vi "main 1.17a beta.vi"() -> ()   [LabVIEW 2015]
uses:
  subvi/PHOIBOS/DEFINITIONS/DEF_dev_state.ctl
  subvi/PHOIBOS/DEFINITIONS/DEF_dev_type.ctl
  <vilib>/Analysis/_algsub.llb/Real Vector Norm.vi
  <vilib>/Analysis/1siggen.llb/Ramp Pattern by Samples.vi
  <vilib>/DAQmx/create/channels.llb/DAQmx Create Channel (DI-Digital Input).vi
  <userlib>/caLab/Private/Put_DBL_PV.vi
  <vilib>/Utility/file.llb/Write Delimited Spreadsheet (string).vi
  <vilib>/Utility/file.llb/Read Delimited Spreadsheet (string).vi
  <userlib>/caLab/Private/Get_PV.vi
  <vilib>/Utility/file.llb/Write Delimited Spreadsheet (DBL).vi
  subvi/Newport ESP301/Newport ESP301.lvlib
  subvi/sp_manip.llb/sp_manip_lib.lvlib
  subvi/sp_manip.llb/tcp_gateway.lvlib
  <vilib>/Analysis/NI_AALBase.lvlib
  <vilib>/Analysis/NI_AALPro.lvlib
  subvi/ZaberTSeries/ZaberTSeries.lvlib
panel:
  out "Pics L":i32=200
  out "Waveform Chart":dbl(graph)
  out "G2 X":cluster{dbl[], "Ramp Pattern":dbl[]}(graph)={array[344 elements], "Ramp Pattern"=[0.0, 0.0, 0.0, 0.0, 0.0, 0.0, 0.0, 0.0, 0.0, 0.0, 0.0, 0.0, 0.0, 0.0, 0.0, 0.0, 0.0, 0.0, 0.0, 0.0, 0.0, 12.377241379310345, 41.64689655172414, 18.335172413793103, 0.0, 0.0, 0.0, 0.0, 0.0, 0.0, 0.0, 0.0, 0.0, 0.0, 0.0, 0.0, 0.0, 0.0, 0.0, 0.0, 0.0, 0.0, 0.0, 0.0, 0.0, 0.0, 0.0, 0.0, 0.0, 0.0, 0.0, 0.0, 0.0, 0.0, 0.0, 0.0, 0.0, 0.0, 0.0, 0.0, 0.0, 0.0, 0.0, 0.0, 0.0, 0.0, 0.0, 0.0, 0.0, 0.0, 0.0, 0.0, 0.0, 0.0, 0.0, 0.0, 0.0, 0.0, 0.0, 0.0, 0.0, 0.0, 0.0, 0.0, 0.0, 0.0, 0.0, 0.0, 0.0, 0.0, 0.0, 0.0, 0.0, 0.0, 0.0, 0.0, 0.0, 0.0, 0.0, 0.0, 0.0, 0.0, 0.0, 0.0, 0.0, 0.0, 0.0, 0.0, 0.0, 0.0, 0.0, 0.0, 0.0, 0.0, 0.0, 17.495517241379314, 48.13413793103449, 27.429999999999996, 0.0, 0.0, 0.0, 0.0, 0.0, 0.0, 0.0, 0.0, 0.0, 0.0, 0.0, 0.0, 0.0, 0.0, 0.0, 0.0, 0.0, 0.0, 0.0, 0.0, 0.0, 0.0, 0.0, 0.0, 0.0, 0.0, 0.0, 0.0, 0.0, 0.0, 0.0, 0.0, 0.0, 0.0, 0.0, 0.0, 0.0, 0.0, 0.0, 0.0, 0.0, 0.0, 0.0, 0.0, 0.0, 0.0, 0.0, 0.0, 0.0, 0.0, 0.0, 0.0, 0.0, 0.0, 0.0, 0.0, 0.0, 0.0, 0.0, 0.0, 0.0, 0.0, 0.0, 0.0, 17.760344827586206, 28.923448275862068, 17.532068965517244, 0.0, 0.0, 0.0, 0.0, 0.0, 0.0, 0.0, 0.0, 0.0, 0.0, 0.0, 0.0, 0.0, 0.0, 0.0, 0.0, 0.0, 0.0, 0.0, 0.0, 0.0, 0.0, 0.0, 0.0, 0.0, 0.0, 0.0, 0.0, 0.0, 0.0, 0.0, 0.0, 0.0, 0.0, 0.0, 0.0, 0.0, 0.0, 0.0, 0.0, 0.0, 0.0, 0.0, 0.0, 0.0, 2.201724137931034, 1.9948275862068956, 0.0, 0.0, 0.0, 0.0, 0.0, 0.0, 0.0, 0.0, 0.0, 0.0, 0.0, 0.0, 0.0, 0.0, 0.0, 0.0, 0.0, 0.0, 0.0, 0.0, 0.0, 0.0, 0.0, 0.0, 0.0, 0.0, 0.0, 0.0, 0.0, 0.0, 0.0, 0.0, 0.0, 0.0, 0.0, 0.0, 0.0, 0.0, 0.0, 0.0, 0.0, 0.0, 0.0, 0.0, 0.0, 0.0, 0.0, 0.0, 0.0, 0.0, 0.0, 0.0, 0.0, 0.0, 0.0, 0.0, 0.0, 0.0, 0.0, 0.0, 0.0, 0.0, 0.0, 0.0, 0.0, 0.0, 0.0, 0.0, 0.0, 0.0, 0.0, 0.0, 0.0, 0.0, 0.0, 0.0, 0.0, 0.0, 0.0, 0.0, 0.0, 0.0, 0.0, 0.0, 0.0, 0.0, 0.0, 0.0, 0.0, 0.0, 0.0, 0.0, 0.0, 0.0, 0.0, 0.0, 0.0, 0.0, 0.0, 0.0, 0.0, 0.0, 0.0, 0.0, 0.0, 0.0, 0.0, 0.0, 0.0, 0.0, 0.0, 0.0]}
  in  "reset every n pics":bool=TRUE
  in  "pics2avg":i32=50
  in  "abort acq.":bool
  out "G2 Y":cluster{dbl[], "Ramp Pattern":dbl[]}(graph)={[0.0, 0.0, 0.0, 0.0, 0.0, 0.0, 0.0, 0.0, 0.0, 0.0, 0.0, 0.0, 0.0, 0.0, 0.0, 0.0, 0.0, 0.0, 0.0, 0.0, 0.0, 0.0, 0.0, 0.0, 0.0, 0.0, 0.0, 0.0, 0.0, 0.0, 0.0, 0.0, 0.0, 0.0, 0.0, 0.0, 0.0, 0.0, 0.0, 0.0, 0.0, 0.0, 0.0, 0.0, 0.0, 0.0, 0.0, 0.0, 0.0, 0.0, 0.0, 0.0, 0.0, 0.0, 0.0, 0.0, 0.0, 0.0, 0.0, 0.0, 0.0, 0.0, 0.0, 0.0, 0.0, 0.0, 0.0, 0.0, 0.0, 0.0, 0.0, 0.0, 0.0, 0.0, 0.0, 0.0, 0.0, 0.0, 0.0, 0.0, 0.0, 0.0, 0.0, 0.0, 0.0, 0.0, 0.0, 0.0, 0.0, 0.0, 0.0, 0.0, 0.0, 0.0, 0.0, 0.0, 0.0, 0.0, 0.0, 0.0, 0.0, 0.0, 0.0, 0.0, 0.0, 0.0, 0.0, 0.0, 0.0, 0.0, 0.0, 0.0, 0.0, 0.0, 0.0, 0.0, 0.0, 0.0, 0.0, 0.0, 0.0, 0.0, 0.0, 0.0, 0.0, 0.0, 0.0, 0.0, 0.0, 0.0, 0.0, 0.0, 0.0, 0.0, 0.0, 0.0, 0.0, 0.0, 0.0, 0.0, 0.0, 0.0, 0.0, 0.0, 0.0, 0.0, 0.0, 0.0, 0.0, 0.0, 0.0, 0.0, 0.0, 0.0, 0.0, 0.0, 0.0, 0.0, 0.0, 0.0, 0.0, 0.0, 0.0, 0.0, 0.0, 0.0, 0.0, 0.0, 0.0, 0.0, 0.0, 0.0, 0.0, 0.0, 0.0, 0.0, 0.0, 0.0, 0.0, 0.0, 0.0, 0.0, 0.0, 0.0, 0.0, 0.0, 0.0, 0.0, 0.0, 0.0, 0.0, 0.0, 0.0, 0.0, 0.0, 0.0, 0.0, 0.0, 0.0, 0.0, 0.0, 0.0, 0.0, 0.0, 0.0, 0.0, 0.0, 0.0, 0.0, 0.0, 0.0, 0.0, 0.0, 0.0, 0.0, 0.0, 0.0, 0.0, 0.0, 0.0, 0.0, 0.0, 0.0, 0.0, 0.0, 0.0, 0.0, 0.0, 0.0, 0.0, 0.0, 0.0, 0.0, 0.0, 0.0, 0.0, 0.0, 0.0, 0.0, 0.0, 0.0, 0.0, 0.0, 0.0, 0.0, 0.0, 0.0, 0.0, 0.0, 0.0, 0.0, 0.0, 0.0, 0.0, 0.0, 0.0], "Ramp Pattern"=[0.0, 1.003921568627451, 2.007843137254902, 3.011764705882353, 4.015686274509804, 5.019607843137255, 6.023529411764706, 7.027450980392157, 8.031372549019608, 9.035294117647059, 10.03921568627451, 11.04313725490196, 12.047058823529412, 13.050980392156863, 14.054901960784314, 15.058823529411764, 16.062745098039215, 17.066666666666666, 18.070588235294117, 19.07450980392157, 20.07843137254902, 21.08235294117647, 22.08627450980392, 23.090196078431372, 24.094117647058823, 25.098039215686274, 26.101960784313725, 27.105882352941176, 28.109803921568627, 29.113725490196078, 30.11764705882353, 31.12156862745098, 32.12549019607843, 33.129411764705885, 34.13333333333333, 35.13725490196079, 36.141176470588235, 37.14509803921569, 38.14901960784314, 39.15294117647059, 40.15686274509804, 41.16078431372549, 42.16470588235294, 43.168627450980395, 44.17254901960784, 45.1764705882353, 46.180392156862744, 47.1843137254902, 48.188235294117646, 49.1921568627451, 50.19607843137255, 51.2, 52.20392156862745, 53.207843137254905, 54.21176470588235, 55.21568627450981, 56.219607843137254, 57.22352941176471, 58.227450980392156, 59.23137254901961, 60.23529411764706, 61.23921568627451, 62.24313725490196, 63.247058823529414, 64.25098039215686, 65.25490196078431, 66.25882352941177, 67.26274509803922, 68.26666666666667, 69.27058823529411, 70.27450980392157, 71.27843137254902, 72.28235294117647, 73.28627450980392, 74.29019607843138, 75.29411764705883, 76.29803921568627, 77.30196078431372, 78.30588235294118, 79.30980392156863, 80.31372549019608, 81.31764705882352, 82.32156862745099, 83.32549019607843, 84.32941176470588, 85.33333333333333, 86.33725490196079, 87.34117647058824, 88.34509803921569, 89.34901960784313, 90.3529411764706, 91.35686274509804, 92.36078431372549, 93.36470588235294, 94.3686274509804, 95.37254901960785, 96.37647058823529, 97.38039215686274, 98.3843137254902, 99.38823529411765, 100.3921568627451, 101.39607843137254, 102.4, 103.40392156862745, 104.4078431372549, 105.41176470588235, 106.41568627450981, 107.41960784313726, 108.4235294117647, 109.42745098039215, 110.43137254901961, 111.43529411764706, 112.43921568627451, 113.44313725490196, 114.44705882352942, 115.45098039215686, 116.45490196078431, 117.45882352941176, 118.46274509803922, 119.46666666666667, 120.47058823529412, 121.47450980392156, 122.47843137254903, 123.48235294117647, 124.48627450980392, 125.49019607843137, 126.49411764705883, 127.49803921568628, 128.50196078431372, 129.50588235294117, 130.50980392156862, 131.51372549019607, 132.51764705882354, 133.521568627451, 134.52549019607844, 135.52941176470588, 136.53333333333333, 137.53725490196078, 138.54117647058823, 139.54509803921567, 140.54901960784315, 141.5529411764706, 142.55686274509804, 143.5607843137255, 144.56470588235294, 145.5686274509804, 146.57254901960783, 147.57647058823528, 148.58039215686276, 149.5843137254902, 150.58823529411765, 151.5921568627451, 152.59607843137255, 153.6, 154.60392156862744, 155.6078431372549, 156.61176470588236, 157.6156862745098, 158.61960784313726, 159.6235294117647, 160.62745098039215, 161.6313725490196, 162.63529411764705, 163.6392156862745, 164.64313725490197, 165.64705882352942, 166.65098039215687, 167.65490196078431, 168.65882352941176, 169.6627450980392, 170.66666666666666, 171.6705882352941, 172.67450980392158, 173.67843137254903, 174.68235294117648, 175.68627450980392, 176.69019607843137, 177.69411764705882, 178.69803921568626, 179.7019607843137, 180.7058823529412, 181.70980392156864, 182.71372549019608, 183.71764705882353, 184.72156862745098, 185.72549019607843, 186.72941176470587, 187.73333333333332, 188.7372549019608, 189.74117647058824, 190.7450980392157, 191.74901960784314, 192.75294117647059, 193.75686274509803, 194.76078431372548, 195.76470588235293, 196.7686274509804, 197.77254901960785, 198.7764705882353, 199.78039215686275, 200.7843137254902, 201.78823529411764, 202.7921568627451, 203.79607843137254, 204.8, 205.80392156862746, 206.8078431372549, 207.81176470588235, 208.8156862745098, 209.81960784313725, 210.8235294117647, 211.82745098039214, 212.83137254901962, 213.83529411764707, 214.8392156862745, 215.84313725490196, 216.8470588235294, 217.85098039215686, 218.8549019607843, 219.85882352941175, 220.86274509803923, 221.86666666666667, 222.87058823529412, 223.87450980392157, 224.87843137254902, 225.88235294117646, 226.8862745098039, 227.89019607843136, 228.89411764705883, 229.89803921568628, 230.90196078431373, 231.90588235294118, 232.90980392156862, 233.91372549019607, 234.91764705882352, 235.92156862745097, 236.92549019607844, 237.9294117647059, 238.93333333333334, 239.93725490196078, 240.94117647058823, 241.94509803921568, 242.94901960784313, 243.95294117647057, 244.95686274509805, 245.9607843137255, 246.96470588235294, 247.9686274509804, 248.97254901960784, 249.9764705882353, 250.98039215686273, 251.98431372549018, 252.98823529411766, 253.9921568627451, 254.99607843137255, 256.0]}
  out "ETA":timestamp=timestamp(3655133644.4615793 s since 1904-01-01) format="%<%H:%M:%S>T"
  out "acq. imgs":i32=200
  out "snap_prog":dbl(slide)=1.0 scale=0.0..1.0
  in  "BasePath":path=path "T:/trARPES/PESData"
  in  "cam_liveavg":bool=TRUE caption="live average"
  out "cam_fps":dbl=19.690658487387566 caption="FPS" format="%.1g"
  out "sideimg":dbl[][](graph)
  out "RunNumber":u16=3091
  out "sum":dbl format="%#.2g"
  out "max":dbl=22.774482758620692
  out "mainimg":dbl[][](graph)
  out "ESP_con?":bool=TRUE caption="ESP301"
  out "phoib_con?":bool caption="PHOIBOS"
  out "manip_con?":bool=TRUE caption="manipulator"
  out "cam_con?":bool caption="camera"
  in  "main_close":bool=TRUE
  in  "Tab Control":enum32{"live", "scan", "devices"}(tab)=enum."devices"
  in  "wattpilot_set":bool
  out "Readback_wattpilot":dbl=304.89
  in  "Set Powet (%)":dbl
  out "Readback":dbl=340.0
  out "In Range":bool
  in  "setpoint_set":bool
  in  "Setpoint":dbl=302.0
  out "TB":dbl=304.91
  out "TA":dbl=304.49
  in  "phoib_I_10s":dbl
  out "phoib_I_10":dbl caption="Mesh Back"
  in  "mirr_go":bool
  in  "ESP_opent0file":bool
  in  "mirr_rel":i32=1 caption="relative [steps]"
  in  "mirr_Y-":bool
  in  "mirr_Y+":bool
  in  "mirr_X+":bool
  in  "mirr_X-":bool
  in  "manip_deltas":dbl[](array[numeric])=[0.0, 0.0, 5.0, 0.0, 0.0, 0.0] caption="delta" format="%#.5g"
  in  "aq.mode":enum32{"Radio Selection 1", "Radio Selection 2"}(radio)=enum."Radio Selection 2"
  in  "dark avg":i32=100
  in  "cam_avgs":i32=20 caption="N"
  in  "ESP_delta":dbl caption="relative [mm]"
  in  "ESP_-":bool
  in  "ESP_+":bool
  in  "ESP_go":bool
  in  "ESP_dest_t":dbl=728236.1319443199 caption="[fs]"
  in  "ESP_dest":dbl=-35.84015 caption="[mm]"
  in  "ESP_set_t0":bool
  in  "phoib_I_6s":dbl=3200.0
  in  "phoib_I_5s":dbl=1500.0
  in  "phoib_I_4s":dbl=4.558
  in  "phoib_I_3s":dbl=-10.0
  in  "phoib_I_2s":dbl=35.0
  in  "phoib_I_1s":dbl=21.0
  in  "phoib_standby":bool
  in  "phoib_set":bool
  out "phoib_I_6":dbl=3200.0 caption="Screen Voltage"
  out "phoib_I_5":dbl=1500.0 caption="Detctor Voltage"
  out "phoib_I_4":dbl=4.558 caption="Work Function"
  out "phoib_I_3":dbl=-10.0 caption="Coil Current"
  out "phoib_I_2":dbl=35.0 caption="Pass Energy"
  out "phoib_I_1":dbl=21.0 caption="Kinetic Energy"
  out "Saved Positions":string[][](table)=[["ertwertwert", "-2.299945", "-2.030214", "38.900024", "50.000762", "0.000887", "-97.998082"], ["uztgugt", "-14.999451", "-13.638894", "442.380066", "13.998380", "-1.893758", "-76.305838"], ["asdf", "-14.999451", "-13.638894", "442.380066", "13.998380", "-1.893758", "-76.305838"], ["test3", "-14.999451", "-13.638894", "441.380066", "13.998380", "-1.893758", "-76.305838"]]
  in  "Save Pos":bool
  in  "Load":bool
  in  "Delete":bool
  in  "ManipRel +":bool
  in  "ManipRel -":bool
  in  "Move Abs":bool
  in  "stop manip":bool
  in  "dest":dbl[](array[numeric])=[1.794011231344732, -4.007411134769244, 35.099853515625, 337.9843004481455, 2.0, 140.61656469713384] caption="destination" format="%#.5g"
  out "axis":string[](array[string])=["x", "y", "z", "polar", "tilt", "azimut"]
  out "pos":dbl[](array[numeric])=[1.794011231344732, -4.007411134769244, 35.099853515625, 337.9843004481455, 1.998632949125299, 140.61656469713384] caption="position" format="%.5f"
  in  "ana_mode":T1(ring)=enum."WideAngleMode"
  in  "ana_voltrange":enum16{"3.5kV", "1.5kV", "400V", "100V", "10V"}(ring)=enum."400V"
  out "ESP_pos":dbl=-35.84015 caption="Position"
  out "ESP_delay":dbl=-0.3335640952092252 caption="Delay"
  out "ESP_t0":dbl=-35.8401 caption="Time Zero @"
  out "phoib_I_7":dbl=-30.0 caption="Conversion Voltage"
  in  "phoib_I_7s":dbl=-30.0
  in  "phoib_I_8s":dbl=0.0039
  in  "phoib_I_9s":dbl
  out "phoib_I_8":dbl=0.0039 caption="FD1"
  out "phoib_I_9":dbl caption="Mesh Front"
  in  "gain":bool
  in  "cam_exp":u32=50 caption="exposure [ms]"
  in  "binning":u16(ring)=2 items=["X 1", "X 2", "X 4", "X 8"]
  in  "cam_dark?":bool=TRUE caption="subtract dark?"
  in  "cam_dark":bool
  in  "cam_saveimg":bool
  in  "e-size":u8
  in  "lower threshold":i32=50
  in  "count?":bool
  in  "ROI Left":i32=1
  in  "ROI Right":i32=43
  in  "ROI Top":i32=1
  in  "ROI Bottom":i32=33
  out "moving?":bool[](array[boolean])
  out "mirr_posX":i32=1955 caption="X"
  out "mirr_posY":i32=2950 caption="Y"
  in  "mirr_dest":i32[](array[numeric])=[60782, 121383]
  out "waveplate position":dbl format="%.6g"
  out "stage2 position":dbl format="%.6g"
  out "current scan 2":i32=3
  out "scan 1":dbl(slide)=1.0 scale=0.0..1.0
  in  "Tab Control 2":enum32{"setup", "data"}(tab)
  in  "scan_selector 2":T2(tab)
  in  "scan_manip_start 2":dbl[](array[numeric])=[1.794011231344732, -4.007411134769244, 35.099853515625, 337.9843004481455, 2.000390761745462, 140.61656469713384] caption="start position" format="%#.5g"
  in  "scan_manip_deltas 2":dbl[](array[numeric])=[0.0, 0.0, 0.0, 0.0, 1.0, 0.0] caption="direction vector\n(gets normalized)" format="%#.5g"
  in  "scan_manip_setstart 2":bool
  in  "scan_mirr_start 2":i32[](array[numeric])=[60782, 121383] caption="scan_mirr_start"
  in  "scan_mirr_deltas 2":i32[](array[numeric])=[1, 0] caption="direction vector\n(gets normalized)"
  in  "scan_mirr_setstart 2":bool
  in  "wait addional  2":dbl caption="s"
  in  "Wait for T 2":bool=TRUE
  in  "scan_volt_parameter 2":string(combo)="Kinetic Energy"
  in  "waypointsD2":string[][](table)
  in  "waypointsD1":string[][](table)=[["302", "1"], ["304", ""], ["", ""]]
  in  "load waypoints 1":bool
  in  "meas_iter":i32=1 caption="Iterations"
  in  "scan_selector":T2(tab)=enum."delay"
  in  "scan_manip_setstart":bool
  in  "scan_manip_start":dbl[](array[numeric])=[1.794011231344732, -4.007411134769244, 35.099853515625, 337.9843004481455, 2.000390761745462, 140.61656469713384] caption="start position" format="%#.5g"
  in  "scan_manip_deltas":dbl[](array[numeric])=[0.0, 0.0, 0.0, 0.0, 1.0, 0.0] caption="direction vector\n(gets normalized)" format="%#.5g"
  in  "scan_mirr_start":i32[](array[numeric])=[60782, 121383]
  in  "scan_mirr_deltas":i32[](array[numeric])=[1, 0] caption="direction vector\n(gets normalized)"
  in  "scan_mirr_setstart":bool
  in  "wait addional":dbl caption="s"
  in  "Wait for T":bool=TRUE
  in  "scan_volt_parameter":string(combo)="Kinetic Energy"
  in  "clear waypoints 1":bool
  in  "load waypoints 2":bool
  in  "clear waypoints 2":bool
  out "intensitygraph":cluster{"Array":dbl[], "Intensity Chart":dbl[]}(graph)={"Array"=[302.0, 303.0, 304.0], "Intensity Chart"=[1937.88, 12704.590000000002, 4640.840000000001]}
  out "energygraph":dbl[][](graph)=[[0.0, 0.0, 0.0, 64.28999999999999, 120.06, 0.0, 0.0, 0.0, 0.0, 0.0, 0.0, 0.0, 0.0, 0.0, 0.0, 0.0, 0.0, 0.0, 0.0, 0.0, 0.0, 0.0, 0.0, 0.0, 0.0, 0.0, 0.0, 0.0, 0.0, 0.0, 0.0, 0.0, 0.0, 0.0, 0.0, 0.0, 0.0, 0.0, 0.0, 0.0, 0.0, 0.0, 0.0, 0.0, 0.0, 0.0, 0.0, 0.0, 0.0, 384.53999999999996, 1103.3799999999999, 448.21000000000004, 0.0, 0.0, 0.0, 0.0, 0.0, 0.0, 0.0, 0.0, 0.0, 0.0, 0.0, 0.0, 0.0, 0.0, 0.0, 0.0, 0.0, 120.82, 0.0, 261.04, 195.1, 253.87, 199.70999999999998, 127.75, 87.50999999999999, 0.0, 52.54, 0.0, 0.0, 51.78, 55.73, 0.0, 0.0, 0.0, 0.0, 0.0, 0.0, 0.0, 0.0, 0.0, 0.0, 0.0, 0.0, 0.0, 0.0, 0.0, 0.0, 0.0, 0.0, 0.0, 0.0, 0.0, 0.0, 0.0, 0.0, 0.0, 0.0, 0.0, 0.0, 0.0, 0.0, 332.90999999999997, 1106.25, 934.74, 0.0, 156.76, 62.65, 0.0, 0.0, 0.0, 0.0, 0.0, 0.0, 54.62, 0.0, 0.0, 0.0, 0.0, 0.0, 0.0, 0.0, 0.0, 0.0, 0.0, 0.0, 0.0, 0.0, 0.0, 0.0, 0.0, 0.0, 0.0, 65.85, 165.75, 0.0, 0.0, 0.0, 0.0, 0.0, 0.0, 0.0, 0.0, 0.0, 0.0, 0.0, 0.0, 0.0, 0.0, 0.0, 0.0, 0.0, 266.63, 591.5, 261.64, 0.0, 391.9, 527.29, 82.87, 123.75, 286.74, 151.72, 0.0, 0.0, 0.0, 0.0, 0.0, 0.0, 0.0, 0.0, 0.0, 0.0, 0.0, 0.0, 0.0, 0.0, 0.0, 0.0, 0.0, 0.0, 0.0, 396.37, 721.0900000000001, 353.5, 83.97999999999999, 104.77000000000001, 0.0, 57.83, 60.98, 182.28, 128.78, 0.0, 0.0, 0.0, 465.25, 624.3399999999999, 348.62, 0.0, 0.0, 0.0, 0.0, 0.0, 0.0, 0.0, 0.0, 0.0, 0.0, 0.0, 0.0, 119.7, 217.91, 120.56, 0.0, 0.0, 0.0, 0.0, 0.0, 0.0, 0.0, 58.89, 0.0, 0.0, 0.0, 202.23999999999998, 149.79000000000002, 0.0, 117.82, 212.51999999999998, 534.74, 421.98, 50.97, 0.0, 0.0, 0.0, 0.0, 362.15999999999997, 656.04, 265.02, 0.0, 0.0, 0.0, 0.0, 0.0, 0.0, 0.0, 0.0, 0.0, 0.0, 0.0, 0.0, 0.0, 0.0, 0.0, 0.0, 0.0, 0.0, 0.0, 0.0, 0.0, 0.0, 0.0, 0.0, 0.0, 0.0, 0.0, 0.0, 0.0, 0.0, 0.0, 0.0, 0.0, 0.0, 0.0, 0.0, 0.0, 0.0, 0.0, 0.0, 0.0, 0.0, 0.0, 0.0, 0.0, 0.0, 0.0, 0.0, 0.0, 0.0, 0.0, 0.0, 0.0, 0.0, 0.0, 0.0, 0.0, 0.0, 0.0, 0.0, 0.0, 0.0, 0.0, 0.0, 237.67999999999998, 286.08, 130.9, 0.0, 0.0, 0.0, 0.0, 0.0, 0.0, 0.0, 0.0, 0.0, 0.0, 0.0, 0.0, 0.0, 0.0, 0.0, 0.0, 0.0, 0.0, 0.0, 0.0, 0.0, 0.0, 0.0, 0.0, 0.0, 0.0, 0.0, 0.0], [0.0, 0.0, 0.0, 0.0, 0.0, 0.0, 0.0, 0.0, 0.0, 0.0, 0.0, 0.0, 0.0, 0.0, 0.0, 0.0, 0.0, 485.13, 1279.2, 234.71, 0.0, 0.0, 0.0, 0.0, 0.0, 0.0, 0.0, 0.0, 0.0, 0.0, 0.0, 0.0, 50.5, 654.4200000000001, 511.98, 0.0, 0.0, 0.0, 0.0, 0.0, 0.0, 0.0, 0.0, 0.0, 0.0, 0.0, 0.0, 0.0, 0.0, 0.0, 0.0, 0.0, 0.0, 0.0, 0.0, 0.0, 0.0, 0.0, 63.72, 693.84, 574.54, 0.0, 0.0, 0.0, 68.68, 1054.28, 1010.9499999999999, 0.0, 0.0, 0.0, 0.0, 0.0, 0.0, 0.0, 0.0, 0.0, 0.0, 0.0, 56.57, 971.76, 1333.73, 330.0, 0.0, 0.0, 0.0, 0.0, 0.0, 349.33000000000004, 292.7, 0.0, 0.0, 0.0, 0.0, 0.0, 0.0, 82.77000000000001, 1059.23, 1069.87, 156.47, 0.0, 0.0, 0.0, 0.0, 293.91, 333.47, 551.4, 493.64, 73.72999999999999, 0.0, 0.0, 0.0, 0.0, 0.0, 0.0, 0.0, 0.0, 0.0, 0.0, 0.0, 0.0, 0.0, 0.0, 286.01, 543.0699999999999, 251.94, 0.0, 0.0, 0.0, 0.0, 0.0, 233.63, 968.4799999999999, 771.53, 109.94, 0.0, 123.07, 499.72999999999996, 431.4, 0.0, 0.0, 60.85, 69.5, 0.0, 0.0, 0.0, 0.0, 0.0, 0.0, 0.0, 0.0, 0.0, 0.0, 0.0, 0.0, 0.0, 0.0, 52.01, 0.0, 0.0, 0.0, 0.0, 0.0, 0.0, 0.0, 0.0, 0.0, 0.0, 0.0, 0.0, 0.0, 0.0, 0.0, 0.0, 0.0, 0.0, 0.0, 0.0, 0.0, 0.0, 0.0, 0.0, 0.0, 0.0, 0.0, 0.0, 0.0, 0.0, 0.0, 0.0, 0.0, 52.95, 478.8, 870.47, 572.83, 61.67, 268.19, 1143.4, 1804.2599999999998, 1145.6100000000001, 739.22, 904.59, 1109.3000000000002, 1233.6599999999999, 212.92, 0.0, 0.0, 105.95, 448.76000000000005, 1306.3500000000001, 1005.5900000000001, 68.8, 0.0, 57.94, 0.0, 0.0, 0.0, 0.0, 0.0, 0.0, 0.0, 0.0, 0.0, 0.0, 0.0, 0.0, 0.0, 0.0, 0.0, 0.0, 0.0, 0.0, 0.0, 0.0, 0.0, 0.0, 0.0, 0.0, 159.01, 520.94, 925.5600000000001, 1641.53, 2261.26, 1259.83, 0.0, 0.0, 0.0, 0.0, 0.0, 0.0, 136.69, 398.81, 382.02, 0.0, 0.0, 0.0, 0.0, 0.0, 0.0, 421.01, 1376.5800000000002, 1425.75, 268.07, 0.0, 345.84000000000003, 396.77, 0.0, 0.0, 0.0, 0.0, 0.0, 216.93, 727.65, 830.9, 774.2299999999999, 839.3900000000001, 309.97, 0.0, 0.0, 0.0, 0.0, 0.0, 0.0, 0.0, 100.57, 459.66, 305.86, 0.0, 0.0, 0.0, 0.0, 0.0, 0.0, 0.0, 0.0, 0.0, 0.0, 0.0, 0.0, 0.0, 0.0, 0.0, 0.0, 0.0, 0.0, 0.0, 0.0, 0.0, 0.0, 0.0, 0.0, 0.0, 64.97999999999999, 379.62, 337.15999999999997, 83.6, 463.66, 399.03999999999996, 0.0, 0.0, 0.0, 0.0, 0.0, 0.0, 0.0, 0.0, 0.0, 0.0, 0.0, 0.0, 0.0, 0.0, 0.0, 0.0, 0.0, 0.0, 0.0, 0.0, 0.0, 0.0, 0.0, 0.0, 0.0, 0.0, 0.0], [0.0, 0.0, 0.0, 0.0, 0.0, 0.0, 0.0, 0.0, 0.0, 0.0, 0.0, 0.0, 0.0, 0.0, 0.0, 165.83, 124.99, 78.27000000000001, 0.0, 0.0, 0.0, 765.77, 1457.88, 293.67, 0.0, 0.0, 0.0, 0.0, 0.0, 0.0, 0.0, 0.0, 0.0, 0.0, 0.0, 0.0, 0.0, 0.0, 0.0, 0.0, 0.0, 0.0, 0.0, 0.0, 0.0, 0.0, 0.0, 0.0, 0.0, 85.5, 116.32, 0.0, 0.0, 0.0, 0.0, 0.0, 0.0, 0.0, 0.0, 0.0, 0.0, 0.0, 0.0, 0.0, 0.0, 0.0, 0.0, 0.0, 179.01, 123.78999999999999, 64.69, 0.0, 433.57000000000005, 1457.15, 661.49, 0.0, 0.0, 0.0, 0.0, 0.0, 0.0, 171.38, 497.28999999999996, 835.47, 1797.0300000000002, 1202.25, 169.95, 0.0, 0.0, 0.0, 0.0, 383.74, 496.08, 196.89999999999998, 0.0, 0.0, 0.0, 0.0, 719.08, 1717.5100000000002, 1360.8, 163.65, 118.56, 798.75, 610.32, 0.0, 0.0, 0.0, 0.0, 73.12, 51.75, 0.0, 0.0, 0.0, 0.0, 0.0, 0.0, 0.0, 0.0, 0.0, 0.0, 0.0, 233.35000000000002, 1128.3, 1138.8400000000001, 207.43, 0.0, 0.0, 50.52, 0.0, 0.0, 0.0, 0.0, 0.0, 0.0, 0.0, 0.0, 0.0, 0.0, 0.0, 0.0, 0.0, 0.0, 0.0, 0.0, 0.0, 0.0, 0.0, 0.0, 0.0, 0.0, 122.82, 66.93, 184.87, 606.35, 1065.2, 616.33, 82.97, 0.0, 0.0, 0.0, 0.0, 0.0, 0.0, 0.0, 0.0, 0.0, 0.0, 0.0, 210.77, 369.49, 0.0, 0.0, 0.0, 0.0, 0.0, 0.0, 0.0, 0.0, 0.0, 0.0, 0.0, 0.0, 0.0, 0.0, 0.0, 0.0, 0.0, 0.0, 61.71, 492.70000000000005, 501.67999999999995, 50.9, 0.0, 0.0, 0.0, 0.0, 0.0, 0.0, 0.0, 0.0, 0.0, 0.0, 0.0, 0.0, 0.0, 0.0, 0.0, 0.0, 0.0, 0.0, 0.0, 0.0, 0.0, 0.0, 0.0, 0.0, 0.0, 0.0, 0.0, 0.0, 0.0, 0.0, 0.0, 0.0, 0.0, 0.0, 0.0, 0.0, 0.0, 0.0, 0.0, 0.0, 0.0, 0.0, 0.0, 0.0, 0.0, 0.0, 0.0, 0.0, 0.0, 0.0, 0.0, 0.0, 0.0, 0.0, 0.0, 0.0, 0.0, 0.0, 0.0, 0.0, 0.0, 0.0, 0.0, 0.0, 0.0, 0.0, 0.0, 0.0, 0.0, 0.0, 0.0, 0.0, 0.0, 0.0, 0.0, 0.0, 0.0, 191.69, 347.02, 262.31, 325.89, 168.79, 0.0, 0.0, 52.9, 53.13, 0.0, 0.0, 0.0, 0.0, 0.0, 0.0, 0.0, 0.0, 0.0, 0.0, 0.0, 0.0, 0.0, 0.0, 0.0, 0.0, 0.0, 0.0, 0.0, 0.0, 0.0, 0.0, 0.0, 0.0, 0.0, 0.0, 327.12, 491.83000000000004, 242.02999999999997, 0.0, 0.0, 0.0, 0.0, 0.0, 0.0, 0.0, 676.6, 975.77, 229.86, 0.0, 144.15, 151.75, 0.0, 0.0, 0.0, 0.0, 0.0, 0.0, 0.0, 0.0, 0.0, 0.0, 0.0, 0.0, 0.0, 0.0, 0.0, 0.0, 0.0, 0.0, 0.0, 0.0, 0.0, 0.0, 0.0]]
  out "anglegraph":dbl[][](graph)=[[0.0, 0.0, 0.0, 0.0, 0.0, 0.0, 0.0, 0.0, 0.0, 0.0, 0.0, 0.0, 0.0, 0.0, 0.0, 0.0, 0.0, 0.0, 0.0, 0.0, 0.0, 0.0, 0.0, 0.0, 0.0, 0.0, 0.0, 307.98, 204.45, 0.0, 0.0, 0.0, 0.0, 0.0, 0.0, 0.0, 0.0, 0.0, 0.0, 0.0, 0.0, 0.0, 0.0, 0.0, 0.0, 0.0, 0.0, 0.0, 0.0, 0.0, 0.0, 0.0, 0.0, 0.0, 0.0, 0.0, 0.0, 0.0, 0.0, 0.0, 0.0, 0.0, 0.0, 0.0, 0.0, 0.0, 0.0, 0.0, 0.0, 0.0, 0.0, 0.0, 0.0, 0.0, 0.0, 0.0, 0.0, 0.0, 0.0, 0.0, 0.0, 0.0, 0.0, 0.0, 0.0, 0.0, 0.0, 0.0, 0.0, 0.0, 0.0, 0.0, 0.0, 0.0, 0.0, 0.0, 0.0, 0.0, 0.0, 0.0, 0.0, 0.0, 0.0, 0.0, 0.0, 0.0, 0.0, 0.0, 0.0, 0.0, 0.0, 0.0, 0.0, 0.0, 0.0, 0.0, 0.0, 0.0, 0.0, 0.0, 0.0, 0.0, 0.0, 0.0, 0.0, 0.0, 0.0, 0.0, 0.0, 0.0, 0.0, 0.0, 0.0, 0.0, 0.0, 0.0, 0.0, 0.0, 0.0, 0.0, 0.0, 0.0, 0.0, 0.0, 0.0, 0.0, 0.0, 0.0, 0.0, 0.0, 0.0, 0.0, 0.0, 0.0, 0.0, 0.0, 640.8800000000001, 550.45, 91.89, 0.0, 0.0, 0.0, 0.0, 0.0, 0.0, 0.0, 0.0, 0.0, 0.0, 0.0, 0.0, 0.0, 0.0, 0.0, 0.0, 69.94, 60.96, 0.0, 0.0, 0.0, 0.0, 0.0, 0.0, 0.0, 0.0, 0.0, 0.0, 0.0, 0.0, 0.0, 0.0, 0.0, 0.0, 0.0, 0.0, 0.0, 115.87, 235.84, 172.04999999999998, 0.0, 0.0, 0.0, 0.0, 0.0, 0.0, 0.0, 0.0, 0.0, 0.0, 0.0, 0.0, 0.0, 0.0, 0.0, 0.0, 0.0, 0.0, 0.0, 0.0, 0.0, 0.0, 0.0, 0.0, 0.0, 0.0, 0.0, 0.0, 0.0, 0.0, 0.0, 0.0, 0.0, 0.0, 0.0, 0.0, 0.0, 0.0, 0.0, 0.0, 0.0, 0.0, 0.0, 0.0, 0.0, 0.0, 0.0, 0.0, 0.0, 0.0, 0.0, 0.0, 0.0, 0.0, 0.0, 0.0, 0.0], [0.0, 0.0, 0.0, 0.0, 0.0, 0.0, 0.0, 0.0, 0.0, 0.0, 0.0, 0.0, 0.0, 0.0, 0.0, 0.0, 54.97, 1426.6399999999999, 1312.94, 180.81, 0.0, 0.0, 0.0, 0.0, 0.0, 0.0, 0.0, 465.48, 989.61, 293.56, 0.0, 0.0, 0.0, 0.0, 0.0, 0.0, 0.0, 0.0, 0.0, 0.0, 0.0, 0.0, 0.0, 0.0, 0.0, 0.0, 0.0, 0.0, 0.0, 0.0, 0.0, 0.0, 0.0, 0.0, 0.0, 0.0, 0.0, 0.0, 0.0, 331.78, 944.91, 463.28, 0.0, 0.0, 0.0, 0.0, 143.70999999999998, 402.81, 196.09, 0.0, 0.0, 0.0, 483.82, 433.7, 0.0, 0.0, 0.0, 0.0, 0.0, 0.0, 89.85, 513.2, 263.03999999999996, 0.0, 0.0, 0.0, 0.0, 0.0, 0.0, 0.0, 0.0, 104.84, 0.0, 226.86, 214.93, 235.13, 0.0, 0.0, 0.0, 0.0, 0.0, 0.0, 0.0, 0.0, 0.0, 0.0, 0.0, 0.0, 0.0, 0.0, 0.0, 0.0, 0.0, 0.0, 0.0, 0.0, 0.0, 0.0, 0.0, 0.0, 0.0, 0.0, 0.0, 0.0, 0.0, 0.0, 0.0, 0.0, 0.0, 0.0, 0.0, 0.0, 0.0, 0.0, 0.0, 0.0, 0.0, 0.0, 0.0, 380.83, 649.96, 229.04, 0.0, 0.0, 0.0, 276.21000000000004, 441.79999999999995, 228.29, 0.0, 0.0, 0.0, 0.0, 0.0, 0.0, 0.0, 0.0, 0.0, 0.0, 0.0, 0.0, 0.0, 0.0, 0.0, 0.0, 0.0, 0.0, 0.0, 0.0, 123.92000000000002, 1311.81, 1454.81, 600.87, 0.0, 0.0, 0.0, 0.0, 0.0, 0.0, 0.0, 0.0, 0.0, 0.0, 0.0, 0.0, 0.0, 0.0, 0.0, 0.0, 0.0, 0.0, 0.0, 0.0, 0.0, 0.0, 0.0, 0.0, 0.0, 0.0, 0.0, 0.0, 0.0, 0.0, 654.53, 894.22, 410.35, 0.0, 0.0, 0.0, 0.0, 0.0, 0.0, 0.0, 0.0, 0.0, 0.0, 0.0, 0.0, 0.0, 0.0, 0.0, 0.0, 0.0, 0.0, 0.0, 0.0, 0.0, 0.0, 0.0, 0.0, 0.0, 0.0, 0.0, 0.0, 0.0, 0.0, 0.0, 0.0, 0.0, 0.0, 0.0, 0.0, 0.0, 0.0, 0.0, 0.0, 0.0, 0.0, 0.0, 0.0, 0.0, 0.0, 0.0, 0.0, 0.0, 0.0, 0.0], [0.0, 0.0, 0.0, 0.0, 0.0, 0.0, 0.0, 0.0, 0.0, 0.0, 0.0, 0.0, 0.0, 0.0, 0.0, 0.0, 0.0, 0.0, 0.0, 0.0, 0.0, 0.0, 0.0, 0.0, 0.0, 0.0, 0.0, 0.0, 0.0, 125.9, 1017.51, 504.48, 0.0, 0.0, 0.0, 0.0, 0.0, 0.0, 0.0, 0.0, 0.0, 0.0, 0.0, 0.0, 0.0, 0.0, 0.0, 0.0, 0.0, 0.0, 0.0, 0.0, 0.0, 0.0, 0.0, 0.0, 0.0, 0.0, 0.0, 0.0, 0.0, 0.0, 0.0, 0.0, 0.0, 0.0, 0.0, 0.0, 0.0, 0.0, 0.0, 0.0, 109.81, 66.88, 0.0, 0.0, 733.48, 806.32, 342.43, 0.0, 0.0, 0.0, 0.0, 0.0, 0.0, 0.0, 0.0, 0.0, 0.0, 0.0, 0.0, 0.0, 0.0, 0.0, 0.0, 0.0, 0.0, 0.0, 0.0, 0.0, 0.0, 0.0, 0.0, 0.0, 0.0, 174.07999999999998, 275.74, 429.21, 301.15999999999997, 0.0, 0.0, 0.0, 0.0, 0.0, 0.0, 0.0, 0.0, 0.0, 0.0, 0.0, 0.0, 0.0, 0.0, 0.0, 0.0, 0.0, 0.0, 0.0, 0.0, 0.0, 0.0, 0.0, 0.0, 0.0, 0.0, 0.0, 0.0, 0.0, 0.0, 0.0, 0.0, 0.0, 0.0, 0.0, 0.0, 0.0, 0.0, 0.0, 0.0, 0.0, 0.0, 0.0, 0.0, 0.0, 0.0, 0.0, 0.0, 0.0, 0.0, 0.0, 0.0, 0.0, 0.0, 0.0, 0.0, 0.0, 0.0, 0.0, 0.0, 0.0, 0.0, 0.0, 0.0, 0.0, 0.0, 252.98000000000002, 303.56, 60.91, 52.9, 53.13, 0.0, 0.0, 0.0, 0.0, 0.0, 0.0, 0.0, 0.0, 0.0, 0.0, 0.0, 0.0, 0.0, 0.0, 0.0, 0.0, 0.0, 0.0, 0.0, 0.0, 0.0, 0.0, 0.0, 0.0, 0.0, 0.0, 0.0, 0.0, 0.0, 0.0, 0.0, 0.0, 0.0, 61.05, 350.49, 266.71000000000004, 0.0, 0.0, 0.0, 0.0, 0.0, 0.0, 0.0, 0.0, 0.0, 0.0, 0.0, 0.0, 0.0, 0.0, 0.0, 0.0, 0.0, 0.0, 0.0, 0.0, 0.0, 0.0, 0.0, 0.0, 0.0, 0.0, 0.0, 0.0, 0.0, 0.0, 0.0, 0.0, 0.0, 0.0, 0.0, 0.0, 0.0, 0.0, 0.0, 0.0]]
  in  "stop after iteration":bool
  in  "time/step [s]":dbl=10.787117004394531
  out "current iteration":i32=1
  out "current scan":i32=3
  out "iteration":dbl(slide)=1.0 scale=0.0..1.0
  out "scan 2":dbl(slide)=1.0 scale=0.0..1.0
  in  "stop after step":bool
  in  "scan_go":bool
  out "measpoints":i32=3
  out "total steps":i32=3
  out "RAM [MB]":dbl=1.6590000000000003
  out "disk [MB]":dbl=1.6590000000000003
  out "duration [HH:MM:SS]":dbl=32.361351013183594 format="%<%H:%M:%S>t"
  out "ETA 2":timestamp
  in  "WattPilot EPICS chanel readback":string="trARPES:Wattpilot:PumpPercent_RBV"
  in  "WattPilot EPICS chanel set":string="trARPES:Wattpilot:PumpPercent"
  in  "ESP patch":i32[](array[numeric])=[3, 2, 1]
  in  "LS310  EPICS Heater":string="trARPES:Carving:HT-RNG"
  in  "LS310  EPICS SP":string="trARPES:Carving:TEMP"
  in  "LS310  EPICS chanel B":string="trARPES:Carving:TEMP-B"
  in  "mm/s":dbl
  in  "Set Speed to":bool
  in  "ESP Axis waveplate":i32=2 min=1 max=3
  in  "mirr_init":bool
  in  "mirr_release":bool
  in  "mirr_Y#":u8=2
  in  "manip_init":bool
  in  "manip_release":bool
  in  "phoib_init":bool
  in  "phoib_release":bool
  in  "ESP_init":bool
  in  "ESP_release":bool
  in  "ESP301 VISA":refnum<visa-resource-name>="COM4"
  in  "board number":i32
  in  "cam_init":bool
  in  "cam_release":bool
  out "cam_error":errorcluster
  out "phoib_error":errorcluster
  out "state":T3=1 items=["Off"=-1, "Standby"=0, "On"=1]
  in  "ESP Axis delay":i32=3 min=1 max=3
  out "error out":errorcluster={"status"=FALSE, "code"=1073676418, "source"="VISA Close in Newport ESP301.lvlib:Close.vi->main 1.17a beta.vi"}
  out "error out 2":errorcluster={"status"=TRUE, "code"=1, "source"="TCP Write in sp_manip_lib.lvlib:sp_manip_disconnect.vi->main 1.17a beta.vi"}
  out "mirr_Error":errorcluster={"status"=FALSE, "code"=1073676418, "source"="VISA Close in ZaberTSeries.lvlib:Close.vi->main 1.17a beta.vi"}
  in  "mirr_VISA":refnum<visa-resource-name>="COM7"
  in  "mirr_X#":u8=1
  in  "Operating mode\nHP & QE / HS & DiCam Pro":u32=1
  in  "Frame trigger \n(High Performance and QE only)":u16
  in  "LS310  EPICS chanel A":string="trARPES:Carving:TEMP_RBV"
  in  "Status EPICS chanel":string="trARPES:Carving:TEMP-STAT"
  # "camera"
  # "analyzer"
  # "manipulator"
  # "temperature"
  # "aquisition"
  # "delay stage"
  # "Position"
  # "Destination"
  # "WattPilot"
  # "- no settings -"
  # "waypoints are absolute values"
  # "- no settings -"
  # "waypoints are absolute values"
  # "- no settings -"
  # "waypoints are absolute values"
  # "- no settings -"
  # "waypoints are absolute values"
  # "X\nY\nZ\npolar\ntilt\nazimut"
  # "waypoint \"0\" is start position"
  # "X\nY"
  # "waypoint \"0\" is start position"
  # "waypoints are absolute values"
  # "- no settings -"
  # "waypoints are absolute values"
  # "- no settings -"
  # "waypoints are absolute values"
  # "- no settings -"
  # "waypoints are absolute values"
  # "- no settings -"
  # "waypoints are absolute values"
  # "X\nY\nZ\npolar\ntilt\nazimut"
  # "waypoint \"0\" is start position"
  # "X\nY"
  # "waypoint \"0\" is start position"
  # "waypoints are absolute values"
  # "camera"
  # "phoibos"
  # "ESP301"
  # "manipulator"
  # "mirror"
  # "delay"
  # "waveplate"
  # "stage2"
  # "0 = sequential\n1 = simultaneous"
  # "0 = internal\n1 = external rising\n2 = external falling"
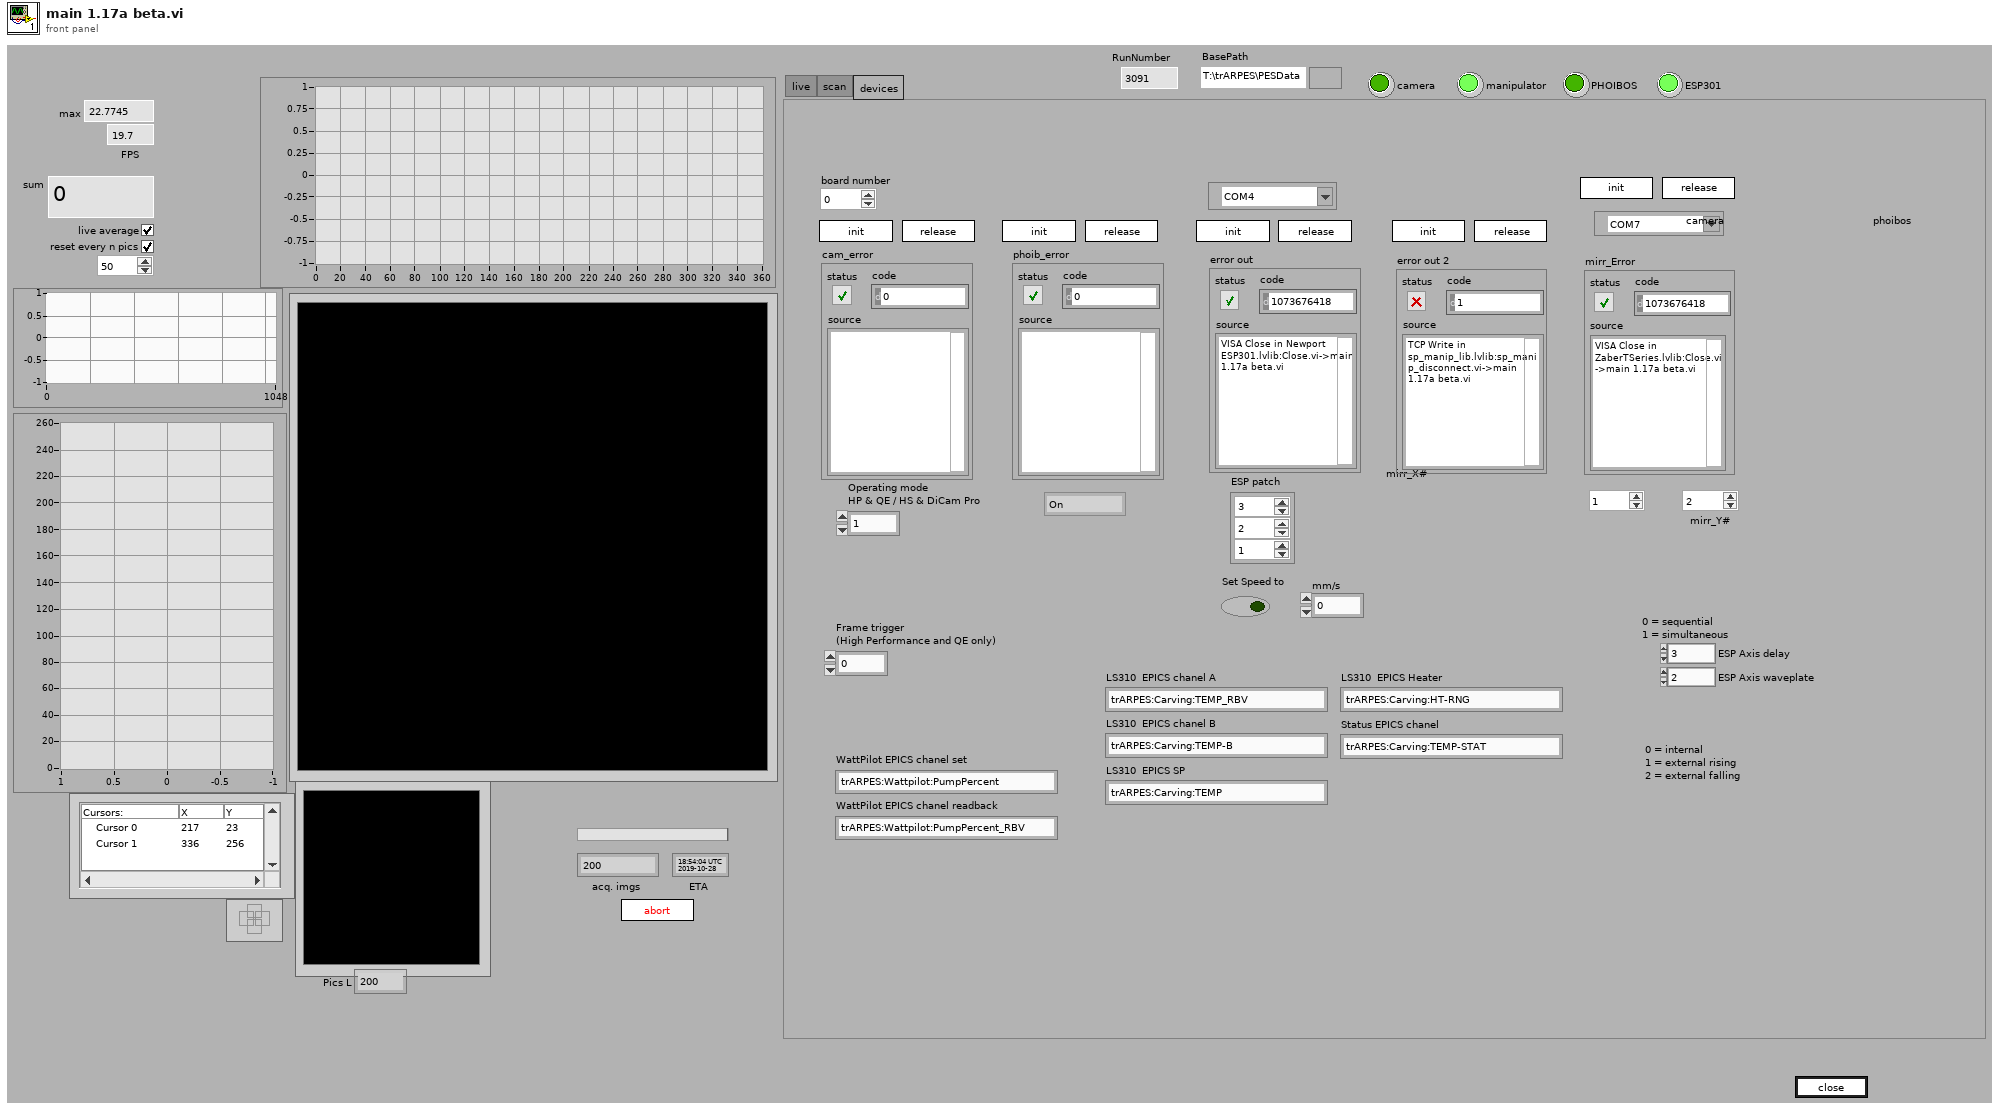
[diagram p1: front panel]
types:
  T1 = enum16{"HighMagnification", "MediumMagnification", "LowMagnification", "HighAngularDispersion", "MediumAngularDispersion", "LowAngularDispersion", "WideAngleMode", "LargeArea", "MediumArea", "SmallArea", "HighMagnification2", "SmallArea2"}
  T2 = enum32{"none", "delay", "wattpilot", "waveplate", "stage2", "manipulator", "mirror", "temperature", "voltage"}
  T3 = typedef "DEF_dev_state.ctl" = i32
  T4 = cluster{"queue out":refnum<queue>, "queue out":refnum<queue>, "queue out":refnum<queue>, "queue out":refnum<queue>, "queue out":refnum<queue>, "queue out":refnum<queue>, "queue out":refnum<queue>}
  T5 = typedef "LVCursorListTypeDef.ctl" = cluster{"Name":string, "Color":u32, "Style":u8, "Point Style":u8, "Name Visible":bool, "Allow Drag":bool, "Cursor Mode":u32, "Plot":i32, "Index":i32, "Position":cluster{"X":dbl, "Y":dbl}, "X Scale":u32, "Y Scale":u32, "Watch Plots":i32[], "Watch All Plots":bool, "Plot Area":i32, "Label Offset":cluster{"X":dbl, "Y":dbl}}[]
  T6 = cluster{"mirr_X#":u8, "Command":u8, dbl, "Response Count":i32}
  T7 = cluster{"mirr_Y#":u8, "Command":u8, dbl, "Response Count":i32}
  T8 = cluster{i32, "Command":u8, i32, "Response Count":i32}
  T9 = cluster{"Axis_Name":string, "Axis_Type":string, "Axis_Position":dbl, "continous":bool, "moving":bool}[]
  T10 = typedef "DEF_dev_type.ctl" = enum32{"devA (analyzer)", "devD (detector)"}
  T11 = cluster{"Camera type":u32, "Operating mode\nHP & QE / HS & DiCam Pro ":u32, "Frame trigger \n(High Performance and QE only)":u16, "Sequence trigger":u16, "Low Light\n(QE only)":bool, "Gain":bool, "Horzontal\nbinning":u16, "Vertical\nbinning ":u16, "ROI Left":i32, "ROI Right":i32, "ROI Top":i32, "ROI Bottom":i32}
  T12 = cluster{"Name":string, "Color":u32, "Style":u8, "Point Style":u8, "Name Visible":bool, "Allow Drag":bool, "Cursor Mode":u32, "Plot":i32, "Index":i32, "Position":cluster{"X":dbl, "Y":dbl}, "X Scale":u32, "Y Scale":u32, "Watch Plots":i32[], "Watch All Plots":bool, "Plot Area":i32, "Label Offset":cluster{"X":dbl, "Y":dbl}}
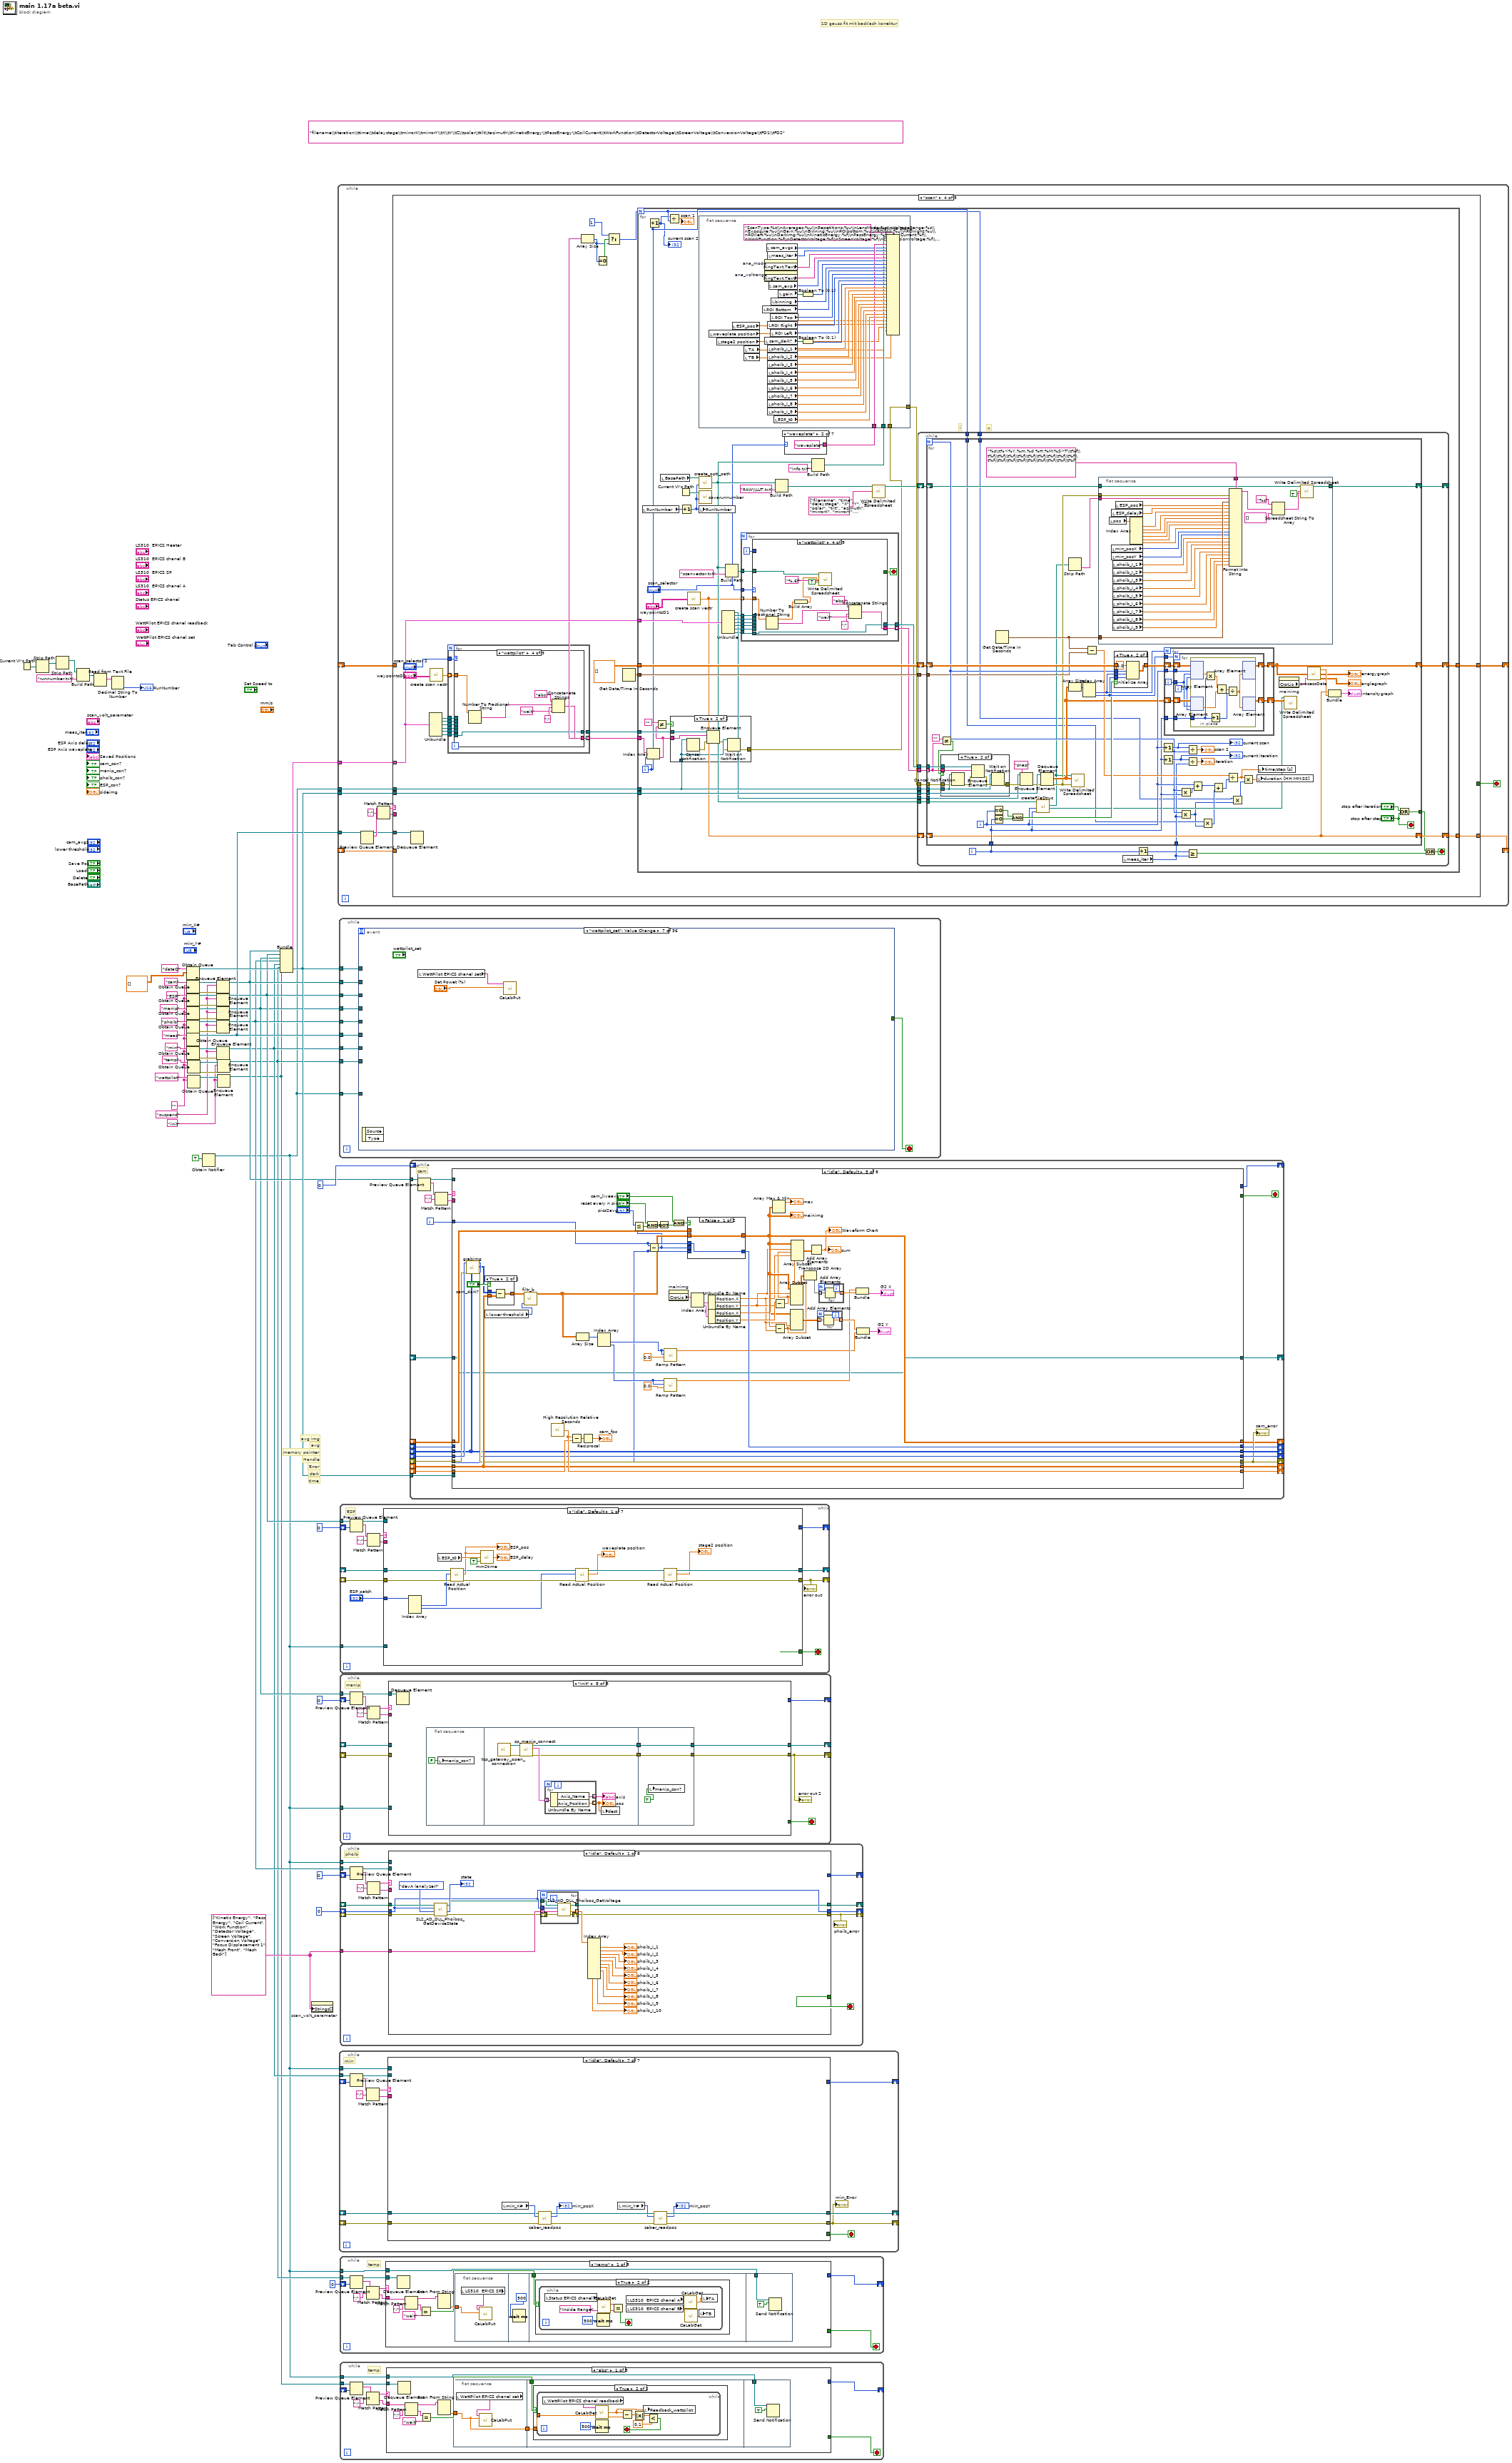
[diagram p0: block diagram]
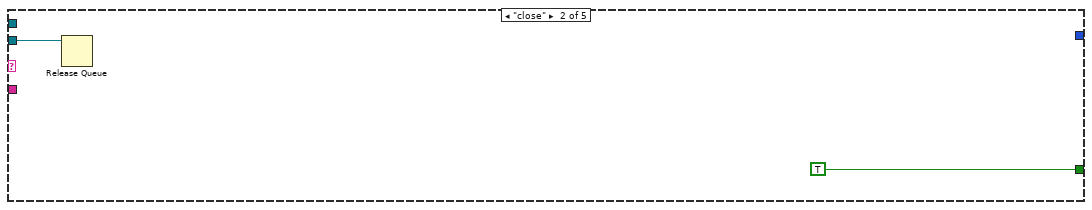
[diagram p3: hidden frame]
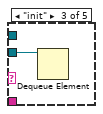
[diagram p4: hidden frame]
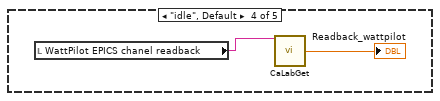
[diagram p5: hidden frame]
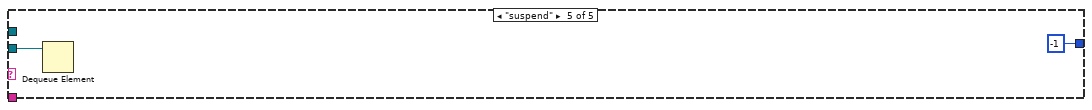
[diagram p6: hidden frame]
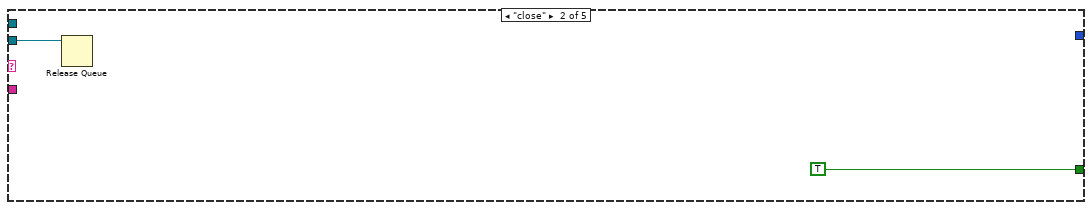
[diagram p8: hidden frame]
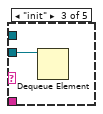
[diagram p9: hidden frame]
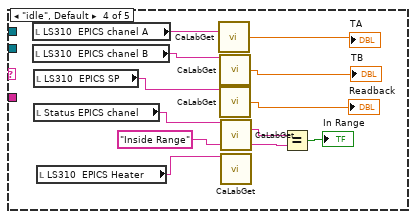
[diagram p10: hidden frame]
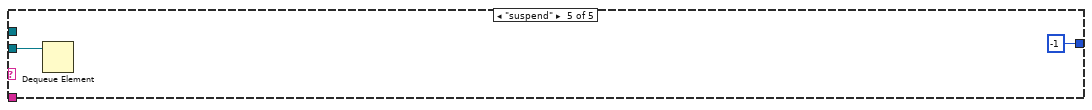
[diagram p11: hidden frame]
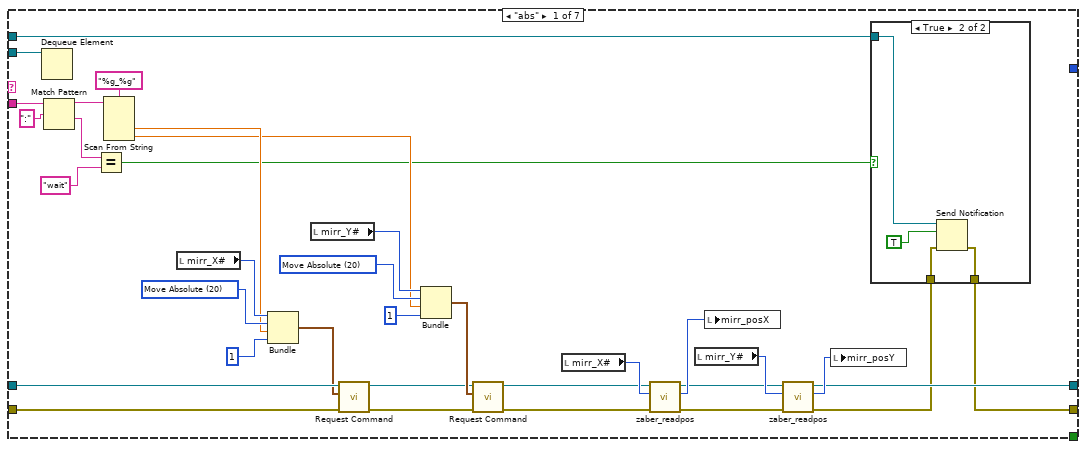
[diagram p12: hidden frame]
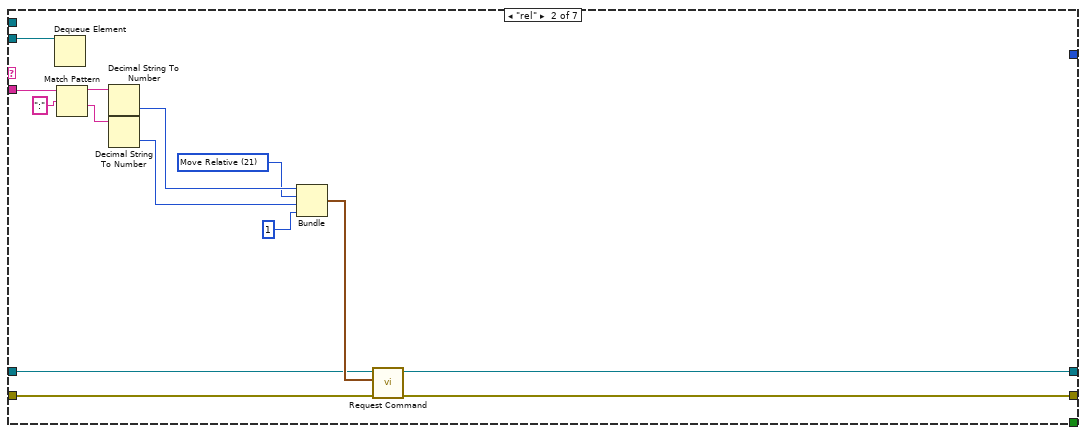
[diagram p14: hidden frame]
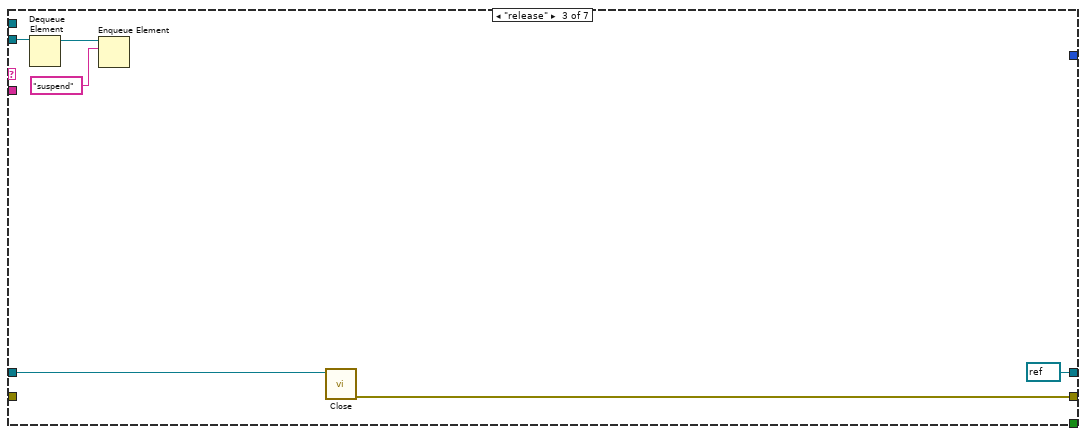
[diagram p15: hidden frame]
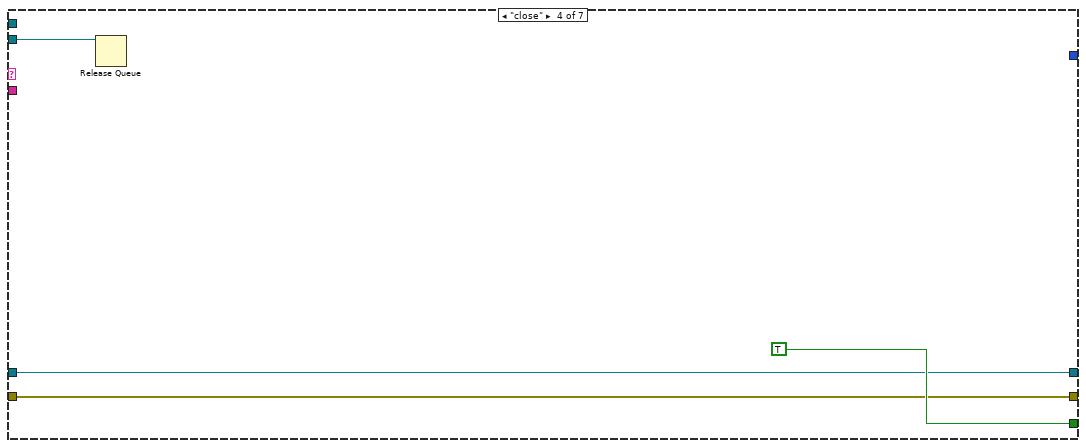
[diagram p16: hidden frame]
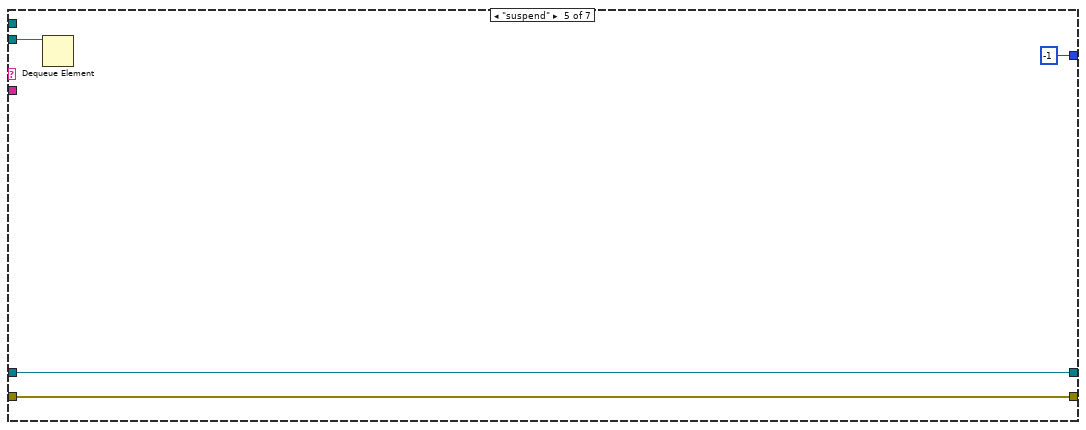
[diagram p17: hidden frame]
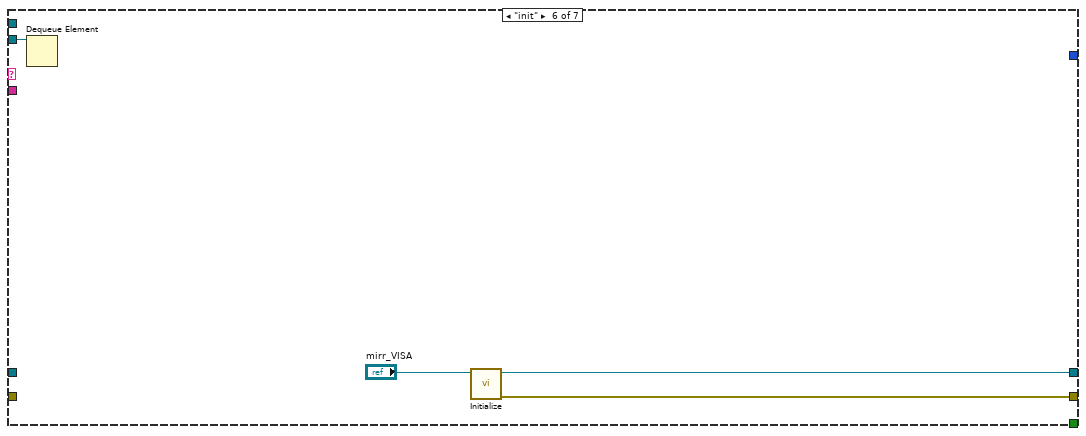
[diagram p18: hidden frame]
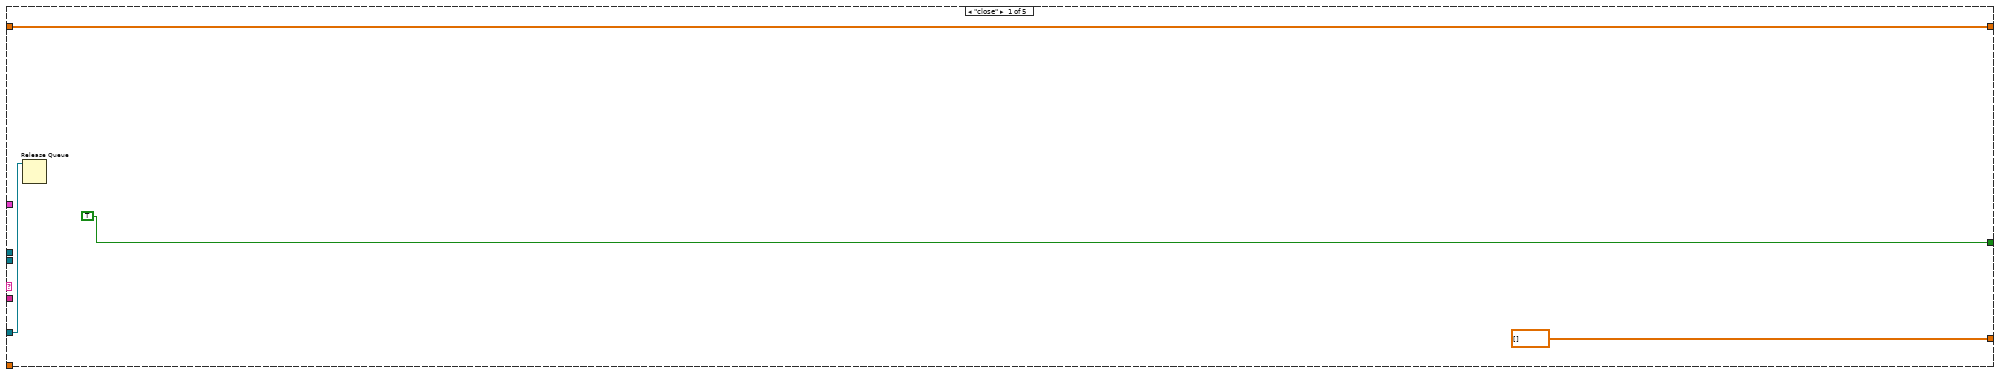
[diagram p19: hidden frame]
diagram:
  (unwired) "filename\\titeration\\ttime\\tdelaystage\\tmirrorX\\tmirrorY\\tX\\tY\\tZ\\tpolar\\ttilt\\tazimuth\\tKineticEnergy\\tPassEnergy\\tCoilCurrent\\tWorkFunction\\tDetectorVoltage\\tScreenVoltage\\tConversionVoltage\\tFD1\\tFD2"
  w18 = string[] ["Kinetic Energy", "Pass Energy", "Coil Current", "Work Function", "Detector Voltage", "Screen Voltage", "Conversion Voltage", "Focus Displacement 1", "Mesh Front", "Mesh Back"]
  w1 = "init" ("name (unnamed)")
  w8 = "suspend" ("name (unnamed)")
  w2 = "" ("name (unnamed)")
  # "1D gauss fit mit backlash korrektur"
  # "avg img"
  # "avg"
  # "time"
  # "dark"
  # "Error"
  # "Handle"
  # "memory pointer"
  n1 = Current VI's Path() -> (path=w26:path)
  n2 = Strip Path(path=w26) -> (stripped path=w30:path)  [unwired: 1 out]
  n3 = Strip Path(path=w30) -> (stripped path=w31:path)  [unwired: 1 out]
  n4 = Build Path(base path=w31, name or relative path="runnumber.txt") -> (appended path=w28:path)
  n5 = Read from Text File(file (use dialog)=w28) -> (text=w29:string)  [unwired: 3 in, 3 out]
  n6 = Decimal String To Number(string=w29) -> (number=→"RunNumber":i32)  [unwired: 2 in, 1 out]
  n7 = Obtain Queue(name (unnamed)="dataQ", element data type=dbl[][] []) -> (queue out=w32:refnum<queue>)  [unwired: 3 in, 2 out]
  n8 = Obtain Queue(name (unnamed)="cam", element data type=w2) -> (queue out=w51:refnum<queue>, error out=w50:errorcluster)  [unwired: 3 in, 1 out]
  n9 = Obtain Queue(name (unnamed)="ESP", element data type=w2) -> (queue out=w48:refnum<queue>, error out=w49:errorcluster)  [unwired: 3 in, 1 out]
  n10 = Obtain Queue(name (unnamed)="manip", element data type=w2) -> (queue out=w45:refnum<queue>, error out=w44:errorcluster)  [unwired: 3 in, 1 out]
  n11 = Obtain Queue(name (unnamed)="phoib", element data type=w2) -> (queue out=w42:refnum<queue>, error out=w43:errorcluster)  [unwired: 3 in, 1 out]
  n12 = Obtain Queue(name (unnamed)="meas", element data type=w2) -> (queue out=w25:refnum<queue>)  [unwired: 3 in, 2 out]
  n13 = Obtain Queue(name (unnamed)="mirr", element data type=w2) -> (queue out=w16:refnum<queue>, error out=w15:errorcluster)  [unwired: 3 in, 1 out]
  n14 = Obtain Queue(name (unnamed)="temp", element data type=w2) -> (queue out=w11:refnum<queue>, error out=w10:errorcluster)  [unwired: 3 in, 1 out]
  n15 = Obtain Queue(name (unnamed)="wattpilot", element data type=w2) -> (queue out=w5:refnum<queue>)  [unwired: 3 in, 2 out]
  n16 = Obtain Notifier(notification data type=TRUE) -> (notifier out=w6:refnum<notifier>)  [unwired: 3 in, 2 out]
  n17 = Enqueue Element(queue=w51, element=w8, error in (no error)=w50) -> (queue out=w23:refnum<queue>)  [unwired: 1 in, 2 out]
  n18 = Enqueue Element(queue=w48, element=w8, error in (no error)=w49) -> (queue out=w22:refnum<queue>)  [unwired: 1 in, 2 out]
  n19 = Enqueue Element(queue=w45, element=w8, error in (no error)=w44) -> (queue out=w21:refnum<queue>)  [unwired: 1 in, 2 out]
  n20 = Enqueue Element(queue=w42, element=w8, error in (no error)=w43) -> (queue out=w20:refnum<queue>)  [unwired: 1 in, 2 out]
  n21 = Enqueue Element(queue=w16, element=w8, error in (no error)=w15) -> (queue out=w13:refnum<queue>)  [unwired: 1 in, 2 out]
  n22 = Enqueue Element(queue=w11, element=w1, error in (no error)=w10) -> (queue out=w7:refnum<queue>)  [unwired: 1 in, 2 out]
  n23 = Enqueue Element(queue=w5, element=w1) -> (queue out=w4:refnum<queue>)  [unwired: 2 in, 2 out]
  n24 = Bundle("queue out"=w23, "queue out"=w22, "queue out"=w21, "queue out"=w20, "queue out"=w13, "queue out"=w7, "queue out"=w4) -> (w24:T4)  [unwired: 1 in]
  n25 = property on="scan_volt_parameter" class="CmbBox"("Strings[]"=w18) -> ()  [unwired: 2 in, 2 out]
  n26 = while {
    tunnel: w32 -> [w66]
    tunnel: w25 -> [w63]
    tunnel: w24 -> [w59]
    shift-right: [w57] -> _
    shift-left: _ -> [w56]
    tunnel: w6 -> [w55]
    shift-right: [w54] -> _
    shift-left: _ -> [w53]
    stop <- w58 stop-if-true
    n27 = Preview Queue Element(queue=w63) -> (queue out=w60:refnum<queue>, element=w65:string)  [unwired: 2 in, 2 out]
    n28 = Match Pattern(string=w65, regular expression=":") -> (before substring=w62:string, after substring=w61:string)  [unwired: 1 in, 2 out]
    n29 = case shown="\"scan\"" w62 {
      tunnel: w66 -> [_ _ w122 w146 _]
      tunnel: w61 -> [_ _ _ _ _]
      tunnel: w60 -> [w70 _ w123 w142 w626]
      tunnel: [TRUE _ _ _ _] -> w58
      tunnel: w59 -> [_ _ w110 w139 _]
      tunnel: [w68 w72 w108 w144 w632] -> w57
      tunnel: w56 -> [w68 w72 w108 _ w632]
      tunnel: w55 -> [_ _ _ w143 _]
      tunnel: [dbl[] [] ("Array") w71 w80 w140 w628] -> w54
      tunnel: w53 -> [_ w71 w80 _ w628]
      frame "close" {
        n30 = Release Queue(queue=w70) -> ()  [unwired: 2 in, 3 out]
      }
      frame "idle", Default {
      }
      frame "single" {
        n31 = Dequeue Element(queue=w123) -> ()  [unwired: 2 in, 4 out]
        n32 = local read "RunNumber"() -> (w117:u16)
        n33 = local read "BasePath"() -> (w118:path)
        n34 = Unbundle(w110) -> ("queue out"=w109:refnum<queue>)  [unwired: 6 out]
        n35 = Increment(x=w117) -> (x+1=w119:u16)
        n36 = Current VI's Path() -> (path=w116:path)
        n37 = call "saverunnumber.vi"("RunNumber"=w119, "VI path"=w116) -> ()  [unwired: 10 in]
        n38 = local write "RunNumber"(w119) -> ()
        n39 = call "create_opti_path.vi"("RunNumber"=w119, "base path"=w118) -> ("Path"=w112:path)  [unwired: 2 in]
        n40 = Enqueue Element(queue=w109, element="snap" ("string")) -> (error out=w120:errorcluster)  [unwired: 2 in, 2 out]
        n41 = Build Path(base path=w112, name or relative path="info.txt") -> (appended path=w81:path)
        n42 = Build Path(base path=w112, name or relative path="AVG\\000.tsv") -> (appended path=w114:path)
        n43 = Dequeue Element(queue=w122, error in (no error)=w120) -> (element=w111:dbl[][])  [unwired: 1 in, 3 out]
        n44 = call-poly <vilib>:"Write Delimited Spreadsheet.vi"("file path (dialog if empty)"=w114, "2D data"=w111) -> ()  [unwired: 12 in, 2 out]
        n45 = local read "ROI Bottom"() -> (w88:i32)
        n46 = property on="ana_mode" class="Enum (strict)"() -> ("RingText.Text"=w103:string)  [unwired: 2 in, 2 out]
        n47 = property on="ana_voltrange" class="Enum (strict)"() -> ("RingText.Text"=w102:string)  [unwired: 2 in, 2 out]
        n48 = local read "cam_dark?"() -> (w84:bool)
        n49 = local read "cam_avgs"() -> (w105:i32)
        n50 = local read "meas_iter"() -> (w104:i32)
        n51 = local read "phoib_I_1"() -> (w101:dbl)
        n52 = local read "phoib_I_2"() -> (w100:dbl)
        n53 = local read "phoib_I_3"() -> (w99:dbl)
        n54 = local read "phoib_I_4"() -> (w98:dbl)
        n55 = local read "phoib_I_5"() -> (w97:dbl)
        n56 = local read "phoib_I_6"() -> (w96:dbl)
        n57 = local read "phoib_I_7"() -> (w95:dbl)
        n58 = local read "phoib_I_8"() -> (w94:dbl)
        n59 = local read "phoib_I_9"() -> (w93:dbl)
        n60 = local read "ROI Right"() -> (w86:i32)
        n61 = local read "cam_exp"() -> (w92:u32)
        n62 = local read "ROI Top"() -> (w87:i32)
        n63 = local read "ROI Left"() -> (w85:i32)
        n64 = local read "binning"() -> (w89:u16)
        n65 = local read "pos"() -> (w79:dbl[])
        n66 = local read "gain"() -> (w91:bool)
        n67 = Get Date/Time In Seconds() -> (seconds since 1Jan1904=w82:timestamp)
        n68 = Boolean To (0,1)(Boolean=w91) -> (0, 1=w90:i16)
        n69 = Boolean To (0,1)(Boolean=w84) -> (0, 1=w83:i16)
        n70 = Index Array(array=w79) -> (element #1=w78:dbl, element #2=w77:dbl, element #3=w76:dbl, element #4=w75:dbl, element #5=w74:dbl, element #6=w73:dbl)  [unwired: 6 in]
        n71 = Format Into String(format string="ScanType=%s\\nAverages=%u\\nRepetitions=%u\\nLensMode=%s\\nVoltageRange=%s\\nKineticEnergy=%f\\nPassEnergy=%f\\nCoilCurrent=%f\\nWorkFunction=%f\\nDetectorVoltage=%f\\nScreenVoltage=%f\\nConversionVoltage=%f\\nFocusDisplacement1=%f\\nFocusDisplacement2=%f\\nExposure=%u\\nGain=%u\\nBinning=%u\\nROIbottom=%u\\nROItop=%u\\nROIright=%u\\nROIleft=%u\\nDarkImg=%u\\nStartTime=%<%Y.%m.%d %H:%M:%S>T\\n\nX=%f\\n\nY=%f\\n\nZ=%f\\n\nPolar=%f\\n\nTilt=%f\\n\nAzimuth=%f\\n", initial string=w81, "single" ("input 1"), w105, w104, w103, w102, w101, w100, w99, w98, w97, w96, w95, w94, w93, w92, w90, w89, w88, w87, w86, w85, w83, w82, w78, w77, w76, w75, w74, w73) -> ()  [unwired: 1 in, 2 out]
      }
      frame "scan" {
        n72 = Dequeue Element(queue=w142) -> ()  [unwired: 2 in, 4 out]
        n73 = Unbundle(w139) -> ("queue out"=w138:refnum<queue>, "queue out"=w137:refnum<queue>, "queue out"=w136:refnum<queue>, "queue out"=w135:refnum<queue>, "queue out"=w134:refnum<queue>, "queue out"=w124:refnum<queue>)  [unwired: 1 out]
        n74 = call "create scan vectr.vi"("Table Control"="waypointsD2") -> ("Array"=w132:dbl[])
        n75 = for {
          tunnel: "scan_selector 2" -> [w156]
          tunnel: w138 -> [w155]
          tunnel: w137 -> [w154]
          tunnel: w136 -> [w153]
          tunnel: w135 -> [w152]
          tunnel: w134 -> [w151]
          tunnel: [w150] -> w129 mode=indexing
          tunnel: [w149] -> w133
          tunnel: w132 -> [w148] mode=indexing
          tunnel: w124 -> [w147]
          n76 = case shown="\"wattpilot\"" w156 {
            tunnel: ["" w160 w171 w182 w188 w199 w217 w231 w243] -> w150
            tunnel: w155 -> [w157 w159 w173 _ w187 _ _ _ _]
            tunnel: w154 -> [_ _ _ _ _ w198 _ _ _]
            tunnel: w153 -> [_ _ _ _ _ _ _ _ w242]
            tunnel: w152 -> [_ _ _ _ _ _ w216 _ _]
            tunnel: w151 -> [_ _ _ _ _ _ _ w230 _]
            tunnel: [w157 w159 w173 w181 w187 w198 w216 w230 w242] -> w149
            tunnel: w148 -> [_ w161 w172 w183 w189 w200 w215 w233 w244]
            tunnel: w147 -> [_ _ _ w181 _ _ _ _ _]
            frame "none", Default {
            }
            frame "delay" {
              w164 = ":" ("string")
              n77 = local read "ESP_t0"() -> (w168:dbl)
              n78 = call "time2mm.vi"("fs[1]/ps[0]"=TRUE, "Offset (mm)"=w168, "time"=w161) -> ("position (mm)"=w169:dbl)
              n79 = Number To Decimal String(number=0) -> (decimal integer string=w166:string)  [unwired: 1 in]
              n80 = Number To Fractional String(number=w169) -> (F-format string=w162:string)  [unwired: 3 in]
              n81 = Concatenate Strings("abs:" ("string"), w166, w164, w162, w164, "wait" ("string")) -> (w160:string)
            }
            frame "waveplate" {
              w179 = ":" ("string")
              n82 = Number To Fractional String(number=w172) -> (F-format string=w174:string)  [unwired: 3 in]
              n83 = Number To Decimal String(number=1) -> (decimal integer string=w177:string)  [unwired: 1 in]
              n84 = Concatenate Strings("abs:" ("string"), w177, w179, w174, w179, "wait" ("string")) -> (w171:string)
            }
            frame "wattpilot" {
              n85 = Number To Fractional String(number=w183) -> (F-format string=w184:string)  [unwired: 3 in]
              n86 = Concatenate Strings("abs:" ("string"), w184, ":" ("string"), "wait" ("string")) -> (w182:string)
            }
            frame "stage2" {
              w194 = ":" ("string")
              n87 = Number To Decimal String(number=2) -> (decimal integer string=w191:string)  [unwired: 1 in]
              n88 = Number To Fractional String(number=w189) -> (F-format string=w190:string)  [unwired: 3 in]
              n89 = Concatenate Strings("abs:" ("string"), w191, w194, w190, w194, "wait" ("string")) -> (w188:string)
            }
            frame "manipulator" {
              n90 = call-poly <vilib>:"Vector Norm.vi"("Input Vector"="scan_manip_deltas 2") -> ("norm"=w201:dbl)  [unwired: 9 in, 1 out]
              n91 = Divide(x="scan_manip_deltas 2", y=w201) -> (x/y=w202:dbl[])
              n92 = Multiply(x=w202, y=w200) -> (x*y=w213:dbl[])
              n93 = Add(x="scan_manip_start 2", y=w213) -> (x+y=w214:dbl[])
              n94 = Index Array(array=w214) -> (element #1=w211:dbl, element #2=w210:dbl, element #3=w209:dbl, element #4=w208:dbl, element #5=w207:dbl, element #6=w206:dbl)  [unwired: 6 in]
              n95 = Format Into String(format string="%g_%g_%g_%g_%g_%g", w211, w210, w209, w208, w207, w206) -> (resulting string=w204:string)  [unwired: 2 in, 1 out]
              n96 = Concatenate Strings("abs:" ("string"), w204, ":wait" ("string")) -> (w199:string)
            }
            frame "mirror" {
              n97 = call-poly <vilib>:"Vector Norm.vi"("Input Vector"="scan_mirr_deltas 2") -> ("norm"=w220:dbl)  [unwired: 9 in, 1 out]
              n98 = Divide(x="scan_mirr_deltas 2", y=w220) -> (x/y=w221:dbl[])
              n99 = Multiply(x=w221, y=w215) -> (x*y=w228:dbl[])
              n100 = Add(x="scan_mirr_start 2", y=w228) -> (x+y=w229:dbl[])
              n101 = Index Array(array=w229) -> (element #1=w225:dbl, element #2=w224:dbl)  [unwired: 2 in]
              n102 = Format Into String(format string="%g_%g", w225, w224) -> (resulting string=w222:string)  [unwired: 2 in, 1 out]
              n103 = Concatenate Strings("abs:" ("string"), w222, ":wait" ("string")) -> (w217:string)
            }
            frame "temperature" {
              n104 = Number To Fractional String(number=w233) -> (F-format string=w235:string)  [unwired: 3 in]
              n105 = Concatenate Strings("ramp:" ("string"), w235) -> (w236:string)
              n106 = case shown="True" "Wait for T 2" {
                tunnel: w236 -> [w238 w241]
                tunnel: ":wait" ("string") -> [_ w240]
                tunnel: [w238 w239] -> w231
                frame False {
                }
                frame True {
                  n107 = Concatenate Strings(w241, w240) -> (w239:string)
                }
              }
            }
            frame "voltage" {
              n108 = Number To Fractional String(number=w244) -> (F-format string=w248:string)  [unwired: 3 in]
              n109 = Concatenate Strings("setsgl:" ("string"), "scan_volt_parameter 2", ":" ("string"), w248) -> (w243:string)
            }
          }
        }
        n110 = Array Size(array=w129) -> (size(s)=w126:i32)
        n111 = Equal To 0?(x=w126) -> (x = 0?=w128:bool)
        n112 = Select(t=1, s=w128, f=w126) -> (s? t:f=w125:i32)
        n113 = Get Date/Time In Seconds() -> (seconds since 1Jan1904=w141:timestamp)
        n114 = for {
          N: w125 -> [w250]
          tunnel: w146 -> [w292]
          tunnel: dbl[][][] [] -> [w291]
          tunnel: [w290] -> w144
          tunnel: w143 -> [w287]
          tunnel: w141 -> [w289]
          tunnel: [w288] -> w140
          tunnel: w139 -> [w279]
          tunnel: w129 -> [w254]
          tunnel: w133 -> [w260]
          i -> [w252]
          # "i"
          # "n"
          n115 = local read "RunNumber"() -> (w272:u16)
          n116 = Index Array(array=w254, index=w252) -> (element=w253:string)
          n117 = Increment(x=w252) -> (x+1=w249:i32)
          "current scan 2" <- w249
          n118 = Not Equal?(x="", y=w253) -> (x != y?=w285:bool)
          n119 = local read "BasePath"() -> (w271:path)
          n120 = Divide(x=w249, y=w250) -> (x/y=→"scan 1":dbl)
          n121 = case shown="True" w285 {
            tunnel: w260 -> [_ w475]
            tunnel: w253 -> [_ w474]
            tunnel: w287 -> [_ w473]
            tunnel: [errorcluster {"status"=FALSE, "code"=0, "source"=""} ("error out") w470] -> w259
            frame False {
            }
            frame True {
              n122 = Cancel Notification(0:w473) -> (11:w472:errorcluster)  [unwired: 1 in, 2 out]
              n123 = Enqueue Element(queue=w475, element=w474, error in (no error)=w472) -> (error out=w471:errorcluster)  [unwired: 1 in, 2 out]
              n124 = Wait on Notification(notifier=w473, error in (no error)=w471) -> (error out=w470:errorcluster)  [unwired: 2 in, 3 out]
            }
          }
          n125 = Current VI's Path() -> (path=w273:path)
          n126 = Increment(x=w272) -> (x+1=w270:u16)
          n127 = call "create scan vectr.vi"("Table Control"="waypointsD1") -> ("Array"=w261:dbl[])
          n128 = flat-sequence {
            tunnel: w275 -> [w307]
            tunnel: w262 -> [w299]
            tunnel: w259 -> [w293]
            tunnel: [w293] -> w258
            frame #0 {
              n129 = local read "waveplate position"() -> (w296:dbl)
              n130 = local read "stage2 position"() -> (w295:dbl)
              n131 = local read "ESP_pos"() -> (w297:dbl)
              n132 = local read "TA"() -> (w298:dbl)
              n133 = local read "TB"() -> (w294:dbl)
              n134 = local read "ROI Bottom"() -> (w311:i32)
              n135 = property on="ana_mode" class="Enum (strict)"() -> ("RingText.Text"=w303:string)  [unwired: 2 in, 2 out]
              n136 = property on="ana_voltrange" class="Enum (strict)"() -> ("RingText.Text"=w304:string)  [unwired: 2 in, 2 out]
              n137 = local read "cam_dark?"() -> (w306:bool)
              n138 = local read "cam_avgs"() -> (w301:i32)
              n139 = local read "meas_iter"() -> (w302:i32)
              n140 = local read "ROI Right"() -> (w313:i32)
              n141 = local read "phoib_I_1"() -> (w316:dbl)
              n142 = local read "phoib_I_2"() -> (w317:dbl)
              n143 = local read "phoib_I_3"() -> (w318:dbl)
              n144 = local read "phoib_I_4"() -> (w319:dbl)
              n145 = local read "phoib_I_5"() -> (w320:dbl)
              n146 = local read "phoib_I_6"() -> (w321:dbl)
              n147 = local read "phoib_I_7"() -> (w322:dbl)
              n148 = local read "phoib_I_8"() -> (w323:dbl)
              n149 = local read "phoib_I_9"() -> (w324:dbl)
              n150 = local read "cam_exp"() -> (w308:u32)
              n151 = local read "ROI Top"() -> (w312:i32)
              n152 = local read "ROI Left"() -> (w314:i32)
              n153 = local read "binning"() -> (w310:u16)
              n154 = local read "ESP_t0"() -> (w325:dbl)
              n155 = local read "gain"() -> (w305:bool)
              n156 = Boolean To (0,1)(Boolean=w305) -> (0, 1=w309:i16)
              n157 = Boolean To (0,1)(Boolean=w306) -> (0, 1=w315:i16)
              n158 = Format Into String(format string="ScanType:%s\\nAverages:%u\\nRepetitions:%u\\nLensMode:%s\\nVoltageRange:%s\\nExposure:%u\\nGain:%u\\nBinning:%u\\nROIbottom:%u\\nROItop:%u\\nROIright:%u\\nROIleft:%u\\nDarkImg:%u\\nKineticEnergy:%f\\nPassEnergy:%f\\nCoilCurrent:%f\\nWorkFunction:%f\\nDetectorVoltage:%f\\nScreenVoltage:%f\\nConversionVoltage:%f\\nFocusDisplacement1:%f\\nFocusDisplacement2:%f\\nTimeZero:%f\\nDelayStage:%f\\nWaveplate:%f\\n2ndStage:%f\\nTempA:%f\\nTempB:%f\\n", initial string=w299, w307, w301, w302, w303, w304, w308, w309, w310, w311, w312, w313, w314, w315, w316, w317, w318, w319, w320, w321, w322, w323, w324, w325, w297, w296, w295, w298, w294) -> ()  [unwired: 1 in, 2 out]
            }
          }
          n159 = call "create_opti_path.vi"("RunNumber"=w270, "base path"=w271) -> ("Path"=w263:path)  [unwired: 2 in]
          n160 = call "saverunnumber.vi"("RunNumber"=w270, "VI path"=w273) -> ()  [unwired: 10 in]
          n161 = local write "RunNumber"(w270) -> ()
          n162 = Unbundle(w279) -> ("queue out"=w278:refnum<queue>, "queue out"=w280:refnum<queue>, "queue out"=w281:refnum<queue>, "queue out"=w282:refnum<queue>, "queue out"=w283:refnum<queue>, "queue out"=w284:refnum<queue>, "queue out"=w251:refnum<queue>)
          n163 = Build Path(base path=w263, name or relative path="scanvector.txt") -> (appended path=w265:path)
          n164 = for {
            tunnel: [w345] -> w277 mode=indexing
            tunnel: [w344] -> w276
            tunnel: w280 -> [w343]
            tunnel: w281 -> [w342]
            tunnel: w282 -> [w341]
            tunnel: w283 -> [w340]
            tunnel: w265 -> [w339]
            tunnel: w284 -> [w338]
            tunnel: w261 -> [w337] mode=indexing
            tunnel: "scan_selector" -> [w335]
            tunnel: w251 -> [w333]
            i -> [w334]
            stop <- w336 stop-if-true
            n165 = case shown="\"wattpilot\"" w335 {
              tunnel: w337 -> [w354 _ w368 w382 w390 w421 w433 w450 w459]
              tunnel: [w352 w362 w365 w379 w391 w409 w430 w448 w463] -> w344
              tunnel: [w357 "" w369 w383 w392 w410 w431 w443 w464] -> w345
              tunnel: w343 -> [w352 w362 w365 _ w391 _ _ _ _]
              tunnel: w342 -> [_ _ _ _ _ w409 _ _ _]
              tunnel: w341 -> [_ _ _ _ _ _ _ _ w463]
              tunnel: w340 -> [_ _ _ _ _ _ w430 _ _]
              tunnel: w339 -> [w347 _ w367 w381 w389 w405 w427 w451 w460]
              tunnel: w338 -> [_ _ _ _ _ _ _ w448 _]
              tunnel: [_ TRUE _ _ _ _ _ _ _] -> w336
              tunnel: w334 -> [_ _ _ _ _ _ _ _ _]
              tunnel: w333 -> [_ _ _ w379 _ _ _ _ _]
              frame "delay" {
                w359 = ":" ("string")
                n166 = local read "ESP_t0"() -> (w353:dbl)
                n167 = call "time2mm.vi"("fs[1]/ps[0]"=TRUE, "Offset (mm)"=w353, "time"=w354) -> ("position (mm)"=w349:dbl)
                n168 = Build Array(w349) -> (w348:dbl[])
                n169 = Number To Decimal String(number=0) -> (decimal integer string=w356:string)  [unwired: 1 in]
                n170 = Number To Fractional String(number=w349) -> (F-format string=w361:string)  [unwired: 3 in]
                n171 = call-poly <vilib>:"Write Delimited Spreadsheet.vi"("file path (dialog if empty)"=w347, "format (%.3f)"="%.6f", "1D data"=w348, "append to file? (F)"=TRUE) -> ()  [unwired: 10 in, 2 out]
                n172 = Concatenate Strings("abs:" ("string"), w356, w359, w361, w359, "wait" ("string")) -> (w357:string)
              }
              frame "none", Default {
              }
              frame "waveplate" {
                w366 = ":" ("string")
                n173 = Number To Fractional String(number=w368) -> (F-format string=w377:string)  [unwired: 3 in]
                n174 = Build Array(w368) -> (w371:dbl[])
                n175 = Number To Decimal String(number=1) -> (decimal integer string=w374:string)  [unwired: 1 in]
                n176 = call-poly <vilib>:"Write Delimited Spreadsheet.vi"("file path (dialog if empty)"=w367, "format (%.3f)"="%.6f", "1D data"=w371, "append to file? (F)"=TRUE) -> ()  [unwired: 10 in, 2 out]
                n177 = Concatenate Strings("abs:" ("string"), w374, w366, w377, w366, "wait" ("string")) -> (w369:string)
              }
              frame "wattpilot" {
                n178 = Number To Fractional String(number=w382) -> (F-format string=w388:string)  [unwired: 3 in]
                n179 = Build Array(w382) -> (w384:dbl[])
                n180 = call-poly <vilib>:"Write Delimited Spreadsheet.vi"("file path (dialog if empty)"=w381, "format (%.3f)"="%.6f", "1D data"=w384, "append to file? (F)"=TRUE) -> ()  [unwired: 10 in, 2 out]
                n181 = Concatenate Strings("abs:" ("string"), w388, ":" ("string"), "wait" ("string")) -> (w383:string)
              }
              frame "stage2" {
                w394 = ":" ("string")
                n182 = Build Array(w390) -> (w399:dbl[])
                n183 = Number To Decimal String(number=2) -> (decimal integer string=w400:string)  [unwired: 1 in]
                n184 = Number To Fractional String(number=w390) -> (F-format string=w401:string)  [unwired: 3 in]
                n185 = call-poly <vilib>:"Write Delimited Spreadsheet.vi"("file path (dialog if empty)"=w389, "format (%.3f)"="%.6f", "1D data"=w399, "append to file? (F)"=TRUE) -> ()  [unwired: 10 in, 2 out]
                n186 = Concatenate Strings("abs:" ("string"), w400, w394, w401, w394, "wait" ("string")) -> (w392:string)
              }
              frame "manipulator" {
                n187 = call-poly <vilib>:"Vector Norm.vi"("Input Vector"="scan_manip_deltas") -> ("norm"=w423:dbl)  [unwired: 9 in, 1 out]
                n188 = Divide(x="scan_manip_deltas", y=w423) -> (x/y=w422:dbl[])
                n189 = Multiply(x=w422, y=w421) -> (x*y=w408:dbl[])
                n190 = Add(x="scan_manip_start", y=w408) -> (x+y=w404:dbl[])
                n191 = call-poly <vilib>:"Write Delimited Spreadsheet.vi"("file path (dialog if empty)"=w405, "format (%.3f)"="%.6f", "1D data"=w404, "append to file? (F)"=TRUE) -> ()  [unwired: 10 in, 2 out]
                n192 = Index Array(array=w404) -> (element #1=w412:dbl, element #2=w413:dbl, element #3=w414:dbl, element #4=w415:dbl, element #5=w416:dbl, element #6=w417:dbl)  [unwired: 6 in]
                n193 = Format Into String(format string="%g_%g_%g_%g_%g_%g", w412, w413, w414, w415, w416, w417) -> (resulting string=w419:string)  [unwired: 2 in, 1 out]
                n194 = Concatenate Strings("abs:" ("string"), w419, ":wait" ("string")) -> (w410:string)
              }
              frame "mirror" {
                n195 = call-poly <vilib>:"Vector Norm.vi"("Input Vector"="scan_mirr_deltas") -> ("norm"=w441:dbl)  [unwired: 9 in, 1 out]
                n196 = Divide(x="scan_mirr_deltas", y=w441) -> (x/y=w440:dbl[])
                n197 = Multiply(x=w440, y=w433) -> (x*y=w429:dbl[])
                n198 = Add(x="scan_mirr_start", y=w429) -> (x+y=w426:dbl[])
                n199 = call-poly <vilib>:"Write Delimited Spreadsheet.vi"("file path (dialog if empty)"=w427, "format (%.3f)"="%.6f", "1D data"=w426, "append to file? (F)"=TRUE) -> ()  [unwired: 10 in, 2 out]
                n200 = Index Array(array=w426) -> (element #1=w436:dbl, element #2=w437:dbl)  [unwired: 2 in]
                n201 = Format Into String(format string="%g_%g", w436, w437) -> (resulting string=w439:string)  [unwired: 2 in, 1 out]
                n202 = Concatenate Strings("abs:" ("string"), w439, ":wait" ("string")) -> (w431:string)
              }
              frame "temperature" {
                n203 = Build Array(w450) -> (w449:dbl[])
                n204 = Number To Fractional String(number=w450) -> (F-format string=w447:string)  [unwired: 3 in]
                n205 = Concatenate Strings("ramp:" ("string"), w447) -> (w445:string)
                n206 = case shown="True" "Wait for T" {
                  tunnel: w445 -> [w454 w457]
                  tunnel: ":wait" ("string") -> [_ w456]
                  tunnel: [w454 w455] -> w443
                  frame False {
                  }
                  frame True {
                    n207 = Concatenate Strings(w457, w456) -> (w455:string)
                  }
                }
                n208 = call-poly <vilib>:"Write Delimited Spreadsheet.vi"("file path (dialog if empty)"=w451, "format (%.3f)"="%.6f", "1D data"=w449, "append to file? (F)"=TRUE) -> ()  [unwired: 10 in, 2 out]
              }
              frame "voltage" {
                n209 = local read "scan_volt_parameter"() -> (w467:string)
                n210 = Build Array(w459) -> (w458:dbl[])
                n211 = Number To Fractional String(number=w459) -> (F-format string=w465:string)  [unwired: 3 in]
                n212 = Concatenate Strings("setsgl:" ("string"), w467, ":" ("string"), w465) -> (w464:string)
                n213 = call-poly <vilib>:"Write Delimited Spreadsheet.vi"("file path (dialog if empty)"=w460, "format (%.3f)"="%.6f", "1D data"=w458, "append to file? (F)"=TRUE) -> ()  [unwired: 10 in, 2 out]
              }
            }
          }
          n214 = Build Path(base path=w263, name or relative path="RAW\\LUT.txt") -> (appended path=w274:path)
          n215 = case shown="\"waveplate\"" "scan_selector" {
            tunnel: ["delay" ("input 1") "waveplate" ("input 1") "stage2" ("input 1") "manipulator" ("input 1") "temperature" "mirror" ("input 1") "voltage" ("input 1")] -> w275
            frame "delay", Default {
            }
            frame "waveplate" {
            }
            frame "stage2" {
            }
            frame "manipulator" {
            }
            frame "temperature" {
            }
            frame "mirror" {
            }
            frame "voltage" {
            }
          }
          n216 = Build Path(base path=w263, name or relative path="info.txt") -> (appended path=w262:path)
          n217 = call-poly <vilib>:"Write Delimited Spreadsheet.vi"("file path (dialog if empty)"=w274, "1D data"=string[] ["filename", "time", "delaystage", "X", "Y", "Z", "polar", "tilt", "azimuth", "mirrorX", "mirrorY", "KineticEnergy", "PassEnergy", "CoilCurrent", "WorkFunction", "DetectorVoltage", "ScreenVoltage", "ConversionVoltage", "FD1", "FD2"]) -> ("new file path (Not A Path if cancelled)"=w266:path)  [unwired: 12 in, 1 out]
          n218 = while {
            tunnel: w263 -> [w497]
            tunnel: w292 -> [w496]
            shift-right: [w495] -> w290
            shift-left: w291 -> [w494]
            tunnel: w287 -> [w493]
            tunnel: w289 -> [w492]
            tunnel: w276 -> [w491]
            tunnel: w277 -> [w490]
            tunnel: w278 -> [w489]
            shift-right: [w487] -> _
            shift-left: w266 -> [w488]
            shift-right: [w486] -> w288
            shift-left: w261 -> [w485]
            tunnel: w258 -> [w478]
            tunnel: w250 -> [w477]
            tunnel: w252 -> [w476]
            i -> [w484]
            stop <- w481 stop-if-true
            n219 = local read "meas_iter"() -> (w483:i32)
            n220 = for {
              N -> [w534]
              tunnel: w497 -> [w532]
              tunnel: w496 -> [w553]
              tunnel: w484 -> [w530]
              shift-right: [w544] -> w495
              shift-left: w494 -> [w549]
              tunnel: w493 -> [w546]
              tunnel: w492 -> [w533]
              tunnel: w491 -> [w526]
              tunnel: w490 -> [w506] mode=indexing
              tunnel: w489 -> [w525]
              shift-right: [w521] -> w487
              shift-left: w488 -> [w522]
              shift-right: [w517] -> w486
              shift-left: w485 -> [w517]
              tunnel: [w514] -> w480
              tunnel: w483 -> [w513]
              tunnel: w478 -> [w508]
              tunnel: w477 -> [w500]
              tunnel: w476 -> [w504]
              i -> [w531]
              stop <- "stop after step" stop-if-true
              n221 = Not Equal?(x="", y=w506) -> (x != y?=w505:bool)
              n222 = case shown="True" w505 {
                tunnel: [w558 w564] -> w548
                tunnel: w546 -> [_ w562]
                tunnel: w526 -> [_ w561]
                tunnel: w506 -> [_ w560]
                tunnel: w508 -> [w558 w559]
                frame False {
                }
                frame True {
                  n223 = Cancel Notification(0:w562, 3:w559) -> (11:w563:errorcluster)  [unwired: 2 out]
                  n224 = Enqueue Element(queue=w561, element=w560, error in (no error)=w563) -> (error out=w565:errorcluster)  [unwired: 1 in, 2 out]
                  n225 = Wait on Notification(notifier=w562, error in (no error)=w565) -> (error out=w564:errorcluster)  [unwired: 2 in, 3 out]
                }
              }
              n226 = Equal To 0?(x=w531) -> (x = 0?=w552:bool)
              n227 = Equal To 0?(x=w530) -> (x = 0?=w551:bool)
              n228 = Get Date/Time In Seconds() -> (seconds since 1Jan1904=w523:timestamp)
              n229 = And(x=w552, y=w551) -> (x .and. y?=w550:bool)
              n230 = Enqueue Element(queue=w525, element="snap", error in (no error)=w548) -> (error out=w547:errorcluster)  [unwired: 1 in, 2 out]
              n231 = call "createFileStruc.vi"("i_iter"=w530, "i_delay"=w531, "meas_path"=w532) -> ("AVG file"=w527:path, "RAW file"=w519:path)  [unwired: 7 in]
              n232 = Dequeue Element(queue=w553, error in (no error)=w547) -> (element=w529:dbl[][], error out=w520:errorcluster)  [unwired: 1 in, 2 out]
              n233 = Strip Path(path=w519) -> (name=w518:string)  [unwired: 1 out]
              n234 = Array Size(array=w529) -> (size(s)=w557:i32[])
              n235 = call-poly <vilib>:"Write Delimited Spreadsheet.vi"("file path (dialog if empty)"=w519, "2D data"=w529, "error in (no error)"=w520) -> ()  [unwired: 11 in, 2 out]
              n236 = Index Array(array=w557) -> (element #1=w555:i32, element #2=w554:i32)  [unwired: 2 in]
              n237 = Subtract(x=w523, y=w533) -> (x-y=w536:dbl)
              n238 = flat-sequence {
                tunnel: "%s\\t%<%Y.%m.%d %H:%M:%S>T\\t%f\\t%f\\t%f\\t%f\\t%f\\t%f\\t%f\\t%f\\t%f\\t%f\\t%f\\t%f\\t%f\\t%f\\t%f\\t%f\\t%f\\t%f\\t%f" -> [w595]
                tunnel: w523 -> [w594]
                tunnel: w522 -> [w571]
                tunnel: [w570] -> w521
                tunnel: w520 -> [w567]
                tunnel: w518 -> [w566]
                frame #0 {
                  n239 = local read "pos"() -> (w596:dbl[])
                  n240 = local read "mirr_posX"() -> (w583:i32)
                  n241 = local read "mirr_posY"() -> (w584:i32)
                  n242 = local read "ESP_delay"() -> (w576:dbl)
                  n243 = local read "phoib_I_1"() -> (w585:dbl)
                  n244 = local read "phoib_I_2"() -> (w586:dbl)
                  n245 = local read "phoib_I_3"() -> (w587:dbl)
                  n246 = local read "phoib_I_4"() -> (w588:dbl)
                  n247 = local read "phoib_I_5"() -> (w589:dbl)
                  n248 = local read "phoib_I_6"() -> (w590:dbl)
                  n249 = local read "phoib_I_7"() -> (w591:dbl)
                  n250 = local read "phoib_I_8"() -> (w592:dbl)
                  n251 = local read "phoib_I_9"() -> (w593:dbl)
                  n252 = local read "ESP_pos"() -> (w575:dbl)
                  n253 = Index Array(array=w596) -> (element #1=w577:dbl, element #2=w578:dbl, element #3=w579:dbl, element #4=w580:dbl, element #5=w581:dbl, element #6=w582:dbl)  [unwired: 6 in]
                  n254 = Format Into String(format string=w595, error in=w567, w566, w594, w575, w576, w577, w578, w579, w580, w581, w582, w583, w584, w585, w586, w587, w588, w589, w590, w591, w592, w593) -> (resulting string=w573:string)  [unwired: 1 in, 1 out]
                  n255 = Spreadsheet String To Array(format string="%s", spreadsheet string=w573, array type (2D Dbl)=string[] []) -> (array=w569:string[])  [unwired: 1 in]
                  n256 = call-poly <vilib>:"Write Delimited Spreadsheet.vi"("file path (dialog if empty)"=w571, "1D data"=w569, "append to file? (F)"=TRUE) -> ("new file path (Not A Path if cancelled)"=w570:path)  [unwired: 11 in, 1 out]
                }
              }
              n257 = case shown="True" w550 {
                tunnel: w534 -> [_ w602]
                tunnel: [w597 w600] -> w556
                tunnel: w549 -> [w597 _]
                tunnel: w555 -> [_ w599]
                tunnel: w554 -> [_ w598]
                frame False {
                }
                frame True {
                  n258 = Initialize Array(0.0 ("element"), w602, w599, w598) -> (w600:dbl[][][])
                }
              }
              n259 = Increment(x=w531) -> (x+1=w540:i32)
              "current scan" <- w540
              n260 = Increment(x=w530) -> (x+1=w539:i32)
              "current iteration" <- w539
              n261 = for {
                N: w555 -> [_]
                tunnel: w531 -> [w609]
                shift-right: [w607] -> w544
                shift-left: w556 -> [w610]
                tunnel: w530 -> [w605]
                shift-right: [w604] -> w528
                shift-left: w529 -> [w606]
                tunnel: w554 -> [w603]
                i -> [w608]
                n262 = for {
                  N: w603 -> [_]
                  tunnel: w609 -> [w617]
                  tunnel: w608 -> [w614]
                  shift-right: [w616] -> w607
                  shift-left: w610 -> [w618]
                  tunnel: w605 -> [w612]
                  shift-right: [w611] -> w604
                  shift-left: w606 -> [w615]
                  i -> [w613]
                  n263 = in-place {
                    in-place-border: w612 -> [w624]
                    n264 = in-place-array #1(w618, w617, w614, w613) -> (w625:dbl)
                    n265 = in-place-array #2(w615, w614, w613) -> (w622:dbl)
                    n266 = Multiply(x=w625, y=w624) -> (x*y=w623:dbl)
                    n267 = Increment(x=w624) -> (x+1=w620:i32)
                    n268 = Add(x=w623, y=w622) -> (x+y=w621:dbl)
                    n269 = Divide(x=w621, y=w620) -> (x/y=w619:dbl)
                    n270 = in-place-array #1(w619) -> (w616:dbl[][][])  [unwired: 3 out]
                    n271 = in-place-array #2(w619) -> (w611:dbl[][])  [unwired: 2 out]
                  }
                }
              }
              n272 = Multiply(x=w534, y=w530) -> (x*y=w535:i32)
              n273 = Multiply(x=w534, y=w513) -> (x*y=w499:i32)
              n274 = Divide(x=w540, y=w534) -> (x/y=→"scan 2":dbl)
              n275 = Divide(x=w539, y=w513) -> (x/y=→"iteration":dbl)
              n276 = Add(x=w531, y=w535) -> (x+y=w502:i32)
              n277 = Multiply(x=w504, y=w499) -> (x*y=w503:i32)
              n278 = Add(x=w502, y=w503) -> (x+y=w501:i32)
              n279 = Divide(x=w536, y=w501) -> (x/y=w509:dbl)
              n280 = Multiply(x=w500, y=w499) -> (x*y=w498:i32)
              n281 = Multiply(x=w509, y=w498) -> (x*y=w512:dbl)
              n282 = local write "duration [HH:MM:SS]"(w512) -> ()
              n283 = local write "time/step [s]"(w509) -> ()
              n284 = property on="mainimg" class="IntGraph (strict)"() -> ("CrsrLis"=w543:T5)  [unwired: 2 in, 2 out]
              n285 = call-poly <vilib>:"Write Delimited Spreadsheet.vi"("file path (dialog if empty)"=w527, "2D data"=w528) -> ()  [unwired: 12 in, 2 out]
              n286 = call "processData.vi"("Cursor List"=w543, "data in"=w544) -> ("Angle Chart"=→"anglegraph":dbl[][], "Energy Chart"=→"energygraph":dbl[][], "Intensity Chart"=w542:dbl[])  [unwired: 1 in]
              n287 = Bundle("Array"=w517, "Intensity Chart"=w542) -> (→"intensitygraph":cluster{"Array":dbl[], "Intensity Chart":dbl[]})  [unwired: 1 in]
              n288 = Or(x="stop after iteration", y="stop after step") -> (x .or. y?=w514:bool)
            }
            n289 = Increment(x=w484) -> (x+1=w482:i32)
            n290 = Greater Or Equal?(x=w482, y=w483) -> (x >= y?=w479:bool)
            n291 = Or(x=w480, y=w479) -> (x .or. y?=w481:bool)
          }
        }
      }
      frame "refresh" {
        n292 = Dequeue Element(queue=w626) -> ()  [unwired: 2 in, 4 out]
        n293 = property on="mainimg" class="IntGraph (strict)"() -> ("CrsrLis"=w633:T5)  [unwired: 2 in, 2 out]
        n294 = call "processData.vi"("Cursor List"=w633, "data in"=w632) -> ("Angle Chart"=w630:dbl[][], "Energy Chart"=w631:dbl[][], "Intensity Chart"=w627:dbl[])  [unwired: 1 in]
        n295 = Bundle("Array"=w628, "Intensity Chart"=w627) -> (w629:cluster{"Array":dbl[], "Intensity Chart":dbl[]})  [unwired: 1 in]
        n296 = local write "energygraph"(w631) -> ()
        n297 = local write "intensitygraph"(w629) -> ()
        n298 = local write "anglegraph"(w630) -> ()
      }
    }
  }
  n299 = while {
    tunnel: w23 -> [w642]
    tunnel: w22 -> [w641]
    tunnel: w21 -> [w640]
    tunnel: w20 -> [w639]
    tunnel: w25 -> [w637]
    tunnel: w32 -> [w638]
    tunnel: w6 -> [w636]
    tunnel: w13 -> [w635]
    tunnel: w7 -> [w634]
    stop <- w643 stop-if-true
    n300 = event shown="[6] \"wattpilot_set\": Value Change" {
      selector: _ -> [_ _ _ _ _ _ _ _ _ _ _ _ _ _ _ _ _ _ _ _ _ _ _ _ _ _ _ _ _ _ _ _ _ _ _ _]
      dyn-events: _ -> [_ _ _ _ _ _ _ _ _ _ _ _ _ _ _ _ _ _ _ _ _ _ _ _ _ _ _ _ _ _ _ _ _ _ _ _]
      timeout: _ -> [_ _ _ _ _ _ _ _ _ _ _ _ _ _ _ _ _ _ _ _ _ _ _ _ _ _ _ _ _ _ _ _ _ _ _ _]
      tunnel: [_ TRUE _ _ _ _ _ _ _ _ _ _ _ _ _ _ _ _ _ _ _ _ _ _ _ _ _ _ _ _ _ _ _ _ _ _] -> w643
      tunnel: w642 -> [_ w658 w670 _ _ _ _ _ _ _ w700 w702 _ _ _ _ _ _ _ _ _ _ _ _ _ _ _ _ _ _ _ _ _ _ _ _]
      tunnel: w641 -> [_ w657 _ w674 _ _ _ _ _ _ _ _ _ _ _ _ _ _ _ _ _ _ _ w781 _ _ w803 _ _ _ _ _ _ _ _ _]
      tunnel: w640 -> [_ w656 _ _ w680 _ _ _ _ _ _ _ _ _ _ _ _ _ _ _ w755 w771 w773 _ _ _ _ _ _ _ _ _ _ _ _ _]
      tunnel: w639 -> [_ w655 _ _ _ _ _ w690 w696 w697 _ _ _ _ _ _ _ _ _ _ _ _ _ _ _ _ _ _ _ _ _ _ _ _ _ _]
      tunnel: w638 -> [_ w663 _ _ _ _ _ _ _ _ _ _ _ _ _ _ _ _ _ _ _ _ _ _ _ _ _ _ _ _ _ _ _ _ _ _]
      tunnel: w637 -> [_ w654 _ _ _ _ _ _ _ _ _ _ w704 w706 _ _ _ _ _ _ _ _ _ _ _ _ _ _ _ _ _ _ _ w827 _ _]
      tunnel: w636 -> [_ w662 _ _ _ _ _ _ _ _ _ _ _ _ _ _ _ _ _ _ _ _ _ _ _ _ _ _ _ _ _ _ _ _ _ _]
      tunnel: w635 -> [_ w653 _ _ _ _ _ _ _ _ _ _ _ _ _ w729 _ _ _ _ _ _ _ _ _ _ _ _ _ _ _ _ _ _ w829 w850]
      tunnel: w634 -> [_ w646 _ _ _ _ _ _ _ _ _ _ _ _ _ _ _ _ _ _ _ _ _ _ _ _ _ _ _ _ _ _ _ _ _ _]
      event Timeout {
        n301 = event-data() -> ()  [unwired: 1 in, 1 out]
      }
      event "main_close": Value Change {
        w644 = "close" ("element")
        w659 = "release" ("element")
        n302 = event-data() -> ()  [unwired: 1 in, 1 out]
        n303 = Flush Queue(queue=w658) -> (queue out=w652:refnum<queue>)  [unwired: 1 in, 2 out]
        n304 = Flush Queue(queue=w657) -> (queue out=w651:refnum<queue>)  [unwired: 1 in, 2 out]
        n305 = Flush Queue(queue=w656) -> (queue out=w650:refnum<queue>)  [unwired: 1 in, 2 out]
        n306 = Flush Queue(queue=w655) -> (queue out=w649:refnum<queue>)  [unwired: 1 in, 2 out]
        n307 = Flush Queue(queue=w654) -> (queue out=w648:refnum<queue>)  [unwired: 1 in, 2 out]
        n308 = Flush Queue(queue=w653) -> (queue out=w647:refnum<queue>)  [unwired: 1 in, 2 out]
        n309 = Flush Queue(queue=w646) -> (queue out=w645:refnum<queue>)  [unwired: 1 in, 2 out]
        n310 = Release Notifier(notifier=w662) -> ()  [unwired: 2 in, 3 out]
        n311 = Release Queue(queue=w663) -> ()  [unwired: 2 in, 3 out]
        n312 = Enqueue Element(queue=w652, element=w659) -> (queue out=w667:refnum<queue>)  [unwired: 2 in, 2 out]
        n313 = Enqueue Element(queue=w651, element=w659) -> (queue out=w666:refnum<queue>)  [unwired: 2 in, 2 out]
        n314 = Enqueue Element(queue=w650, element=w659) -> (queue out=w665:refnum<queue>)  [unwired: 2 in, 2 out]
        n315 = Enqueue Element(queue=w649, element=w659) -> (queue out=w664:refnum<queue>)  [unwired: 2 in, 2 out]
        n316 = Enqueue Element(queue=w647, element=w659) -> (queue out=w661:refnum<queue>, error out=w660:errorcluster)  [unwired: 2 in, 1 out]
        n317 = Enqueue Element(queue=w667, element=w644) -> ()  [unwired: 2 in, 3 out]
        n318 = Enqueue Element(queue=w666, element=w644) -> ()  [unwired: 2 in, 3 out]
        n319 = Enqueue Element(queue=w665, element=w644) -> ()  [unwired: 2 in, 3 out]
        n320 = Enqueue Element(queue=w664, element=w644) -> ()  [unwired: 2 in, 3 out]
        n321 = Enqueue Element(queue=w648, element=w644) -> ()  [unwired: 2 in, 3 out]
        n322 = Enqueue Element(queue=w661, element=w644, error in (no error)=w660) -> ()  [unwired: 1 in, 3 out]
        n323 = Enqueue Element(queue=w645, element=w644) -> ()  [unwired: 2 in, 3 out]
      }
      event "cam_release", "cam_init": Value Change {
        n324 = event-data() -> ()  [unwired: 1 in, 2 out]
        n325 = Select(t="init" ("name (unnamed)"), s="cam_init", f="release" ("name (unnamed)")) -> (s? t:f=w669:string)
        n326 = Enqueue Element(queue=w670, element=w669) -> ()  [unwired: 2 in, 3 out]
      }
      event "ESP_release", "ESP_init": Value Change {
        n327 = event-data() -> ()  [unwired: 1 in, 2 out]
        n328 = Select(t="init" ("name (unnamed)"), s="ESP_init", f="release" ("name (unnamed)")) -> (s? t:f=w678:string)
        n329 = Enqueue Element(queue=w674, element=w678) -> ()  [unwired: 2 in, 3 out]
      }
      event "manip_init", "manip_release": Value Change {
        n330 = event-data() -> ()  [unwired: 1 in, 2 out]
        n331 = Flush Queue(queue=w680) -> (queue out=w679:refnum<queue>)  [unwired: 1 in, 2 out]
        n332 = Select(t="init" ("name (unnamed)"), s="manip_init", f="release" ("name (unnamed)")) -> (s? t:f=w682:string)
        n333 = Enqueue Element(queue=w679, element=w682) -> ()  [unwired: 2 in, 3 out]
      }
      event "setpoint_set": Value Change {
        n334 = event-data() -> ()  [unwired: 1 in, 2 out]
        n335 = local read "LS310  EPICS SP"() -> (w686:string)
        n336 = call-poly <userlib>:"CaLabPut.vi"("Value"="Setpoint", "PV Name"=w686) -> ()  [unwired: 6 in, 4 out]
      }
      event "wattpilot_set": Value Change {
        n337 = event-data() -> ()  [unwired: 1 in, 2 out]
        n338 = local read "WattPilot EPICS chanel set"() -> (w688:string)
        n339 = call-poly <userlib>:"CaLabPut.vi"("Value"="Set Powet (%)", "PV Name"=w688) -> ()  [unwired: 6 in, 4 out]
      }
      event "phoib_release", "phoib_init": Value Change {
        n340 = event-data() -> ()  [unwired: 1 in, 2 out]
        n341 = Flush Queue(queue=w690) -> (queue out=w689:refnum<queue>)  [unwired: 1 in, 2 out]
        n342 = Select(t="init" ("name (unnamed)"), s="phoib_init", f="release" ("name (unnamed)")) -> (s? t:f=w692:string)
        n343 = Enqueue Element(queue=w689, element=w692) -> ()  [unwired: 2 in, 3 out]
      }
      event "phoib_standby": Value Change {
        n344 = event-data() -> ()  [unwired: 1 in, 2 out]
        n345 = Enqueue Element(queue=w696, element="standby") -> ()  [unwired: 2 in, 3 out]
      }
      event "phoib_set": Value Change {
        n346 = event-data() -> ()  [unwired: 1 in, 2 out]
        n347 = Enqueue Element(queue=w697, element="set") -> ()  [unwired: 2 in, 3 out]
      }
      event "cam_dark": Value Change {
        n348 = event-data() -> ()  [unwired: 1 in, 2 out]
        n349 = Enqueue Element(queue=w700, element="dark") -> ()  [unwired: 2 in, 3 out]
      }
      event "ROI Left", "ROI Right", "ROI Top", "ROI Bottom", "cam_exp", "binning", "gain": Value Change {
        n350 = event-data() -> ()  [unwired: 1 in, 1 out]
        n351 = Enqueue Element(queue=w702, element="set") -> ()  [unwired: 2 in, 3 out]
      }
      event "cam_saveimg": Value Change {
        n352 = event-data() -> ()  [unwired: 1 in, 1 out]
        n353 = Enqueue Element(queue=w704, element="single") -> ()  [unwired: 2 in, 3 out]
      }
      event "scan_go": Value Change {
        n354 = event-data() -> ()  [unwired: 1 in, 1 out]
        n355 = Enqueue Element(queue=w706, element="scan") -> ()  [unwired: 2 in, 3 out]
      }
      event "meas_iter", "waypointsD1", "waypointsD2": Value Change {
        n356 = event-data() -> ()  [unwired: 1 in, 6 out]
        n357 = local read "waypointsD2"() -> (w717:string[][])
        n358 = local read "waypointsD1"() -> (w727:string[][])
        n359 = call "create scan vectr.vi"("Table Control"=w717) -> ("Array"=w716:dbl[])
        n360 = call "create scan vectr.vi"("Table Control"=w727) -> ("Array"=w726:dbl[])
        n361 = Array Size(array=w716) -> (size(s)=w714:i32)
        n362 = Array Size(array=w726) -> (size(s)=w710:i32)
        n363 = local read "meas_iter"() -> (w722:i32)
        n364 = local read "binning"() -> (w724:u16)
        n365 = Equal To 0?(x=w714) -> (x = 0?=w715:bool)
        n366 = Select(t=1, s=w715, f=w714) -> (s? t:f=w712:i32)
        n367 = Index Array(array=dbl[] [8.79, 2.2, 0.553, 0.138], index=w724) -> (element=w721:dbl)
        n368 = Multiply(x=w712, y=w710) -> (x*y=w711:i32)
        "measpoints" <- w711
        n369 = Multiply(x=w711, y=w722) -> (x*y=w719:i32)
        "total steps" <- w719
        n370 = Get Date/Time In Seconds() -> (seconds since 1Jan1904=w709:timestamp)
        n371 = Multiply(x=w719, y=w721) -> (x*y=→"disk [MB]":dbl)
        n372 = Multiply(x=w719, y="time/step [s]") -> (x*y=w708:dbl)
        "duration [HH:MM:SS]" <- w708
        n373 = Multiply(x=w710, y=w721) -> (x*y=→"RAM [MB]":dbl)
        n374 = Add(x=w709, y=w708) -> (x+y=→"ETA 2":timestamp)
      }
      event "mirr_go": Value Change {
        n375 = event-data() -> ()  [unwired: 1 in, 1 out]
        n376 = Index Array(array="mirr_dest") -> (element #1=w734:i32, element #2=w733:i32)  [unwired: 2 in]
        n377 = Format Into String(format string="%g_%g", w734, w733) -> (resulting string=w731:string)  [unwired: 2 in, 1 out]
        n378 = Concatenate Strings("abs:" ("string"), w731) -> (w728:string)
        n379 = Enqueue Element(queue=w729, element=w728) -> ()  [unwired: 2 in, 3 out]
      }
      event "scan_manip_setstart": Value Change {
        n380 = event-data() -> ()  [unwired: 1 in, 1 out]
        n381 = local read "pos"() -> (w736:dbl[])
        n382 = local write "scan_manip_start"(w736) -> ()
      }
      event "scan_manip_setstart 2": Value Change {
        n383 = event-data() -> ()  [unwired: 1 in, 1 out]
        n384 = local read "pos"() -> (w737:dbl[])
        n385 = local write "scan_manip_start 2"(w737) -> ()
      }
      event "scan_mirr_setstart": Value Change {
        n386 = event-data() -> ()  [unwired: 1 in, 1 out]
        n387 = local read "mirr_posX"() -> (w740:i32)
        n388 = local read "mirr_posY"() -> (w739:i32)
        n389 = Build Array(w740, w739) -> (w738:i32[])
        n390 = local write "scan_mirr_start"(w738) -> ()
      }
      event "scan_mirr_setstart 2": Value Change {
        n391 = event-data() -> ()  [unwired: 1 in, 1 out]
        n392 = local read "mirr_posX"() -> (w743:i32)
        n393 = local read "mirr_posY"() -> (w742:i32)
        n394 = Build Array(w743, w742) -> (w741:i32[])
        n395 = local write "scan_mirr_start 2"(w741) -> ()
      }
      event "Move Abs": Value Change {
        n396 = event-data() -> ()  [unwired: 1 in, 1 out]
        n397 = Index Array(array="dest") -> (element #1=w753:dbl, element #2=w752:dbl, element #3=w751:dbl, element #4=w750:dbl, element #5=w749:dbl, element #6=w748:dbl)  [unwired: 6 in]
        n398 = Format Into String(format string="%g_%g_%g_%g_%g_%g", w753, w752, w751, w750, w749, w748) -> (resulting string=w746:string)  [unwired: 2 in, 1 out]
        n399 = Concatenate Strings("abs:" ("string"), w746) -> (w745:string)
        n400 = Enqueue Element(queue=w755, element=w745) -> ()  [unwired: 2 in, 3 out]
      }
      event "ManipRel +", "ManipRel -": Value Change {
        n401 = event-data() -> ()  [unwired: 1 in, 2 out]
        n402 = Negate(x="manip_deltas") -> (-x=w759:dbl[])
        n403 = Select(t="manip_deltas", s="ManipRel +", f=w759) -> (s? t:f=w757:dbl[])
        n404 = Index Array(array=w757) -> (element #1=w763:dbl, element #2=w764:dbl, element #3=w765:dbl, element #4=w766:dbl, element #5=w767:dbl, element #6=w768:dbl)  [unwired: 6 in]
        n405 = Format Into String(format string="%g_%g_%g_%g_%g_%g", w763, w764, w765, w766, w767, w768) -> (resulting string=w770:string)  [unwired: 2 in, 1 out]
        n406 = Concatenate Strings("rel:" ("string"), w770, ":wait" ("string")) -> (w761:string)
        n407 = Enqueue Element(queue=w771, element=w761) -> ()  [unwired: 2 in, 3 out]
      }
      event "stop manip": Value Change {
        n408 = event-data() -> ()  [unwired: 1 in, 1 out]
        n409 = Enqueue Element(queue=w773, element="stop") -> ()  [unwired: 2 in, 3 out]
      }
      event "ESP_go": Value Change {
        w775 = ":" ("string")
        n410 = event-data() -> ()  [unwired: 1 in, 1 out]
        n411 = Number To Decimal String(number=0) -> (decimal integer string=w777:string)  [unwired: 1 in]
        n412 = Number To Fractional String(number="ESP_dest") -> (F-format string=w776:string)  [unwired: 3 in]
        n413 = Concatenate Strings("abs:" ("string"), w777, w775, w776, w775) -> (w780:string)
        n414 = Enqueue Element(queue=w781, element=w780) -> ()  [unwired: 2 in, 3 out]
      }
      event "ESP_set_t0": Value Change {
        n415 = event-data() -> ()  [unwired: 1 in, 1 out]
        n416 = Current VI's Path() -> (path=w792:path)
        n417 = Strip Path(path=w792) -> (stripped path=w790:path)  [unwired: 1 out]
        n418 = Strip Path(path=w790) -> (stripped path=w789:path)  [unwired: 1 out]
        n419 = local read "ESP_pos"() -> (w791:dbl)
        "ESP_t0" <- w791
        n420 = Number To Fractional String(number=w791) -> (F-format string=w784:string)  [unwired: 3 in]
        n421 = Build Path(base path=w789, name or relative path="t0.txt") -> (appended path=w786:path)
        n422 = Get Date/Time In Seconds() -> (seconds since 1Jan1904=w788:timestamp)
        n423 = Format Date/Time String(time format string (%c)="%Y.%m.%d %H:%M", seconds (now)=w788) -> (date/time string=w785:string)  [unwired: 1 in]
        n424 = Build Array(w785, w784) -> (w783:string[])
        n425 = call-poly <vilib>:"Write Delimited Spreadsheet.vi"("file path (dialog if empty)"=w786, "1D data"=w783, "append to file? (F)"=TRUE) -> ()  [unwired: 11 in, 2 out]
      }
      event "ESP_opent0file": Value Change {
        n426 = event-data() -> ()  [unwired: 1 in, 6 out]
        n427 = Current VI's Path() -> (path=w796:path)
        n428 = Strip Path(path=w796) -> (stripped path=w795:path)  [unwired: 1 out]
        n429 = Strip Path(path=w795) -> (stripped path=w797:path)  [unwired: 1 out]
        n430 = call <vilib>:"System Exec.vi"("wait until completion? (T)"=FALSE, "working directory"=w797, "command line"="notepad t0.txt") -> ()  [unwired: 5 in, 4 out]
      }
      event "ESP_+", "ESP_-": Value Change {
        n431 = event-data() -> ()  [unwired: 1 in, 6 out]
        n432 = Negate(x="ESP_delta") -> (-x=w806:dbl)
        n433 = Select(t="ESP_delta", s="ESP_+", f=w806) -> (s? t:f=w804:dbl)
        n434 = Number To Decimal String(number=0) -> (decimal integer string=w802:string)  [unwired: 1 in]
        n435 = Number To Fractional String(number=w804) -> (F-format string=w800:string)  [unwired: 3 in]
        n436 = Concatenate Strings("rel:" ("string"), w802, ":" ("string"), w800) -> (w809:string)
        n437 = Enqueue Element(queue=w803, element=w809) -> ()  [unwired: 2 in, 3 out]
      }
      event "ESP_dest": Value Change {
        n438 = event-data() -> ()  [unwired: 1 in, 6 out]
        n439 = local read "ESP_dest"() -> (w813:dbl)
        n440 = local read "ESP_t0"() -> (w812:dbl)
        n441 = call "mm2time.vi"("fs?"=TRUE ("fs[1]/ps[0]"), "Offset (mm)"=w812, "distance (mm)"=w813) -> ("time in fs/ps seconds"=w810:dbl)
        n442 = local write "ESP_dest_t"(w810) -> ()
      }
      event "ESP_dest_t": Value Change {
        n443 = event-data() -> ()  [unwired: 1 in, 1 out]
        n444 = local read "ESP_t0"() -> (w816:dbl)
        n445 = call "time2mm.vi"("fs[1]/ps[0]"=TRUE, "Offset (mm)"=w816, "time"="ESP_dest_t") -> ("position (mm)"=w814:dbl)
        n446 = local write "ESP_dest"(w814) -> ()
      }
      event "load waypoints 1": Value Change {
        n447 = event-data() -> ()  [unwired: 1 in, 6 out]
        n448 = call-poly <vilib>:"Read Delimited Spreadsheet.vi"() -> ("all rows"=w819:string[][], "error out"=w818:errorcluster)  [unwired: 10 in, 4 out]
        n449 = case shown="No Error" w818 {
          tunnel: w819 -> [w820 _]
          frame No Error {
            n450 = local write "waypointsD1"(w820) -> ()
          }
          frame Error {
          }
        }
      }
      event "load waypoints 2": Value Change {
        n451 = event-data() -> ()  [unwired: 1 in, 6 out]
        n452 = call-poly <vilib>:"Read Delimited Spreadsheet.vi"() -> ("all rows"=w822:string[][], "error out"=w821:errorcluster)  [unwired: 10 in, 4 out]
        n453 = case shown="No Error" w821 {
          tunnel: w822 -> [w823 _]
          frame No Error {
            n454 = local write "waypointsD2"(w823) -> ()
          }
          frame Error {
          }
        }
      }
      event "clear waypoints 1": Value Change {
        n455 = event-data() -> ()  [unwired: 1 in, 6 out]
        n456 = local write "waypointsD1"(string[][] []) -> ()
      }
      event "clear waypoints 2": Value Change {
        n457 = event-data() -> ()  [unwired: 1 in, 6 out]
        n458 = local write "waypointsD2"(string[][] []) -> ()
      }
      event "mainimg": Cursor Release {
        n459 = event-data() -> ()  [unwired: 1 in, 1 out]
        n460 = Enqueue Element(queue=w827, element="refresh") -> ()  [unwired: 2 in, 3 out]
      }
      event "mirr_init", "mirr_release": Value Change {
        n461 = event-data() -> ()  [unwired: 1 in, 6 out]
        n462 = Flush Queue(queue=w829) -> (queue out=w830:refnum<queue>)  [unwired: 1 in, 2 out]
        n463 = Select(t="init" ("name (unnamed)"), s="mirr_init", f="release" ("name (unnamed)")) -> (s? t:f=w831:string)
        n464 = Enqueue Element(queue=w830, element=w831) -> ()  [unwired: 2 in, 3 out]
      }
      event "mirr_X-", "mirr_X+", "mirr_Y+", "mirr_Y-": Value Change {
        n465 = event-data() -> ()  [unwired: 1 in, 1 out]
        n466 = local read "mirr_X#"() -> (w841:u8)
        n467 = local read "mirr_Y#"() -> (w840:u8)
        n468 = Or(x="mirr_X+", y="mirr_X-") -> (x .or. y?=w842:bool)
        n469 = Or(x="mirr_X-", y="mirr_Y-") -> (x .or. y?=w848:bool)
        n470 = Negate(x="mirr_rel") -> (-x=w847:i32)
        n471 = Select(t=w841, s=w842, f=w840) -> (s? t:f=w839:u8)
        n472 = Select(t=w847, s=w848, f="mirr_rel") -> (s? t:f=w836:i32)
        n473 = Number To Decimal String(number=w839) -> (decimal integer string=w838:string)  [unwired: 1 in]
        n474 = Number To Decimal String(number=w836) -> (decimal integer string=w835:string)  [unwired: 1 in]
        n475 = Concatenate Strings("rel:" ("string"), w838, ":" ("string"), w835) -> (w834:string)
        n476 = Enqueue Element(queue=w850, element=w834) -> ()  [unwired: 2 in, 3 out]
      }
    }
  }
  n477 = while {
    tunnel: w13 -> [w859]
    shift-right: [w856] -> _
    shift-left: _ -> [w857]
    tunnel: w6 -> [w855]
    shift-right: [w854] -> _
    shift-left: _ -> [w853]
    shift-right: [w851] -> _
    shift-left: _ -> [w852]
    stop <- w858 stop-if-true
    # "mirr"
    n478 = Preview Queue Element(queue=w859, timeout in ms (-1)=w857) -> (queue out=w862:refnum<queue>, element=w863:string)  [unwired: 1 in, 2 out]
    n479 = Match Pattern(string=w863, regular expression=":") -> (before substring=w861:string, after substring=w860:string)  [unwired: 1 in, 2 out]
    n480 = case shown="\"idle\", Default" w861 {
      tunnel: w862 -> [w898 w908 w923 w927 w930 w935 _]
      tunnel: w860 -> [w892 w909 _ _ _ _ _]
      tunnel: [_ _ _ TRUE _ _ _] -> w858
      tunnel: [_ _ _ _ -1 _ _] -> w856
      tunnel: w855 -> [w865 _ _ _ _ _ _]
      tunnel: [w884 w905 refnum<visa-resource-name> refnum ("VISA resource name out") w925 w929 w934 w940] -> w854
      tunnel: w853 -> [w897 w907 w922 w925 w929 _ w944]
      tunnel: [w869 w904 w921 w924 w928 w933 w939] -> w851
      tunnel: w852 -> [w896 w906 _ w924 w928 _ w943]
      frame "abs" {
        w880 = u8 20 items=["Echo"=55, "Home"=1, "Move Absolute"=20, "Move Relative"=21, "Move at Constant Speed"=22, "Renumber"=2, "Restore Settings"=36, "Stop"=23] ("Command")
        w895 = u8 20 items=["Echo"=55, "Home"=1, "Move Absolute"=20, "Move Relative"=21, "Move at Constant Speed"=22, "Renumber"=2, "Restore Settings"=36, "Stop"=23] ("Command")
        n481 = Dequeue Element(queue=w898) -> ()  [unwired: 2 in, 4 out]
        n482 = Match Pattern(string=w892, regular expression=":") -> (before substring=w882:string, after substring=w868:string)  [unwired: 1 in, 2 out]
        n483 = Equal?(x=w868, y="wait") -> (x = y?=w866:bool)
        n484 = Scan From String(format string="%g_%g", input string=w882) -> (output 1=w877:dbl, output 2=w876:dbl)  [unwired: 4 in, 3 out]
        n485 = local read "mirr_X#"() -> (w879:u8)
        n486 = Bundle("mirr_X#"=w879, "Command"=w895, w877, "Response Count"=1) -> (w891:T6)  [unwired: 1 in]
        n487 = local read "mirr_Y#"() -> (w878:u8)
        n488 = call "Request Command.vi"("error in (no error)"=w896, "Request"=w891, "VISA resource name"=w897) -> ("error out"=w873:errorcluster, "VISA resource name out"=w874:refnum<visa-resource-name>)  [unwired: 5 in, 2 out]
        n489 = Bundle("mirr_Y#"=w878, "Command"=w880, w876, "Response Count"=1) -> (w875:T7)  [unwired: 1 in]
        n490 = call "Request Command.vi"("error in (no error)"=w873, "Request"=w875, "VISA resource name"=w874) -> ("error out"=w871:errorcluster, "VISA resource name out"=w872:refnum<visa-resource-name>)  [unwired: 5 in, 2 out]
        n491 = local read "mirr_X#"() -> (w889:u8)
        n492 = call "zaber_readpos.vi"("error in (no error)"=w871, "axis"=w889, "VISA in"=w872) -> ("error out"=w885:errorcluster, "position"=w890:i32, "VISA out"=w886:refnum<visa-resource-name>)  [unwired: 6 in]
        n493 = local read "mirr_Y#"() -> (w887:u8)
        n494 = local write "mirr_posX"(w890) -> ()
        n495 = call "zaber_readpos.vi"("error in (no error)"=w885, "axis"=w887, "VISA in"=w886) -> ("error out"=w870:errorcluster, "position"=w888:i32, "VISA out"=w884:refnum<visa-resource-name>)  [unwired: 6 in]
        n496 = local write "mirr_posY"(w888) -> ()
        n497 = case shown="True" w866 {
          tunnel: w870 -> [w899 w903]
          tunnel: [w899 w902] -> w869
          tunnel: w865 -> [_ w901]
          frame False {
          }
          frame True {
            n498 = Send Notification(notification=TRUE, notifier=w901, error in (no error)=w903) -> (error out=w902:errorcluster)  [unwired: 1 out]
          }
        }
      }
      frame "rel" {
        w912 = u8 21 items=["Echo"=55, "Home"=1, "Move Absolute"=20, "Move Relative"=21, "Move at Constant Speed"=22, "Renumber"=2, "Restore Settings"=36, "Stop"=23] ("Command")
        n499 = Dequeue Element(queue=w908) -> ()  [unwired: 2 in, 4 out]
        n500 = Match Pattern(string=w909, regular expression=":") -> (before substring=w914:string, after substring=w913:string)  [unwired: 1 in, 2 out]
        n501 = Decimal String To Number(string=w914) -> (number=w916:i32)  [unwired: 2 in, 1 out]
        n502 = Decimal String To Number(string=w913) -> (number=w917:i32)  [unwired: 2 in, 1 out]
        n503 = Bundle(w916, "Command"=w912, w917, "Response Count"=1) -> (w910:T8)  [unwired: 1 in]
        n504 = call "Request Command.vi"("error in (no error)"=w906, "Request"=w910, "VISA resource name"=w907) -> ("error out"=w904:errorcluster, "VISA resource name out"=w905:refnum<visa-resource-name>)  [unwired: 5 in, 2 out]
      }
      frame "release" {
        n505 = Dequeue Element(queue=w923) -> (queue out=w919:refnum<queue>)  [unwired: 2 in, 3 out]
        n506 = Enqueue Element(queue=w919, element="suspend") -> ()  [unwired: 2 in, 3 out]
        n507 = call "Close.vi"("VISA resource name"=w922) -> ("error out"=w921:errorcluster)  [unwired: 9 in, 1 out]
      }
      frame "close" {
        n508 = Release Queue(queue=w927) -> ()  [unwired: 2 in, 3 out]
      }
      frame "suspend" {
        n509 = Dequeue Element(queue=w930) -> ()  [unwired: 2 in, 4 out]
      }
      frame "init" {
        n510 = Dequeue Element(queue=w935) -> ()  [unwired: 2 in, 4 out]
        n511 = call "Initialize.vi"("VISA resource name"="mirr_VISA") -> ("error out"=w933:errorcluster, "VISA resource name out"=w934:refnum<visa-resource-name>)  [unwired: 8 in, 1 out]
      }
      frame "idle", Default {
        n512 = local read "mirr_X#"() -> (w945:u8)
        n513 = call "zaber_readpos.vi"("error in (no error)"=w943, "axis"=w945, "VISA in"=w944) -> ("error out"=w941:errorcluster, "position"=→"mirr_posX":i32, "VISA out"=w942:refnum<visa-resource-name>)  [unwired: 6 in]
        n514 = local read "mirr_Y#"() -> (w938:u8)
        n515 = call "zaber_readpos.vi"("error in (no error)"=w941, "axis"=w938, "VISA in"=w942) -> ("error out"=w939:errorcluster, "position"=→"mirr_posY":i32, "VISA out"=w940:refnum<visa-resource-name>)  [unwired: 6 in]
      }
    }
    "mirr_Error" <- w851
  }
  n516 = while {
    tunnel: w22 -> [w955]
    shift-right: [w953] -> _
    shift-left: _ -> [w951]
    shift-right: [w952] -> _
    shift-left: _ -> [w950]
    shift-right: [w948] -> _
    shift-left: 0 -> [w949]
    tunnel: w6 -> [w947]
    stop <- w954 stop-if-true
    # "ESP"
    n517 = Preview Queue Element(queue=w955, timeout in ms (-1)=w949) -> (queue out=w958:refnum<queue>, element=w959:string)  [unwired: 1 in, 2 out]
    n518 = Match Pattern(string=w959, regular expression=":") -> (before substring=w957:string, after substring=w956:string)  [unwired: 1 in, 2 out]
    n519 = case shown="\"idle\", Default" w957 {
      tunnel: w958 -> [_ w981 w1001 w1041 w1044 w1051 w1056]
      tunnel: w956 -> [_ w985 w1007 _ _ _ _]
      tunnel: [_ _ _ _ _ TRUE _] -> w954
      tunnel: [w964 w987 w1002 w1039 refnum<visa-resource-name> refnum ("VISA resource name out") w1048 w1055] -> w953
      tunnel: [w965 w988 w1000 w1038 w1046 w1049 w1054] -> w952
      tunnel: w951 -> [w974 w990 w1005 w1039 w1047 w1048 _]
      tunnel: w950 -> [w973 w989 w1006 w1038 _ w1049 _]
      tunnel: [_ _ _ -1 _ _ _] -> w948
      tunnel: w947 -> [_ _ w994 _ _ _ _]
      tunnel: "ESP patch" -> [w971 w980 w993 _ _ _ _]
      frame "idle", Default {
        n520 = Index Array(array=w971) -> (element #1=w970:i32, element #2=w967:i32)  [unwired: 3 in, 1 out]
        n521 = local read "ESP_t0"() -> (w977:dbl)
        n522 = call "Read Actual Position.vi"("error in (no error)"=w973, "Axis (1)"=w970, "VISA resource name"=w974) -> ("error out"=w968:errorcluster, "Position (units)"=w972:dbl, "VISA resource name out"=w969:refnum<visa-resource-name>)  [unwired: 2 in]
        "ESP_pos" <- w972
        n523 = call "mm2time.vi"("fs?"=TRUE, "Offset (mm)"=w977, "distance (mm)"=w972) -> ("time in fs/ps seconds"=→"ESP_delay":dbl)
        n524 = call "Read Actual Position.vi"("error in (no error)"=w968, "Axis (1)"=w967, "VISA resource name"=w969) -> ("error out"=w966:errorcluster, "Position (units)"=→"waveplate position":dbl, "VISA resource name out"=w963:refnum<visa-resource-name>)  [unwired: 2 in]
        n525 = call "Read Actual Position.vi"("error in (no error)"=w966, "VISA resource name"=w963) -> ("error out"=w965:errorcluster, "Position (units)"=→"stage2 position":dbl, "VISA resource name out"=w964:refnum<visa-resource-name>)  [unwired: 3 in]
      }
      frame "rel" {
        n526 = Dequeue Element(queue=w981) -> ()  [unwired: 2 in, 4 out]
        n527 = Match Pattern(string=w985, regular expression=":") -> (before substring=w984:string, after substring=w983:string)  [unwired: 1 in, 2 out]
        n528 = Decimal String To Number(string=w984) -> (number=w979:i32)  [unwired: 2 in, 1 out]
        n529 = Fract/Exp String To Number(string=w983) -> (number=w982:dbl)  [unwired: 3 in, 1 out]
        n530 = Index Array(array=w980, index=w979) -> (element=w978:i32)
        n531 = call "Move Relative.vi"("error in (no error)"=w989, "Position (0 units)"=w982, "Axis (1)"=w978, "VISA resource name"=w990) -> ("error out"=w988:errorcluster, "VISA resource name out"=w987:refnum<visa-resource-name>)  [unwired: 2 in]
      }
      frame "abs" {
        n532 = Dequeue Element(queue=w1001) -> ()  [unwired: 2 in, 4 out]
        n533 = Match Pattern(string=w1007, regular expression=":") -> (before substring=w1008:string, after substring=w998:string)  [unwired: 1 in, 2 out]
        n534 = Match Pattern(string=w998, regular expression=":") -> (before substring=w997:string, after substring=w996:string)  [unwired: 1 in, 2 out]
        n535 = Decimal String To Number(string=w1008) -> (number=w992:i32)  [unwired: 2 in, 1 out]
        n536 = Fract/Exp String To Number(string=w997) -> (number=w995:dbl)  [unwired: 3 in, 1 out]
        n537 = Index Array(array=w993, index=w992) -> (element=w991:i32)
        n538 = call "Move Absolute.vi"("error in (no error)"=w1006, "Position (0 units)"=w995, "Axis (1)"=w991, "VISA resource name"=w1005) -> ("error out"=w1003:errorcluster, "VISA resource name out"=w1004:refnum<visa-resource-name>)  [unwired: 2 in]
        n539 = case shown="\"wait\"" w996 {
          tunnel: w991 -> [_ w1012]
          tunnel: w1004 -> [w1011 w1028]
          tunnel: w1003 -> [w1010 w1027]
          tunnel: [w1011 w1017] -> w1002
          tunnel: [w1010 w1024] -> w1000
          tunnel: w994 -> [_ w1023]
          frame "", Default {
          }
          frame "wait" {
            n540 = while {
              tunnel: w1012 -> [w1037]
              shift-right: [w1034] -> w1026
              shift-left: w1028 -> [w1036]
              shift-right: [w1033] -> w1025
              shift-left: w1027 -> [w1035]
              stop <- w1032 stop-if-true
              n541 = call "Get Axis Motion Status.vi"("error in (no error)"=w1035, "Axis (1)"=w1037, "VISA resource name"=w1036) -> ("error out"=w1033:errorcluster, "Motion Done"=w1032:bool, "VISA resource name out"=w1034:refnum<visa-resource-name>)  [unwired: 2 in]
            }
            n542 = flat-sequence {
              tunnel: w1026 -> [w1031]
              tunnel: w1025 -> [w1030]
              tunnel: [w1031] -> w1019
              tunnel: [w1030] -> w1018
              frame #0 {
                n543 = Wait (ms)(milliseconds to wait=u32 1000) -> ()  [unwired: 1 out]
              }
            }
            n544 = local read "ESP_t0"() -> (w1021:dbl)
            n545 = call "Read Actual Position.vi"("error in (no error)"=w1018, "Axis (1)"=w1012, "VISA resource name"=w1019) -> ("error out"=w1013:errorcluster, "Position (units)"=w1015:dbl, "VISA resource name out"=w1017:refnum<visa-resource-name>)  [unwired: 2 in]
            n546 = call "mm2time.vi"("fs?"=TRUE, "Offset (mm)"=w1021, "distance (mm)"=w1015) -> ("time in fs/ps seconds"=w1016:dbl)
            n547 = call <vilib>:"Clear Errors.vi"("error in (no error)"=w1013) -> ("error out"=w1014:errorcluster)  [unwired: 5 in, 1 out]
            n548 = local write "ESP_pos"(w1015) -> ()
            n549 = local write "ESP_delay"(w1016) -> ()
            n550 = Send Notification(notification=TRUE, notifier=w1023, error in (no error)=w1014) -> (error out=w1024:errorcluster)  [unwired: 1 out]
          }
        }
      }
      frame "suspend" {
        n551 = Dequeue Element(queue=w1041) -> ()  [unwired: 2 in, 4 out]
      }
      frame "release" {
        n552 = Dequeue Element(queue=w1044) -> (queue out=w1042:refnum<queue>)  [unwired: 2 in, 3 out]
        n553 = call "Close.vi"("VISA resource name"=w1047) -> ("error out"=w1046:errorcluster)  [unwired: 10 in]
        n554 = Enqueue Element(queue=w1042, element="suspend") -> ()  [unwired: 2 in, 3 out]
      }
      frame "close" {
        n555 = Release Queue(queue=w1051) -> ()  [unwired: 2 in, 3 out]
      }
      frame "init" {
        n556 = Dequeue Element(queue=w1056) -> ()  [unwired: 2 in, 4 out]
        n557 = flat-sequence {
          tunnel: [w1059] -> w1053
          tunnel: [w1058] -> w1052
          tunnel: [w1063] -> w1054
          tunnel: [w1064] -> w1055
          tunnel: w1053 -> [w1064]
          tunnel: w1052 -> [w1063]
          frame #0 {
            n558 = local write "ESP_con?"(FALSE ("ESP_con?")) -> ()
          }
          frame #1 {
            n559 = call "Initialize.vi"("VISA resource name"="ESP301 VISA", "Serial Link (RS232)"=enum16{"RS232", "USB"}."RS232") -> ("VISA resource name out"=w1059:refnum<visa-resource-name>, "error out"=w1058:errorcluster)  [unwired: 7 in]
          }
          frame #2 {
            n560 = local write "ESP_con?"(TRUE ("ESP_con?")) -> ()
          }
        }
      }
    }
    "error out" <- w952
  }
  n561 = while {
    tunnel: w21 -> [w1073]
    shift-right: [w1071] -> _
    shift-left: _ -> [w1069]
    shift-right: [w1070] -> _
    shift-left: _ -> [w1068]
    shift-right: [w1066] -> _
    shift-left: 0 -> [w1067]
    tunnel: w6 -> [w1065]
    stop <- w1072 stop-if-true
    # "manip"
    n562 = Preview Queue Element(queue=w1073, timeout in ms (-1)=w1067) -> (queue out=w1076:refnum<queue>, element=w1077:string)  [unwired: 1 in, 2 out]
    n563 = Match Pattern(string=w1077, regular expression=":") -> (before substring=w1075:string, after substring=w1074:string)  [unwired: 1 in, 2 out]
    n564 = case shown="\"init\"" w1075 {
      tunnel: w1076 -> [_ w1089 w1116 w1163 w1201 w1207 w1216 w1221]
      tunnel: w1074 -> [_ _ w1103 w1162 _ _ _ _]
      tunnel: [_ _ _ _ _ _ TRUE _] -> w1072
      tunnel: [w1083 w1091 w1095 w1160 w1203 refnum<k5> refnum ("gateway_connection out") w1214 w1220] -> w1071
      tunnel: [w1082 w1090 w1097 w1159 w1202 w1209 w1213 w1219] -> w1070
      tunnel: w1069 -> [w1085 w1093 w1119 w1153 w1203 w1211 w1214 _]
      tunnel: w1068 -> [w1084 w1092 w1118 w1154 w1202 _ w1213 _]
      tunnel: [_ _ _ _ -1 _ _ _] -> w1066
      tunnel: w1065 -> [_ _ w1094 w1156 _ _ _ _]
      frame "idle", Default {
        n565 = call "sp_manip_get_axis_status.vi"("error in"=w1084, "gateway_connection"=w1085) -> ("error out"=w1082:errorcluster, "axis_out"=w1081:T9, "gateway_connection out"=w1083:refnum<k5>)  [unwired: 5 in, 2 out]
        n566 = for {
          tunnel: w1081 -> [w1088] mode=indexing
          tunnel: [w1087] -> w1080 mode=indexing
          tunnel: [w1086] -> w1079 mode=indexing
          n567 = Unbundle By Name(w1088) -> ("Axis_Position"=w1087:dbl, "moving"=w1086:bool)
        }
        "moving?" <- w1079
        n568 = local write "pos"(w1080) -> ()
      }
      frame "stop" {
        n569 = Dequeue Element(queue=w1089) -> ()  [unwired: 2 in, 4 out]
        n570 = call "sp_manip_abort.vi"("error in"=w1092, "gateway_connection"=w1093) -> ("error out"=w1090:errorcluster, "gateway_connection out"=w1091:refnum<k5>)  [unwired: 6 in, 2 out]
      }
      frame "rel" {
        n571 = Dequeue Element(queue=w1116) -> ()  [unwired: 2 in, 4 out]
        n572 = Match Pattern(string=w1103, regular expression=":") -> (before substring=w1102:string, after substring=w1101:string)  [unwired: 1 in, 2 out]
        n573 = Equal?(x=w1101, y="wait") -> (x = y?=w1099:bool)
        n574 = call "sp_manip_get_axis_status.vi"("error in"=w1118, "gateway_connection"=w1119) -> ("error out"=w1121:errorcluster, "axis_out"=w1108:T9, "gateway_connection out"=w1120:refnum<k5>)  [unwired: 5 in, 2 out]
        n575 = Scan From String(format string="%g_%g_%g_%g_%g_%g", input string=w1102) -> (output 1=w1115:dbl, output 2=w1114:dbl, output 3=w1113:dbl, output 4=w1112:dbl, output 5=w1111:dbl, output 6=w1110:dbl)  [unwired: 8 in, 3 out]
        n576 = for {
          tunnel: w1108 -> [w1148] mode=indexing
          tunnel: [w1147] -> w1106 mode=indexing
          tunnel: [w1146] -> w1107 mode=indexing
          n577 = Unbundle By Name(w1148) -> ("Axis_Name"=w1147:string, "Axis_Position"=w1146:dbl)
        }
        n578 = Build Array(w1115, w1114, w1113, w1112, w1111, w1110) -> (w1109:dbl[])
        n579 = Add(x=w1107, y=w1109) -> (x+y=w1105:dbl[])
        n580 = call "sp_manip_start_move.vi"("error in"=w1121, "target positions"=w1105, "axis names"=w1106, "gateway_connection"=w1120) -> ("error out"=w1098:errorcluster, "gateway_connection out"=w1096:refnum<k5>)  [unwired: 4 in, 2 out]
        n581 = case shown="True" w1099 {
          tunnel: w1098 -> [w1122 w1133]
          tunnel: [w1122 w1132] -> w1097
          tunnel: w1096 -> [w1123 w1134]
          tunnel: [w1123 w1126] -> w1095
          tunnel: w1094 -> [_ w1131]
          frame False {
          }
          frame True {
            n582 = while {
              tunnel: w1134 -> [w1140]
              tunnel: w1133 -> [w1139]
              tunnel: [w1138] -> w1127
              tunnel: [w1137] -> w1125
              stop <- w1141 continue-if-true
              n583 = call "sp_manip_get_axis_status.vi"("error in"=w1139, "gateway_connection"=w1140) -> ("error out"=w1137:errorcluster, "axis_out"=w1143:T9, "gateway_connection out"=w1138:refnum<k5>)  [unwired: 5 in, 2 out]
              n584 = for {
                tunnel: w1143 -> [w1145] mode=indexing
                tunnel: [w1144] -> w1142 mode=indexing
                n585 = Unbundle By Name(w1145) -> ("moving"=w1144:bool)
              }
              n586 = Or Array Elements(Boolean array=w1142) -> (logical OR=w1141:bool)
            }
            n587 = call "sp_manip_get_axis_status.vi"("error in"=w1125, "gateway_connection"=w1127) -> ("error out"=w1124:errorcluster, "axis_out"=w1129:T9, "gateway_connection out"=w1126:refnum<k5>)  [unwired: 5 in, 2 out]
            n588 = for {
              tunnel: w1129 -> [w1136] mode=indexing
              tunnel: [w1135] -> w1128 mode=indexing
              n589 = Unbundle By Name(w1136) -> ("Axis_Position"=w1135:dbl)
            }
            n590 = Send Notification(notification=TRUE, notifier=w1131, error in (no error)=w1124) -> (error out=w1132:errorcluster)  [unwired: 1 out]
            n591 = local write "dest"(w1128) -> ()
          }
        }
      }
      frame "abs" {
        n592 = Dequeue Element(queue=w1163) -> ()  [unwired: 2 in, 4 out]
        n593 = call "sp_manip_get_axis_status.vi"("error in"=w1154, "gateway_connection"=w1153) -> ("error out"=w1149:errorcluster, "axis_out"=w1152:T9, "gateway_connection out"=w1150:refnum<k5>)  [unwired: 5 in, 2 out]
        n594 = Match Pattern(string=w1162, regular expression=":") -> (before substring=w1166:string, after substring=w1165:string)  [unwired: 1 in, 2 out]
        n595 = Equal?(x=w1165, y="wait") -> (x = y?=w1155:bool)
        n596 = for {
          tunnel: w1152 -> [w1176] mode=indexing
          tunnel: [w1175] -> w1151 mode=indexing
          n597 = Unbundle By Name(w1176) -> ("Axis_Name"=w1175:string)
        }
        n598 = Scan From String(format string="%g_%g_%g_%g_%g_%g", input string=w1166) -> (output 1=w1172:dbl, output 2=w1171:dbl, output 3=w1170:dbl, output 4=w1169:dbl, output 5=w1168:dbl, output 6=w1167:dbl)  [unwired: 8 in, 3 out]
        n599 = Build Array(w1172, w1171, w1170, w1169, w1168, w1167) -> (w1174:dbl[])
        n600 = call "sp_manip_start_move.vi"("error in"=w1149, "target positions"=w1174, "axis names"=w1151, "gateway_connection"=w1150) -> ("error out"=w1158:errorcluster, "gateway_connection out"=w1157:refnum<k5>)  [unwired: 4 in, 2 out]
        n601 = case shown="True" w1155 {
          tunnel: w1158 -> [w1177 w1188]
          tunnel: [w1177 w1187] -> w1159
          tunnel: w1157 -> [w1178 w1189]
          tunnel: [w1178 w1180] -> w1160
          tunnel: w1156 -> [_ w1186]
          frame False {
          }
          frame True {
            n602 = while {
              tunnel: w1189 -> [w1195]
              tunnel: w1188 -> [w1194]
              tunnel: [w1193] -> w1182
              tunnel: [w1192] -> w1181
              stop <- w1196 continue-if-true
              n603 = call "sp_manip_get_axis_status.vi"("error in"=w1194, "gateway_connection"=w1195) -> ("error out"=w1192:errorcluster, "axis_out"=w1198:T9, "gateway_connection out"=w1193:refnum<k5>)  [unwired: 5 in, 2 out]
              n604 = for {
                tunnel: w1198 -> [w1200] mode=indexing
                tunnel: [w1199] -> w1197 mode=indexing
                n605 = Unbundle By Name(w1200) -> ("moving"=w1199:bool)
              }
              n606 = Or Array Elements(Boolean array=w1197) -> (logical OR=w1196:bool)
            }
            n607 = call "sp_manip_get_axis_status.vi"("error in"=w1181, "gateway_connection"=w1182) -> ("error out"=w1179:errorcluster, "axis_out"=w1184:T9, "gateway_connection out"=w1180:refnum<k5>)  [unwired: 5 in, 2 out]
            n608 = for {
              tunnel: w1184 -> [w1191] mode=indexing
              tunnel: [w1190] -> w1183 mode=indexing
              n609 = Unbundle By Name(w1191) -> ("Axis_Position"=w1190:dbl)
            }
            n610 = local write "pos"(w1183) -> ()
            n611 = Send Notification(notification=TRUE, notifier=w1186, error in (no error)=w1179) -> (error out=w1187:errorcluster)  [unwired: 1 out]
          }
        }
      }
      frame "suspend" {
        n612 = Dequeue Element(queue=w1201) -> ()  [unwired: 2 in, 4 out]
      }
      frame "release" {
        n613 = Dequeue Element(queue=w1207) -> (queue out=w1205:refnum<queue>)  [unwired: 2 in, 3 out]
        n614 = call "sp_manip_disconnect.vi"("gateway_connection"=w1211) -> ("error out"=w1210:errorcluster, "gateway_connection_out"=w1212:refnum<k5>)  [unwired: 7 in, 2 out]
        n615 = call "tcp_gateway_close_connection.vi"("error in"=w1210, "server_connection"=w1212) -> ("error out"=w1209:errorcluster)  [unwired: 5 in]
        n616 = Enqueue Element(queue=w1205, element="suspend") -> ()  [unwired: 2 in, 3 out]
      }
      frame "close" {
        n617 = Release Queue(queue=w1216) -> ()  [unwired: 2 in, 3 out]
      }
      frame "init" {
        n618 = Dequeue Element(queue=w1221) -> ()  [unwired: 2 in, 4 out]
        n619 = flat-sequence {
          tunnel: [w1224] -> w1218
          tunnel: [w1223] -> w1217
          tunnel: [w1234] -> w1219
          tunnel: [w1235] -> w1220
          tunnel: w1218 -> [w1235]
          tunnel: w1217 -> [w1234]
          frame #0 {
            n620 = local write "manip_con?"(FALSE ("manip_con?")) -> ()
          }
          frame #1 {
            n621 = call "tcp_gateway_open_connection.vi"() -> ("gateway_connection"=w1227:refnum<k5>, "error out"=w1226:errorcluster)  [unwired: 5 in, 3 out]
            n622 = call "sp_manip_connect.vi"("error in"=w1226, "gateway_connection"=w1227) -> ("error out"=w1223:errorcluster, "axis_out"=w1225:T9, "gateway_connection out"=w1224:refnum<k5>)  [unwired: 5 in, 2 out]
            n623 = for {
              tunnel: w1225 -> [w1232] mode=indexing
              tunnel: [w1231] -> w1228 mode=indexing
              tunnel: [w1230] -> w1229 mode=indexing
              n624 = Unbundle By Name(w1232) -> ("Axis_Name"=w1231:string, "Axis_Position"=w1230:dbl)
            }
            "axis" <- w1228
            "pos" <- w1229
            n625 = local write "dest"(w1229) -> ()
          }
          frame #2 {
            n626 = local write "manip_con?"(TRUE ("manip_con?")) -> ()
          }
        }
      }
    }
    "error out 2" <- w1070
  }
  n627 = while {
    tunnel: w20 -> [w1247]
    shift-right: [w1236] -> _
    shift-left: 0 -> [w1245]
    shift-right: [w1244] -> _
    shift-left: _ -> [w1243]
    shift-right: [w1242] -> _
    shift-left: _ -> [w1241]
    shift-right: [w1240] -> _
    shift-left: u32 0 ("pHandle") -> [w1239]
    tunnel: w18 -> [w1238]
    tunnel: w6 -> [w1237]
    stop <- w1246 stop-if-true
    # "phoib"
    n628 = Preview Queue Element(queue=w1247, timeout in ms (-1)=w1245) -> (queue out=w1250:refnum<queue>, element=w1251:string)  [unwired: 1 in, 2 out]
    n629 = Match Pattern(string=w1251, regular expression=":") -> (before substring=w1249:string, after substring=w1248:string)  [unwired: 1 in, 2 out]
    n630 = case shown="\"idle\", Default" w1249 {
      tunnel: w1250 -> [_ w1308 w1363 w1380 w1398 w1412 w1417 w1422]
      tunnel: w1248 -> [_ _ w1359 _ _ _ _ _]
      tunnel: [_ _ _ _ _ TRUE _ _] -> w1246
      tunnel: [w1262 w1310 w1328 w1383 w1396 w1410 w1416 w1419] -> w1244
      tunnel: w1243 -> [w1273 w1299 w1349 w1385 w1397 w1410 w1416 _]
      tunnel: [w1261 w1309 w1344 w1382 w1395 w1408 w1414 w1418] -> w1242
      tunnel: w1241 -> [w1271 w1298 _ w1384 _ w1408 w1414 _]
      tunnel: [w1259 w1296 w1327 w1381 w1394 w1409 w1415 w1421] -> w1240
      tunnel: w1239 -> [w1259 w1296 w1347 w1381 w1393 w1409 w1415 _]
      tunnel: w1238 -> [w1260 w1289 w1325 _ _ _ _ _]
      tunnel: w1237 -> [_ _ w1343 _ _ _ _ _]
      tunnel: [_ _ _ _ _ _ -1 _] -> w1236
      frame "idle", Default {
        n631 = call "SL2_AD_DLL_Phoibos_GetDeviceState.vi"("dll_path"=w1273, "pHandle_in"=w1259, "dev_type"=DEF_dev_type."devA (analyzer)", "error in"=w1271) -> ("path out"=w1258:path, "state"=→"state":T3, "error out"=w1257:errorcluster)  [unwired: 2 in]
        n632 = for {
          tunnel: w1259 -> [w1280]
          tunnel: w1260 -> [w1278] mode=indexing
          tunnel: [w1277] -> w1270 mode=indexing
          tunnel: [w1276] -> w1262
          shift-right: [w1275] -> w1261
          shift-left: w1257 -> [w1279]
          tunnel: w1258 -> [w1274]
          n633 = call "SL2_AD_DLL_Phoibos_GetVoltage.vi"("error in"=w1279, "voltage_name"=w1278, "pHandle"=w1280, "dll path in"=w1274) -> ("error out"=w1275:errorcluster, "value"=w1277:dbl, "dll path out"=w1276:path)  [unwired: 3 in]
        }
        n634 = Index Array(array=w1270) -> (element #1=→"phoib_I_1":dbl, element #2=→"phoib_I_2":dbl, element #3=→"phoib_I_3":dbl, element #4=→"phoib_I_4":dbl, element #5=→"phoib_I_5":dbl, element #6=→"phoib_I_6":dbl, element #7=→"phoib_I_7":dbl, element #8=→"phoib_I_8":dbl, element #9=→"phoib_I_9":dbl, element #10=→"phoib_I_10":dbl)  [unwired: 10 in]
      }
      frame "set" {
        n635 = Dequeue Element(queue=w1308) -> ()  [unwired: 2 in, 4 out]
        n636 = Add(x=u32[] [251749632, 251749633, 251749634, 251749635, 251749636, 251749637, 251749638, 251749639, 251749640, 251749641, 251749642, 251749643, 251749644, 251749645, 251749646, 251749647, 251749648, 251749649, 251749650, 251749651, 251749652, 251749653, 251749654, 251749655, 251749656, 251749657, 251749658, 251749659, 251749660, 251749661, 251749662, 251749663, 251749664, 251749665, 251749666, 251749667, 251749668, 251749669, 251749670, 251749671, 251749672, 251749673, 251749674, 251749675, 251749676, 251749677, 251749678, 251749679, 251749680, 251749681, 251749682, 251749683, 251749684, 251749685, 251749686, 251749687, 251749688, 251749689, 251749690, 251749691, 251749692, 251749693, 251749694, 251749695, 251749696] ("modeIDs"), y=9984) -> (x+y=w1282:u32[])
        n637 = Multiply(x="ana_voltrange", y=12) -> (x*y=w1305:i32)
        n638 = Add(x="ana_mode", y=w1305) -> (x+y=w1302:i32)
        n639 = Index Array(array=w1282, index=w1302) -> (element=w1300:u32)
        n640 = Build Array("phoib_I_1s", "phoib_I_2s", "phoib_I_3s", "phoib_I_4s", "phoib_I_5s", "phoib_I_6s", "phoib_I_7s", "phoib_I_8s", "phoib_I_9s", "phoib_I_10s") -> (w1288:dbl[])
        n641 = call "SL2_AD_DLL_Phoibos_SetDeviceMode.vi"("pHandle"=w1296, "error in"=w1298, "value"=w1300, "dev_type"=DEF_dev_type."devA (analyzer)", "dll path in"=w1299) -> ("error out"=w1287:errorcluster, "dll path out"=w1297:path)  [unwired: 4 in]
        n642 = for {
          tunnel: w1296 -> [w1316]
          shift-right: [w1323] -> w1310
          shift-left: w1297 -> [w1320]
          tunnel: w1289 -> [w1315] mode=indexing
          tunnel: w1288 -> [w1314] mode=indexing
          shift-right: [w1322] -> w1309
          shift-left: w1287 -> [w1318]
          n643 = call "SL2_AD_DLL_Phoibos_GetVoltageRange.vi"("error in"=w1318, "voltage_name"=w1315, "pHandle"=w1316, "dll path in"=w1320) -> ("error out"=w1317:errorcluster, "min"=w1312:dbl, "max"=w1313:dbl, "dll path out"=w1319:path)  [unwired: 2 in]
          n644 = In Range and Coerce(upper limit=w1313, x=w1314, lower limit=w1312) -> (coerced(x)=w1311:dbl)  [unwired: 1 out]
          n645 = call "SL2_AD_DLL_Phoibos_SetVoltage.vi"("commit"=TRUE, "pHandle"=w1316, "error in"=w1317, "value"=w1311, "voltageName"=w1315, "dll path in"=w1319) -> ("error out"=w1322:errorcluster, "dll path out"=w1323:path)  [unwired: 3 in]
        }
      }
      frame "setsgl" {
        n646 = Dequeue Element(queue=w1363) -> ()  [unwired: 2 in, 4 out]
        n647 = Match Pattern(string=w1359, regular expression=":") -> (before substring=w1352:string, after substring=w1361:string)  [unwired: 1 in, 2 out]
        n648 = Equal?(x=w1361, y="wait") -> ()  [unwired: 1 out]
        n649 = Match Pattern(string=w1352, regular expression=":") -> (before substring=w1326:string, after substring=w1351:string)  [unwired: 1 in, 2 out]
        n650 = Fract/Exp String To Number(string=w1351) -> (number=w1350:dbl)  [unwired: 3 in, 1 out]
        n651 = call "SL2_AD_DLL_Phoibos_GetVoltageRange.vi"("voltage_name"=w1326, "pHandle"=w1347, "dll path in"=w1349) -> ("error out"=w1356:errorcluster, "min"=w1354:dbl, "max"=w1355:dbl, "dll path out"=w1357:path)  [unwired: 3 in]
        n652 = In Range and Coerce(upper limit=w1355, x=w1350, lower limit=w1354) -> (coerced(x)=w1345:dbl)  [unwired: 1 out]
        n653 = call "SL2_AD_DLL_Phoibos_SetVoltage.vi"("commit"=TRUE, "pHandle"=w1347, "error in"=w1356, "value"=w1345, "voltageName"=w1326, "dll path in"=w1357) -> ("error out"=w1346:errorcluster, "dll path out"=w1348:path)  [unwired: 3 in]
        n654 = while {
          tunnel: w1348 -> [w1379]
          tunnel: w1347 -> [w1373]
          tunnel: w1326 -> [w1378]
          tunnel: w1346 -> [w1377]
          tunnel: w1345 -> [w1376]
          tunnel: [w1373] -> w1327
          tunnel: [w1372] -> w1329
          tunnel: [w1371] -> w1331
          stop <- w1374 stop-if-true
          n655 = call "SL2_AD_DLL_Phoibos_GetVoltage.vi"("error in"=w1377, "voltage_name"=w1378, "pHandle"=w1373, "dll path in"=w1379) -> ("error out"=w1371:errorcluster, "value"=w1375:dbl, "dll path out"=w1372:path)  [unwired: 3 in]
          n656 = Equal?(x=w1376, y=w1375) -> (x = y?=w1374:bool)
        }
        n657 = for {
          tunnel: w1327 -> [w1370]
          tunnel: [w1368] -> w1332 mode=indexing
          tunnel: [w1367] -> w1328
          shift-right: [w1366] -> w1330
          shift-left: w1331 -> [w1369]
          tunnel: w1329 -> [w1365]
          tunnel: w1325 -> [w1364] mode=indexing
          n658 = call "SL2_AD_DLL_Phoibos_GetVoltage.vi"("error in"=w1369, "voltage_name"=w1364, "pHandle"=w1370, "dll path in"=w1365) -> ("error out"=w1366:errorcluster, "value"=w1368:dbl, "dll path out"=w1367:path)  [unwired: 3 in]
        }
        n659 = Index Array(array=w1332) -> (element #1=w1333:dbl, element #2=w1334:dbl, element #3=w1335:dbl, element #4=w1336:dbl, element #5=w1337:dbl, element #6=w1341:dbl, element #7=w1338:dbl, element #8=w1339:dbl, element #9=w1340:dbl, element #10=w1324:dbl)  [unwired: 10 in]
        n660 = local write "phoib_I_1"(w1333) -> ()
        n661 = local write "phoib_I_2"(w1334) -> ()
        n662 = local write "phoib_I_3"(w1335) -> ()
        n663 = local write "phoib_I_4"(w1336) -> ()
        n664 = local write "phoib_I_5"(w1337) -> ()
        n665 = local write "phoib_I_6"(w1341) -> ()
        n666 = local write "phoib_I_7"(w1338) -> ()
        n667 = local write "phoib_I_8"(w1339) -> ()
        n668 = local write "phoib_I_9"(w1340) -> ()
        n669 = local write "phoib_I_10"(w1324) -> ()
        n670 = Send Notification(notification=TRUE, notifier=w1343, error in (no error)=w1330) -> (error out=w1344:errorcluster)  [unwired: 1 out]
      }
      frame "standby" {
        w1386 = T3 0 items=["Off"=-1, "Standby"=0, "On"=1] ("state")
        n671 = Dequeue Element(queue=w1380) -> ()  [unwired: 2 in, 4 out]
        n672 = call "SL2_AD_DLL_Phoibos_SetDeviceState.vi"("pHandle_in"=w1381, "error in"=w1384, "state"=w1386, "dev_type"=DEF_dev_type."devA (analyzer)", "dll_path"=w1385) -> ("error out"=w1382:errorcluster, "path out"=w1383:path)  [unwired: 2 in]
      }
      frame "release" {
        n673 = Dequeue Element(queue=w1398) -> (queue out=w1388:refnum<queue>)  [unwired: 2 in, 3 out]
        n674 = flat-sequence {
          tunnel: w1397 -> [w1399]
          tunnel: w1393 -> [w1400]
          tunnel: [w1403] -> w1392
          tunnel: [w1402] -> w1391
          tunnel: [u32 0] -> w1390
          tunnel: [w1405] -> w1394
          tunnel: [w1406] -> w1395
          tunnel: [w1407] -> w1396
          tunnel: w1392 -> [w1407]
          tunnel: w1391 -> [w1406]
          tunnel: w1390 -> [w1405]
          frame #0 {
            n675 = call "SL2_AD_DLL_Phoibos_Shutdown.vi"("pHandle"=w1400, "dll path in"=w1399) -> ("error out"=w1402:errorcluster, "dll path out"=w1403:path)  [unwired: 4 in]
          }
          frame #1 {
            n676 = local write "phoib_con?"(FALSE ("phoib_con?")) -> ()
          }
        }
        n677 = Enqueue Element(queue=w1388, element="suspend") -> ()  [unwired: 2 in, 3 out]
      }
      frame "close" {
        n678 = Release Queue(queue=w1412) -> ()  [unwired: 2 in, 3 out]
      }
      frame "suspend" {
        n679 = Dequeue Element(queue=w1417) -> ()  [unwired: 2 in, 4 out]
      }
      frame "init" {
        n680 = Dequeue Element(queue=w1422) -> ()  [unwired: 2 in, 4 out]
        n681 = flat-sequence {
          tunnel: [w1429] -> w1420
          tunnel: [w1425] -> w1419
          tunnel: [w1424] -> w1418
          tunnel: [w1437] -> w1421
          tunnel: w1420 -> [w1437]
          frame #0 {
            n682 = local write "phoib_con?"(FALSE ("phoib_con?")) -> ()
          }
          frame #1 {
            w1428 = DEF_dev_type."devA (analyzer)" ("dev_type")
            n683 = call "GetSL2AD_VI_dllPath.vi"() -> ("error"=w1432:errorcluster, "Path"=w1433:path)  [unwired: 9 in, 1 out]
            n684 = call "SL2_AD_DLL_List_Devices.vi"("error in"=w1432, "dev_type"=w1428, "dll path in"=w1433) -> ("error out"=w1426:errorcluster, "devices"=w1435:string[], "dll path out"=w1427:path)  [unwired: 2 in]
            n685 = Index Array(array=w1435) -> (element=w1434:string)  [unwired: 1 in]
            n686 = call "SL2_AD_DLL_Phoibos_Initialize.vi"("error in"=w1426, "analyzerId"=w1434, "dll_path"=w1427) -> ("error out"=w1430:errorcluster, "pHandle"=w1429:u32, "path out"=w1431:path)  [unwired: 2 in]
            n687 = call "SL2_AD_DLL_Phoibos_ListDeviceModes.vi"("dll path in"=w1431, "dev_type"=w1428, "pHandle"=w1429, "error in"=w1430) -> ("dll path out"=w1425:path, "error out"=w1424:errorcluster)  [unwired: 1 in, 2 out]
          }
          frame #2 {
            n688 = local write "phoib_con?"(TRUE ("phoib_con?")) -> ()
          }
        }
      }
    }
    "phoib_error" <- w1242
  }
  n689 = while {
    tunnel: w7 -> [w1447]
    tunnel: w6 -> [w1441]
    shift-right: [w1440] -> _
    shift-left: 0 -> [w1439]
    stop <- w1438 stop-if-true
    # "temp"
    n690 = Preview Queue Element(queue=w1447, timeout in ms (-1)=w1439) -> (queue out=w1442:refnum<queue>, element=w1446:string)  [unwired: 1 in, 2 out]
    n691 = Match Pattern(string=w1446, regular expression=":") -> (before substring=w1445:string, after substring=w1444:string)  [unwired: 1 in, 2 out]
    n692 = case shown="\"ramp\"" w1445 {
      tunnel: w1444 -> [w1453 _ _ _ _]
      tunnel: w1442 -> [w1448 w1473 w1474 _ w1487]
      tunnel: w1441 -> [w1449 _ _ _ _]
      tunnel: [_ _ _ _ -1] -> w1440
      tunnel: [_ TRUE _ _ _] -> w1438
      frame "ramp" {
        n693 = Dequeue Element(queue=w1448) -> ()  [unwired: 2 in, 4 out]
        n694 = Match Pattern(string=w1453, regular expression=":") -> (before substring=w1452:string, after substring=w1456:string)  [unwired: 1 in, 2 out]
        n695 = Equal?(x=w1456, y="wait") -> (x = y?=w1450:bool)
        n696 = Scan From String(input string=w1452) -> (output 1=w1451:dbl)  [unwired: 4 in, 3 out]
        n697 = flat-sequence {
          tunnel: w1451 -> [w1458]
          tunnel: w1450 -> [w1460]
          tunnel: w1449 -> [w1470]
          frame #0 {
            n698 = local read "LS310  EPICS SP"() -> (w1457:string)
            n699 = call-poly <userlib>:"CaLabPut.vi"("Value"=w1458, "PV Name"=w1457) -> ()  [unwired: 6 in, 4 out]
          }
          frame #1 {
            n700 = Wait (ms)(milliseconds to wait=500) -> ()  [unwired: 1 out]
          }
          frame #2 {
            n701 = case shown="True" w1460 {
              frame False {
              }
              frame True {
                n702 = while {
                  stop <- w1466 stop-if-true
                  n703 = local read "Status EPICS chanel"() -> (w1468:string)
                  n704 = Wait (ms)(milliseconds to wait=500) -> ()  [unwired: 1 out]
                  n705 = call-poly <userlib>:"CaLabGet.vi"("PV Name"=w1468) -> ("1rst Value (string)"=w1469:string)  [unwired: 8 in, 6 out]
                  n706 = Equal?(x=w1469, y="Inside Range") -> (x = y?=w1466:bool)
                  n707 = local read "LS310  EPICS chanel A"() -> (w1462:string)
                  n708 = local read "LS310  EPICS chanel B"() -> (w1461:string)
                  n709 = call-poly <userlib>:"CaLabGet.vi"("PV Name"=w1462) -> ("1rst Value (number)"=w1463:dbl)  [unwired: 8 in, 6 out]
                  n710 = call-poly <userlib>:"CaLabGet.vi"("PV Name"=w1461) -> ("1rst Value (number)"=w1464:dbl)  [unwired: 8 in, 6 out]
                  n711 = local write "TB"(w1464) -> ()
                  n712 = local write "TA"(w1463) -> ()
                }
              }
            }
          }
          frame #3 {
            n713 = Send Notification(notification=TRUE, notifier=w1470) -> ()  [unwired: 1 in, 2 out]
          }
        }
      }
      frame "close" {
        n714 = Release Queue(queue=w1473) -> ()  [unwired: 2 in, 3 out]
      }
      frame "init" {
        n715 = Dequeue Element(queue=w1474) -> ()  [unwired: 2 in, 4 out]
      }
      frame "idle", Default {
        n716 = local read "LS310  EPICS chanel A"() -> (w1485:string)
        n717 = local read "LS310  EPICS chanel B"() -> (w1484:string)
        n718 = local read "LS310  EPICS SP"() -> (w1475:string)
        n719 = local read "Status EPICS chanel"() -> (w1483:string)
        n720 = local read "LS310  EPICS Heater"() -> (w1482:string)
        n721 = call-poly <userlib>:"CaLabGet.vi"("PV Name"=w1485) -> ("1rst Value (number)"=→"TA":dbl)  [unwired: 8 in, 6 out]
        n722 = call-poly <userlib>:"CaLabGet.vi"("PV Name"=w1484) -> ("1rst Value (number)"=→"TB":dbl)  [unwired: 8 in, 6 out]
        n723 = call-poly <userlib>:"CaLabGet.vi"("PV Name"=w1475) -> ("1rst Value (number)"=→"Readback":dbl)  [unwired: 8 in, 6 out]
        n724 = call-poly <userlib>:"CaLabGet.vi"("PV Name"=w1483) -> ("1rst Value (string)"=w1479:string)  [unwired: 8 in, 6 out]
        n725 = call-poly <userlib>:"CaLabGet.vi"("PV Name"=w1482) -> ()  [unwired: 8 in, 7 out]
        n726 = Equal?(x=w1479, y="Inside Range") -> (x = y?=→"In Range":bool)
      }
      frame "suspend" {
        n727 = Dequeue Element(queue=w1487) -> ()  [unwired: 2 in, 4 out]
      }
    }
  }
  n728 = while {
    tunnel: w4 -> [w1497]
    tunnel: w6 -> [w1491]
    shift-right: [w1490] -> _
    shift-left: _ -> [w1489]
    stop <- w1488 stop-if-true
    # "temp"
    n729 = Preview Queue Element(queue=w1497, timeout in ms (-1)=w1489) -> (queue out=w1492:refnum<queue>, element=w1496:string)  [unwired: 1 in, 2 out]
    n730 = Match Pattern(string=w1496, regular expression=":") -> (before substring=w1495:string, after substring=w1494:string)  [unwired: 1 in, 2 out]
    n731 = case shown="\"abs\"" w1495 {
      tunnel: w1494 -> [w1504 _ _ _ _]
      tunnel: w1492 -> [w1499 w1524 w1525 _ w1529]
      tunnel: w1491 -> [w1500 _ _ _ _]
      tunnel: [_ _ _ _ -1] -> w1490
      tunnel: [_ TRUE _ _ _] -> w1488
      frame "abs" {
        n732 = Dequeue Element(queue=w1499) -> ()  [unwired: 2 in, 4 out]
        n733 = Match Pattern(string=w1504, regular expression=":") -> (before substring=w1503:string, after substring=w1507:string)  [unwired: 1 in, 2 out]
        n734 = Equal?(x=w1507, y="wait") -> (x = y?=w1501:bool)
        n735 = Scan From String(input string=w1503) -> (output 1=w1502:dbl)  [unwired: 4 in, 3 out]
        n736 = flat-sequence {
          tunnel: w1502 -> [w1508]
          tunnel: [w1508] -> w1498
          tunnel: w1501 -> [w1511]
          tunnel: w1498 -> [w1510]
          tunnel: w1500 -> [w1521]
          frame #0 {
            n737 = local read "WattPilot EPICS chanel set"() -> (w1509:string)
            n738 = call-poly <userlib>:"CaLabPut.vi"("Value"=w1508, "PV Name"=w1509) -> ()  [unwired: 6 in, 4 out]
          }
          frame #1 {
            n739 = case shown="True" w1511 {
              tunnel: w1510 -> [_ w1512]
              frame False {
              }
              frame True {
                n740 = while {
                  tunnel: w1512 -> [w1517]
                  stop <- w1514 stop-if-true
                  n741 = local read "WattPilot EPICS chanel readback"() -> (w1519:string)
                  n742 = Wait (ms)(milliseconds to wait=500) -> ()  [unwired: 1 out]
                  n743 = call-poly <userlib>:"CaLabGet.vi"("PV Name"=w1519) -> ("1rst Value (number)"=w1518:dbl)  [unwired: 8 in, 6 out]
                  n744 = Subtract(x=w1518, y=w1517) -> (x-y=w1516:dbl)
                  n745 = Absolute Value(x=w1516) -> (abs(x)=w1515:dbl)
                  n746 = local write "Readback_wattpilot"(w1518) -> ()
                  n747 = Less?(x=w1515, y=0.1) -> (x < y?=w1514:bool)
                }
              }
            }
          }
          frame #2 {
            n748 = Send Notification(notification=TRUE, notifier=w1521) -> ()  [unwired: 1 in, 2 out]
          }
        }
      }
      frame "close" {
        n749 = Release Queue(queue=w1524) -> ()  [unwired: 2 in, 3 out]
      }
      frame "init" {
        n750 = Dequeue Element(queue=w1525) -> ()  [unwired: 2 in, 4 out]
      }
      frame "idle", Default {
        n751 = local read "WattPilot EPICS chanel readback"() -> (w1527:string)
        n752 = call-poly <userlib>:"CaLabGet.vi"("PV Name"=w1527) -> ("1rst Value (number)"=→"Readback_wattpilot":dbl)  [unwired: 8 in, 6 out]
      }
      frame "suspend" {
        n753 = Dequeue Element(queue=w1529) -> ()  [unwired: 2 in, 4 out]
      }
    }
  }
  n754 = while {
    tunnel: w23 -> [w1556]
    shift-right: [w1550] -> _
    shift-left: _ -> [w1549]
    shift-right: [w1548] -> _
    shift-left: _ -> [w1546]
    shift-right: [w1547] -> _
    shift-left: _ -> [w1545]
    shift-right: [w1542] -> _
    shift-left: 0 -> [w1543]
    shift-right: [w1541] -> _
    shift-left: _ -> [w1540]
    shift-right: [w1539] -> _
    shift-left: _ -> [w1538]
    tunnel: w32 -> [w1537]
    shift-right: [w1536] -> _
    shift-left: _ -> [w1535]
    shift-right: [w1533] -> _
    shift-left: _ -> [w1532]
    shift-right: [w1531] -> _
    shift-left: _ -> [w1530]
    i -> [w1534]
    stop <- w1544 stop-if-true
    # "cam"
    n755 = Preview Queue Element(queue=w1556, timeout in ms (-1)=w1543) -> (queue out=w1555:refnum<queue>, element=w1554:string)  [unwired: 1 in, 2 out]
    n756 = Match Pattern(string=w1554, regular expression=":") -> (before substring=w1551:string, after substring=w1552:string)  [unwired: 1 in, 2 out]
    n757 = case shown="\"idle\", Default" w1551 {
      tunnel: w1555 -> [w1568 w1600 w1633 w1646 _ w1734 w1764 w1829]
      tunnel: w1552 -> [_ _ _ _ _ _ _ _]
      tunnel: [w1562 w1587 w1632 w1644 w1687 w1731 w1749 w1827] -> w1550
      tunnel: w1549 -> [_ _ w1632 w1644 w1687 w1731 w1749 w1827]
      tunnel: [w1567 w1601 u64 0 ("Hout") w1643 w1691 w1732 w1759 w1826] -> w1548
      tunnel: [w1569 w1602 w1629 w1642 w1692 w1733 w1750 w1825] -> w1547
      tunnel: w1546 -> [_ w1604 w1631 w1643 w1694 w1736 w1761 w1826]
      tunnel: w1545 -> [_ w1603 _ w1642 w1693 w1735 w1760 w1825]
      tunnel: [_ _ _ TRUE _ _ _ _] -> w1544
      tunnel: [_ _ -1 _ _ _ _ -1] -> w1542
      tunnel: [w1561 w1588 _ _ w1701 _ _ _] -> w1541
      tunnel: w1540 -> [w1561 w1588 _ _ w1700 _ _ _]
      tunnel: [w1562 w1590 w1627 w1641 w1696 w1725 w1762 w1824] -> w1539
      tunnel: w1538 -> [_ w1590 w1627 w1641 w1696 _ w1762 w1824]
      tunnel: w1537 -> [_ _ _ _ _ _ w1753 _]
      tunnel: [w1559 w1585 w1626 w1639 w1654 w1722 w1756 w1823] -> w1536
      tunnel: w1535 -> [w1559 w1585 w1626 w1639 w1689 w1722 w1756 w1823]
      tunnel: w1534 -> [_ _ _ _ w1662 _ _ _]
      tunnel: [w1560 w1586 w1625 w1640 w1688 w1721 w1755 w1822] -> w1533
      tunnel: w1532 -> [w1560 w1586 w1625 w1640 w1661 w1721 w1755 w1822]
      tunnel: [w1558 w1582 refnum<k21> refnum ("task out") w1638 w1647 w1720 w1746 w1821] -> w1531
      tunnel: w1530 -> [_ w1582 w1624 w1638 w1647 w1720 w1747 w1821]
      frame "init" {
        w1562 = u16[][] []
        n758 = flat-sequence {
          tunnel: [w1571] -> w1566
          tunnel: [w1572] -> w1565
          tunnel: [w1580] -> w1567
          tunnel: [w1581] -> w1569
          tunnel: w1566 -> [w1581]
          tunnel: w1565 -> [w1580]
          frame #0 {
            n759 = local write "cam_con?"(FALSE ("cam_con?")) -> ()
          }
          frame #1 {
            n760 = call "SCInitBoard.vi"("boardnr"="board number") -> ("Hout"=w1575:u32, "error out"=w1576:errorcluster)  [unwired: 1 in, 1 out]
            n761 = call "SCSetupCamera.vi"("Handle"=w1575, "error in (no error)"=w1576) -> ("Hout"=w1577:u64, "error out"=w1578:errorcluster)  [unwired: 1 out]
            n762 = call "SCStopCOC.vi"("error in (no error)"=w1578, "Stop mode"=0, "Handle"=w1577) -> ("error out"=w1571:errorcluster, "Hout"=w1572:u64)
          }
          frame #2 {
            n763 = local write "cam_con?"(TRUE ("cam_con?")) -> ()
          }
        }
        n764 = Dequeue Element(queue=w1568) -> (queue out=w1564:refnum<queue>)  [unwired: 2 in, 3 out]
        n765 = Enqueue Element At Opposite End(queue=w1564, element="set") -> ()  [unwired: 2 in, 3 out]
        n766 = call-poly <vilib>:"DAQmx Create Virtual Channel.vi"("lines"=tag "Dev3/port0/line0") -> ("task out"=w1558:refnum<k21>)  [unwired: 13 in, 1 out]
      }
      frame "set" {
        n767 = Dequeue Element(queue=w1600) -> ()  [unwired: 2 in, 4 out]
        n768 = call "SCStopCOC.vi"("error in (no error)"=w1603, "Stop mode"=0, "Handle"=w1604) -> ("error out"=w1619:errorcluster, "Hout"=w1618:u64)
        n769 = Bundle By Name(cluster=cluster{"Delay":dbl, "Exposure ":dbl} {"Delay"=0.0, "Exposure "=0.0} ("Delay and exposure"), "Exposure"="cam_exp") -> (w1597:cluster{"Delay":dbl, "Exposure ":dbl})
        n770 = Bundle By Name(cluster=T11 {"Camera type"=0, "Operating mode\nHP & QE / HS & DiCam Pro "=0, "Frame trigger \n(High Performance and QE only)"=0, "Sequence trigger"=0, "Low Light\n(QE only)"=FALSE, "Gain"=FALSE, "Horzontal\nbinning"=0, "Vertical\nbinning "=0, "ROI Left"=1, "ROI Right"=20, "ROI Top"=1, "ROI Bottom"=15} ("Camera controls"), "Operating mode\nHP & QE / HS & DiCam Pro"="Operating mode\nHP & QE / HS & DiCam Pro", "Horzontal\nbinning"="binning", "Vertical\nbinning"="binning", "ROI Left"="ROI Left", "ROI Right"="ROI Right", "ROI Top"="ROI Top", "ROI Bottom"="ROI Bottom", "Gain"="gain", "Frame trigger \n(High Performance and QE only)"="Frame trigger \n(High Performance and QE only)") -> (w1614:T11)
        n771 = call "New delay and exposure forma.vi"("Operating mode\nHP & QE / HS & DiCam Pro"="Operating mode\nHP & QE / HS & DiCam Pro", "Delay and exposure"=w1597) -> ("Output table"=w1615:string)  [unwired: 3 in]
        n772 = call "SCSetCoC.vi"("error in (no error)"=w1619, "Delay and exposure table"=w1615, "Camera controls"=w1614, "Handle"=w1618) -> ("error out"=w1607:errorcluster, "Hout"=w1606:u64)  [unwired: 1 out]
        n773 = call "SCGetImageSize.vi"("Handle"=w1606, "error in (no error)"=w1607) -> ("Hout"=w1605:u64, "error out"=w1589:errorcluster, "Horizontal size"=w1594:i32, "Vertical size"=w1593:i32)  [unwired: 2 out]
        n774 = Greater?(x=w1594, y=w1593) -> (0:w1595:bool)
        n775 = Initialize Array(u16 0 ("dimension size"), w1593, w1594) -> (w1587:u16[][])
        n776 = call "SCRun.vi"("error in (no error)"=w1589, "Run mode"=0, "Handle"=w1605) -> ("error out"=w1602:errorcluster, "Hout"=w1601:u64)  [unwired: 1 out]
        n777 = Select(t=w1594, s=w1595, f=w1593) -> (s? t:f=w1592:i32)
        n778 = property on="mainimg" class="IntGraph (strict)"("XScale.Maximum"=w1592, "YScale.Maximum"=w1592) -> ()  [unwired: 2 in, 2 out]
      }
      frame "release" {
        n779 = Dequeue Element(queue=w1633) -> (queue out=w1620:refnum<queue>)  [unwired: 2 in, 3 out]
        n780 = flat-sequence {
          tunnel: w1631 -> [w1635]
          tunnel: [w1634] -> w1628
          tunnel: [w1637] -> w1629
          tunnel: w1628 -> [w1637]
          frame #0 {
            n781 = call "SCCloseBoard.vi"("Handle"=w1635) -> ("error out"=w1634:errorcluster)  [unwired: 1 in, 2 out]
          }
          frame #1 {
            n782 = local write "cam_con?"(FALSE ("cam_con?")) -> ()
          }
        }
        n783 = Enqueue Element(queue=w1620, element="suspend") -> ()  [unwired: 2 in, 3 out]
        n784 = call <vilib>:"DAQmx Clear Task.vi"("task in"=w1624) -> ()  [unwired: 14 in, 1 out]
      }
      frame "close" {
        n785 = Release Queue(queue=w1646) -> ()  [unwired: 2 in, 3 out]
      }
      frame "idle", Default {
        n786 = call "grabimg.vi"("array in"=w1687, "error in"=w1693, "Hin"=w1694) -> ("error out"=w1692:errorcluster, "imgdata"=w1690:i32[][], "Hout"=w1691:u64)  [unwired: 6 in]
        n787 = local read "lower threshold"() -> (w1685:i32)
        n788 = case shown="True" "cam_dark?" {
          tunnel: w1696 -> [_ w1719]
          tunnel: [w1716 w1718] -> w1686
          tunnel: w1690 -> [w1716 w1717]
          frame False {
          }
          frame True {
            n789 = Subtract(x=w1717, y=w1719) -> (x-y=w1718:dbl[][])
          }
        }
        n790 = call "filtr_b.vi"("threshold"=w1685, "input array"=w1686) -> ("output array"=w1677:dbl[][])  [unwired: 9 in]
        n791 = call <vilib>:"High Resolution Relative Seconds.vi"() -> ("relative seconds"=w1701:dbl)
        n792 = Subtract(x=w1701, y=w1700) -> (x-y=w1699:dbl)
        n793 = Array Size(array=w1677) -> (size(s)=w1676:i32[])
        n794 = Reciprocal(x=w1699) -> (1/x=→"cam_fps":dbl)
        n795 = Index Array(array=w1676) -> (element #1=w1671:i32, element #2=w1670:i32)  [unwired: 2 in]
        n796 = Subtract(x=w1662, y=w1661) -> (x-y=w1660:i32)
        n797 = Less Or Equal?(x="pics2avg", y=w1660) -> (x <= y?=w1683:bool)
        n798 = And(x="reset every n pics", y=w1683) -> (x .and. y?=w1681:bool)
        n799 = Not(x=w1681) -> (.not. x?=w1680:bool)
        n800 = call-poly <vilib>:"Ramp Pattern.vi"("start"=0.0, "end"=w1671, "samples"=w1671) -> ("Ramp Pattern"=w1666:dbl[])  [unwired: 7 in, 1 out]
        n801 = call-poly <vilib>:"Ramp Pattern.vi"("start"=0.0, "end"=w1670, "samples"=w1670) -> ("Ramp Pattern"=w1667:dbl[])  [unwired: 7 in, 1 out]
        n802 = property on="mainimg" class="IntGraph (strict)"() -> ("CrsrLis"=w1659:T5)  [unwired: 2 in, 2 out]
        n803 = And(x="cam_liveavg", y=w1680) -> (x .and. y?=w1678:bool)
        n804 = case shown="False" w1678 {
          tunnel: w1677 -> [w1706 w1712]
          tunnel: [w1706 w1709] -> w1654
          tunnel: w1689 -> [_ w1714]
          tunnel: w1662 -> [w1707 _]
          tunnel: [w1707 w1715] -> w1688
          tunnel: w1661 -> [_ w1715]
          tunnel: w1660 -> [_ w1708]
          frame False {
          }
          frame True {
            n805 = Multiply(x=w1714, y=w1708) -> (x*y=w1713:dbl[][])
            n806 = Increment(x=w1708) -> (x+1=w1710:i32)
            n807 = Add(x=w1713, y=w1712) -> (x+y=w1711:dbl[][])
            n808 = Divide(x=w1711, y=w1710) -> (x/y=w1709:dbl[][])
          }
        }
        "mainimg" <- w1654
        n809 = Index Array(array=w1659) -> (element #1=w1657:T12, element #2=w1658:T12)  [unwired: 2 in]
        n810 = Unbundle By Name(w1657) -> ("Position.X"=w1651:dbl, "Position.Y"=w1653:dbl)
        n811 = Unbundle By Name(w1658) -> ("Position.X"=w1655:dbl, "Position.Y"=w1656:dbl)
        n812 = Array Max & Min(array=w1654) -> (max value=→"max":dbl)  [unwired: 3 out]
        n813 = Subtract(x=w1656, y=w1653) -> (x-y=w1652:dbl)
        n814 = Subtract(x=w1655, y=w1651) -> (x-y=w1650:dbl)
        n815 = Array Subset(array=w1654, index (row)=w1653, length (row)=w1652) -> (w1665:dbl[][])  [unwired: 2 in]
        n816 = Array Subset(array=w1654, index (col)=w1651, length (col)=w1650) -> (w1663:dbl[][])  [unwired: 2 in]
        n817 = Array Subset(array=w1654, index (row)=w1653, length (row)=w1652, index (col)=w1651, length (col)=w1650) -> (w1649:dbl[][])
        n818 = Transpose 2D Array(2D array=w1665) -> (transposed array=w1664:dbl[][])
        n819 = Add Array Elements(numeric array=w1649) -> (sum=→"sum" →"Waveform Chart":dbl)
        n820 = for {
          tunnel: w1663 -> [w1703] mode=indexing
          tunnel: [w1702] -> w1673 mode=indexing
          n821 = Add Array Elements(numeric array=w1703) -> (sum=w1702:dbl)
        }
        n822 = for {
          tunnel: w1664 -> [w1705] mode=indexing
          tunnel: [w1704] -> w1672 mode=indexing
          n823 = Add Array Elements(numeric array=w1705) -> (sum=w1704:dbl)
        }
        n824 = Bundle("Ramp Pattern"=w1667, w1672) -> (→"G2 X":cluster{"Ramp Pattern":dbl[], dbl[]})  [unwired: 1 in]
        n825 = Bundle(w1673, "Ramp Pattern"=w1666) -> (→"G2 Y":cluster{dbl[], "Ramp Pattern":dbl[]})  [unwired: 1 in]
      }
      frame "dark" {
        n826 = Dequeue Element(queue=w1734) -> ()  [unwired: 2 in, 4 out]
        n827 = Array Size(array=w1731) -> (size(s)=w1730:i32[])
        n828 = Index Array(array=w1730) -> (element #1=w1729:i32, element #2=w1728:i32)  [unwired: 2 in]
        n829 = Initialize Array(0.0 ("element"), w1729, w1728) -> (w1726:dbl[][])
        n830 = for {
          N: "dark avg" -> [_]
          tunnel: w1736 -> [w1744]
          tunnel: w1735 -> [w1743]
          tunnel: [w1742] -> w1733
          tunnel: w1731 -> [w1741]
          tunnel: [w1740] -> w1732
          shift-right: [w1737] -> w1724
          shift-left: w1726 -> [w1738]
          n831 = call "grabimg.vi"("array in"=w1741, "error in"=w1743, "Hin"=w1744) -> ("error out"=w1742:errorcluster, "imgdata"=w1739:i32[][], "Hout"=w1740:u64)  [unwired: 6 in]
          n832 = Add(x=w1739, y=w1738) -> (x+y=w1737:dbl[][])
        }
        n833 = Divide(x=w1724, y="dark avg") -> (x/y=w1725:dbl[][])
      }
      frame "snap" {
        n834 = Dequeue Element(queue=w1764) -> ()  [unwired: 2 in, 4 out]
        n835 = local read "cam_dark?"() -> (w1763:bool)
        n836 = local read "cam_avgs"() -> (w1758:i32)
        n837 = To Double Precision Float(number=w1749) -> (double precision float=w1748:dbl[][])
        n838 = Equal To 0?(x="aq.mode") -> (x = 0?=w1751:bool)
        n839 = Get Date/Time In Seconds() -> (seconds since 1Jan1904=w1754:timestamp)
        n840 = for {
          N: w1758 -> [w1776]
          shift-right: [w1793] -> w1759
          shift-left: w1761 -> [w1795]
          shift-right: [w1781] -> w1757
          shift-left: w1760 -> [w1794]
          tunnel: w1763 -> [w1791]
          tunnel: w1762 -> [w1790]
          tunnel: w1749 -> [w1789]
          tunnel: w1754 -> [w1785]
          tunnel: w1751 -> [w1769]
          shift-right: [w1777] -> w1745
          shift-left: w1748 -> [w1778]
          shift-right: [w1767] -> w1746
          shift-left: w1747 -> [w1767]
          i -> [w1765]
          stop <- "abort acq." stop-if-true
          n841 = call "grabimg.vi"("array in"=w1789, "error in"=w1794, "Hin"=w1795) -> ("error out"=w1781:errorcluster, "imgdata"=w1792:i32[][], "Hout"=w1793:u64)  [unwired: 6 in]
          n842 = local read "lower threshold"() -> (w1772:i32)
          n843 = Increment(x=w1765) -> (x+1=w1774:i32)
          "acq. imgs" <- w1774
          n844 = Get Date/Time In Seconds() -> (seconds since 1Jan1904=w1788:timestamp)
          n845 = case shown="True" w1791 {
            tunnel: w1792 -> [w1817 w1820]
            tunnel: w1790 -> [_ w1819]
            tunnel: [w1817 w1818] -> w1771
            frame False {
            }
            frame True {
              n846 = Subtract(x=w1820, y=w1819) -> (x-y=w1818:dbl[][])
            }
          }
          n847 = Divide(x=w1774, y=w1776) -> (x/y=→"snap_prog":dbl)
          n848 = Subtract(x=w1788, y=w1785) -> (x-y=w1787:dbl)
          n849 = call "filtr_b.vi"("threshold"=w1772, "input array"=w1771) -> ("output array"=w1770:dbl[][])  [unwired: 9 in]
          n850 = Divide(x=w1787, y=w1765) -> (x/y=w1783:dbl)
          n851 = Multiply(x=w1783, y=w1776) -> (x*y=w1786:dbl)
          n852 = Reciprocal(x=w1783) -> (1/x=w1782:dbl)
          n853 = case shown="True" "count?" {
            tunnel: w1770 -> [w1808 w1810]
            tunnel: "e-size" -> [_ w1812]
            tunnel: w1772 -> [_ w1811]
            tunnel: [w1808 w1809] -> w1768
            frame False {
            }
            frame True {
              n854 = Array Size(array=w1810) -> (size(s)=w1814:i32[])
              n855 = call "findr.vi"("thresh"=w1811, "esize"=w1812, "inp array"=w1810) -> ("locs"=w1813:i32[][])  [unwired: 8 in]
              n856 = Index Array(array=w1814) -> (element #1=w1816:i32, element #2=w1815:i32)  [unwired: 2 in]
              n857 = call "drawe.vi"("Ysize"=w1816, "Xsize"=w1815, "pos array"=w1813) -> ("img out"=w1809:i32[][])  [unwired: 8 in]
            }
          }
          n858 = Add(x=w1786, y=w1785) -> (x+y=→"ETA":timestamp)
          n859 = local write "cam_fps"(w1782) -> ()
          n860 = local write "mainimg"(w1770) -> ()
          n861 = case shown="True" w1769 {
            tunnel: w1768 -> [w1798 w1806]
            tunnel: w1778 -> [w1800 w1805]
            tunnel: [w1799 w1803] -> w1777
            tunnel: [w1797 w1802] -> w1766
            tunnel: w1765 -> [w1796 w1801]
            frame False {
              n862 = Add(x=w1798, y=w1800) -> (x+y=w1799:dbl[][])
              n863 = Increment(x=w1796) -> (x+1=w1797:i32)
            }
            frame True {
              n864 = Multiply(x=w1805, y=w1801) -> (x*y=w1807:dbl[][])
              n865 = Increment(x=w1801) -> (x+1=w1802:i32)
              n866 = Add(x=w1806, y=w1807) -> (x+y=w1804:dbl[][])
              n867 = Divide(x=w1804, y=w1802) -> (x/y=w1803:dbl[][])
            }
          }
          "Pics L" <- w1766
          n868 = local write "sideimg"(w1777) -> ()
        }
        n869 = Enqueue Element(queue=w1753, element=w1745, error in (no error)=w1757) -> (error out=w1750:errorcluster)  [unwired: 1 in, 2 out]
      }
      frame "suspend" {
        n870 = Dequeue Element(queue=w1829) -> ()  [unwired: 2 in, 4 out]
      }
    }
    "cam_error" <- w1547
  }
